vi "COD主界面（列队使用）.vi"() -> (8 "多列列表框":i32(listbox))   [LabVIEW 2016, in "斯坦道CODMn.lvlib"]
uses:
  <vilib>/Analysis/6fits.llb/Curve Fitting Criteria.ctl
  <vilib>/Utility/miscctls.llb/LVPointTypeDef.ctl
  <vilib>/Utility/config.llb/Read Key (I32).vi
  <vilib>/Utility/config.llb/Read Key (Double).vi
  <vilib>/Utility/config.llb/Read Key (Boolean).vi
  <vilib>/Utility/config.llb/Write Key (I32).vi
  <vilib>/Utility/config.llb/Write Key (Double).vi
  <vilib>/Utility/config.llb/Write Key (Boolean).vi
  <vilib>/Waveform/WDTFileIO.llb/Read Waveform from File.vi
  <vilib>/ptbypt/NI_PtbyPt.lvlib
  <vilib>/Utility/config.llb/NI_LVConfig.lvlib
  <vilib>/Analysis/NI_AALPro.lvlib
panel:
  in  "加标回收量程：":enum32{"H", "L", "AUTO"}(ring)=enum."AUTO"
  in  "定时设置":cluster{"启动":bool, "控制命令":T1, "测量参数":T2}(xcontrol)
  out "氢氧化钠":dbl
  in  "序列号变更":bool
  out "模块版本号":string
  in  "更新程序":bool
  out "进样无液体告警":bool
  out "校准内容显示":string
  out "60分钟超时报警":bool
  in  "远程校准量程":enum16{"L", "H"}(ring)
  in  "远程自动校准浓度":dbl
  in  "仪器参数":bool
  out "CODMn序列号":string
  out "CODMn软件版本：":string
  in  "标样核查量程选择":enum32{"H", "L", "AUTO"}(ring)=enum."AUTO"
  in  "标样浓度":dbl
  in  "零点核查量程选择":enum32{"H", "L", "AUTO"}(ring)=enum."AUTO"
  in  "零点核查浓度":dbl
  out "序列号":string
  in  "采水泵排液时间/s:":i32
  in  "采水泵润洗时间/s:":i32
  in  "采水泵沉淀时间/s:":i32
  in  "采水泵进样时间/s:":i32
  in  "常规版/认证版":enum16{"常规版-酸性", "常规版-碱性", "认证版", "浮台版"}(ring)
  in  "释放串口":bool
  in  "打开串口":bool
  in  "保存参数":dbl[](array[numeric])
  out "报警数字":i16
  out "CODMn工作状态":T3(ring)
  out "ORP-K":string
  out "ORP-B":string
  out "ORP-A":string
  out "x = y?":bool
  out "稀释倍数解释":string
  in  "跨度量程选择":enum32{"H", "L", "AUTO"}(ring)=enum."AUTO"
  in  "跨度液浓度":dbl
  in  "水样：":dbl
  in  "蒸馏水：":dbl
  in  "标液：":dbl
  in  "零点核查样：":dbl
  in  "加标回收样：":dbl
  in  "草酸钠":dbl
  in  "高锰酸钾":dbl
  in  "硫酸":dbl
  out "量程解释说明":string
  in  "高切低阈值:":dbl
  in  "低切高阈值:":dbl
  in  "水样量程选择:":enum16{"L", "H", "自动切换测一次", "自动切换测两次"}(ring)
  in  "氢氧化钠：":dbl
  in  "标准液浓度":dbl
  in  "温度":dbl
  in  "恒温时间":dbl
  in  "当前量程：":enum16{"L", "H"}(ring)
  in  "CODMn零点核查选择":enum16{"零点核查走纯水管", "零点核查走零漂管"}(ring)
  in  "锁定按钮":bool
  in  "低量程稀释倍数:":i8=1
  in  "高量程稀释倍数:":i8=2
  in  "一键写入":bool
  in  "测量模式(公式)":u16(ring)=1 items=["水样测试"=1, "标样核查"=2, "零点核查"=3, "跨度核查"=4, "空白测试"=5, "平行样"=6, "加标回收"=7]
  out "基本量程(显示)":string
  out "测量模式(显示)":string
  out "数据时间":string
  out "断电排液标记":bool
  out "COM":string
  in  "启用5":bool
  in  "校准5":bool
  in  "泵滴定数5":dbl
  in  "浓度5":dbl
  in  "启用4":bool
  in  "校准4":bool
  in  "泵滴定数4":dbl
  in  "浓度4":dbl
  out "波形时间":timestamp
  in  "历史波形":bool
  out "滴定数-ORP值":u16[](array[numeric]) caption="数组"
  in  "关闭 3":bool
  in  "滴定曲线":bool
  out "ORP滴定曲线":u16[](graph)
  out "空白测试标记":bool
  out "跨度核查标记":bool
  in  "量程选择":enum16{"低量程", "高量程", "0-2量程"}(ring)
  in  "手动控制":bool
  in  "选用水样":enum16{"葡萄糖", "草酸钠"}(ring)
  in  "方程系数":cluster{"K":dbl, "b":dbl, "X^2":dbl} {"X^2" format="%#.6g"; "b" format="%#.6g"; "K" format="%#.6g"}
  out "多项式系数":dbl[](array[numeric])
  out "XY图":cluster{"X Values":dbl[], "Y Values":dbl[]}[](graph)
  in  "模型":enum32{"线性", "多项式"}(ring)
  out "启动时间":timestamp format="%<%Y/%m/%d %H:%M:%S>T"
  in  "关闭 2":bool
  out "r^2":dbl format="%.8g"
  out "拟合公式":string
  out "b":dbl format="%#.4g"
  out "K":dbl format="%#.4f"
  in  "启用3":bool
  in  "启用2":bool
  in  "启用1":bool
  in  "校准3":bool
  in  "校准2":bool
  in  "校准1":bool
  in  "泵滴定数3":dbl
  in  "泵滴定数2":dbl
  in  "泵滴定数1":dbl
  in  "浓度3":dbl
  in  "浓度2":dbl
  in  "浓度1":dbl
  in  "写入":bool
  out "零点核查标记":bool
  out "排液故障":bool
  out "进水样超量程":bool
  out "标样核查标记":bool
  out "平行样测量":bool
  out "加标回收测量":bool
  out "质控样测量":bool
  out "待机":bool
  out "校标错误":bool
  out "校零错误":bool
  out "测量错误":bool
  out "草酸钠报警":bool
  out "高锰酸钾报警":bool
  out "加热故障":bool
  out "温控器故障":bool
  out "ORP故障":bool
  out "排液标记":bool
  out "故障标记":bool
  out "校标标记":bool
  out "校零标记":bool
  out "通讯状态":bool
  out "水样测量":bool
  in  "读取":bool
  in  "返回":bool
  in  "校准配置":bool
  in  "零点泵计量数 2":dbl
  in  "标度泵计量数 2":dbl
  out "标度滴定值":dbl
  out "零点滴定值":dbl
  in  "保存":bool
  in  "关闭":bool
  out "仪器时间":timestamp format="%<%Y/%m/%d %H:%M:%S>T"
  out "秒":u16
  out "分":u16
  out "COD浓度（mg/L)":dbl format="%.2g"
  out "进样管":dbl
  out "高锰酸钾":dbl
  out "草酸钠":dbl
  out "硫酸":dbl
  out "实时ORP":dbl
  out "温度℃":dbl
  out "加热":bool
  out "搅拌":bool
  out "进硫酸":bool
  out "进加标回收样":bool
  out "进零点核查样":bool
  out "进标液":bool
  out "进蒸馏水":bool
  out "进水样":bool
  out "进草酸钠":bool
  out "进高锰酸钾":bool
  in  "启动":bool
  in  "故障清除":bool
  in  "参数配置":bool
  in  "停止":bool
  in  "单步启动":bool
  out "系统时间":timestamp
  in  "时间校准":bool
  out "模式（受控）":u16
  # "测试时长："
  # "注：遇到加热故障和排液故障时仪器不能正常启动，\n必须排查故障并点击报警清除按钮方可运行。"
  # "mg/L"
  # "基本参数设置"
  # "校零校标结果"
  # "泵计量参数设置"
  # "校零结果："
  # "校零滴定值："
  # "高锰酸钾："
  # "加热恒温温度(℃):"
  # "草酸钠："
  # "校标结果："
  # "标度滴定值："
  # "恒温时间(分钟):"
  # "零点泵计量值："
  # "硫酸："
  # "标准液浓度(mg/L):"
  # "标度泵计量值："
  # "跨度核查浓度："
  # "跨度核查量程："
  # "零点核查浓度："
  # "标样浓度："
  # "零点核查量程："
  # "标样核查量程："
  # "远程校准配置区"
  # "公式读取写入区"
  # "mg/L"
  # "是否启用"
  # "泵滴定数"
  # "浓度"
  # "辅\n助\n计\n算\n区"
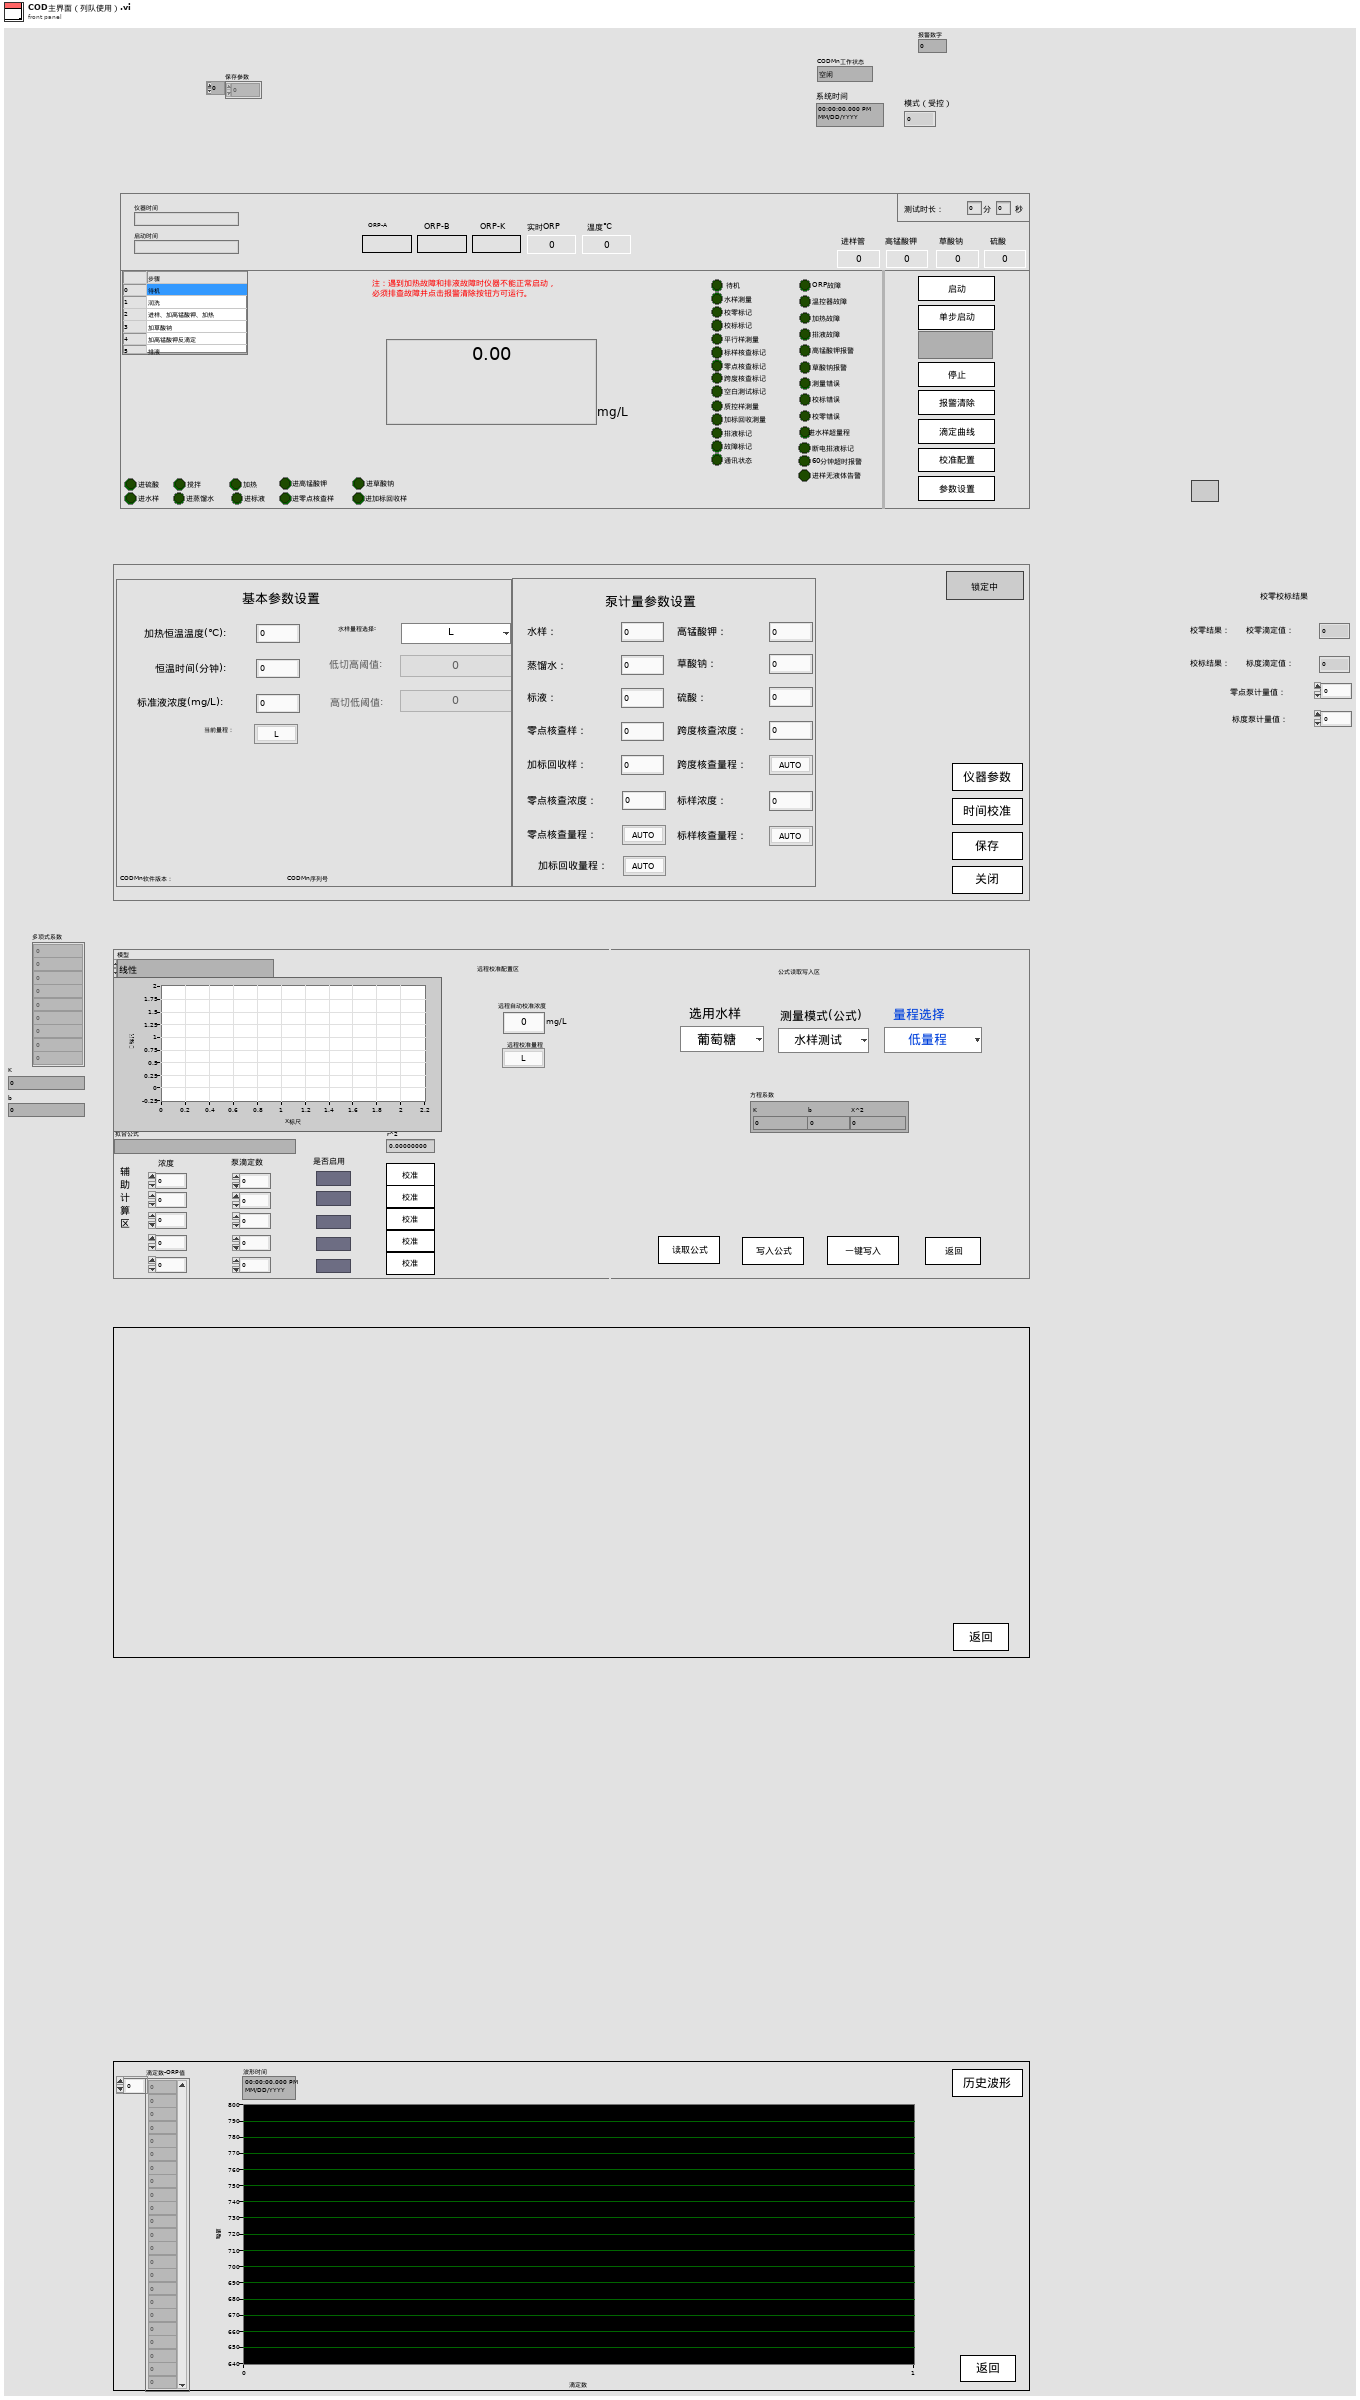
[diagram p1: front panel]
types:
  T1 = typedef "定时设置.xctl/国标控制命令.ctl" = enum16{"启动测量", "标样核查", "零点核查", "跨度核查", "空白测试", "平行样测试", "加标回收", "空白校准", "标样校准", "初始化（清洗）", "停止测试", "仪器重启", "校时", "模式设置", "测量间隔设置"}
  T2 = typedef "定时设置.xctl/测量参数.ctl" = u16
  T3 = enum16{"空闲", "水样测试", "标样核查", "零点核查", "跨度核查", "空白测试", "平行样测试", "质控样", "空白校准", "标样校准", "加标回收"}
  T4 = typedef "LVPointTypeDef.ctl" = cluster{"Horizontal":i16, "Vertical":i16}
  T5 = cluster{"Major":u16, "Minor":u16, "Fix":u16, "Build":u16}
  T6 = typedef "NI_LVConfig.lvlib/Config Data RefNum.ctl" = refnum<k1>
  T7 = cluster{"时间源选择":enum16{"系统时间源", "仪器时间源"}, "外部时间源":timestamp}
  T8 = enum32{"Bad", "Idle", "Run top level", "Running"}
  T9 = enum8{"Enabled", "Disabled", "Disabled and Grayed Out"}
  T10 = cluster{"时间":timestamp, "测量模式":string, "数据类型":string, "检测值":sgl, "单位":string, "数据标识":string, "因子编码":string, "标样参考值":sgl, "ORP-A":sgl, "ORP-B":sgl, "ORP-K":sgl, "COD滴定值":sgl, "高锰酸钾滴定数":sgl, "温度":sgl, "量程":sgl, "LastTime":timestamp, "序列号:":string}
  T11 = cluster{"因子编码":u32, "单位":u16, "标样参考值":sgl, "水样数据时间":timestamp, "水样实测值":sgl, "水样数据标识":string, "标样数据时间":timestamp, "标样实测值":sgl, "标样数据标识":string, "空白数据时间":timestamp, "空白实测值":sgl, "空白数据标识":string, "零点核查数据时间":timestamp, "零点核查实测值":sgl, "零点核查数据标识":string, "跨度核查数据时间":timestamp, "跨度核查实测值":sgl, "跨度核查数据标识":string, "加标回收数据时间":timestamp, "加标回收实测值":sgl, "加标回收数据标识":string, "平行样数据时间":timestamp, "平行样实测值":sgl, "平行样数据标识":string}
  T12 = cluster{"数组 2[0]":sgl, "数组 2[1]":sgl, "数组 2[2]":sgl, "数组 2[3]":sgl, "数组 2[4]":sgl, "数组 2[5]":sgl, "数组 2[6]":sgl, "数组 2[7]":sgl, "数组 2[8]":sgl, "数组 2[9]":sgl, "数组 2[10]":sgl, "数组 2[11]":sgl, "数组 2[12]":sgl, "数组 2[13]":sgl, "数组 2[14]":sgl, "数组 2[15]":sgl, "数组 2[16]":sgl, "数组 2[17]":sgl, "数组 2[18]":sgl, "数组 2[19]":sgl, "数组 2[20]":sgl, "数组 2[21]":sgl, "数组 2[22]":sgl, "数组 2[23]":sgl, "数组 2[24]":sgl, "数组 2[25]":sgl, "数组 2[26]":sgl, "数组 2[27]":sgl, "数组 2[28]":sgl, "数组 2[29]":sgl, "数组 2[30]":sgl, "数组 2[31]":sgl, "数组 2[32]":sgl, "数组 2[33]":sgl, "数组 2[34]":sgl, "数组 2[35]":sgl, "数组 2[36]":sgl, "数组 2[37]":sgl, "数组 2[38]":sgl, "数组 2[39]":sgl, "数组 2[40]":sgl, "数组 2[41]":sgl}
  T13 = cluster{"ORP故障":bool, "温控器故障":bool, "加热故障":bool, "高锰酸钾报警":bool, "草酸钠报警":bool, "测量错误":bool, "校零错误":bool, "校标错误":bool, " 进水样超量程":bool, "排液阀故障":bool, "60分钟超时报警":bool, "进样无液体报警":bool}
  T14 = cluster{"时间标识":timestamp, "参数":string, "日志信息":string, "流程参数":string}
  T15 = cluster{"测量量程":dbl, "测量精度":dbl, "测量间隔":dbl, "消解温度":dbl, "消解时长":dbl, "空白校准时间":timestamp, "曲线截距":dbl, "曲线斜率":dbl, "测量检出限":dbl, "测量信号值":dbl, "线性相关系数":dbl, "二次多项式系数":dbl, "标样校准时间":timestamp, "稀释倍数":dbl, "三项式系数":dbl, "空白标定系数":dbl, "量程系数":dbl, "F0/ORPA":dbl, "F1/ORPB":dbl, "F2/ORPK":dbl, "F3":dbl, "F4":dbl, "F5":dbl, "F6":dbl, "F7":dbl, "X0/滴定数":dbl, "量程":dbl}
  T16 = cluster{"确定":bool, "测量量程":dbl, "测量精度":dbl, "测量间隔":dbl, "消解温度":dbl, "消解时长":dbl, "空白校准时间":timestamp, "曲线截距":dbl, "曲线斜率":dbl, "测量检出限":dbl, "测量信号值":dbl, "线性相关系数":dbl, "二次多项式系数":dbl, "标样校准时间":timestamp, "稀释倍数":dbl, "三项式系数":dbl, "空白标定系数":dbl, "量程系数":dbl, "F0/ORPA":dbl, "F1/ORPB":dbl, "F2/ORPK":dbl, "F3":dbl, "F4":dbl, "F5":dbl, "F6":dbl, "F7":dbl, "X0/滴定数":dbl, "量程":dbl}
  T17 = cluster{"时间标识":timestamp, "设备":string, "日志信息":string, "流程参数":string}
  T18 = typedef "NI_AALPro.lvlib/Curve Fitting Criteria.ctl" = u16
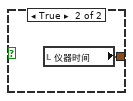
[diagram p2: hidden frame]
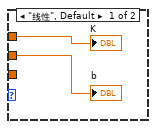
[diagram p8: hidden frame]
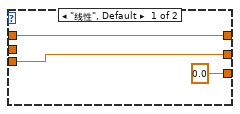
[diagram p10: hidden frame]
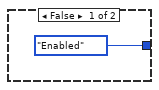
[diagram p11: hidden frame]
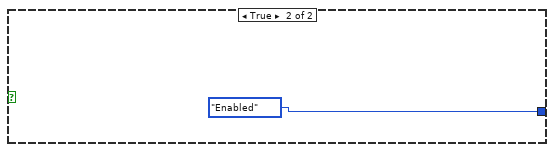
[diagram p12: hidden frame]
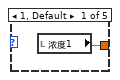
[diagram p17: hidden frame]
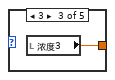
[diagram p18: hidden frame]
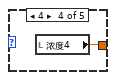
[diagram p19: hidden frame]
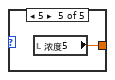
[diagram p20: hidden frame]
diagram:
  n1 = flat-sequence {
    tunnel: w3 -> [_]
    frame #0 {
      w20 = u16 1 items=["水样测试"=1, "标样核查"=2, "零点核查"=3, "跨度核查"=4, "空白测试"=5, "平行样"=6, "加标回收"=7] ("测量模式(公式)")
      n2 = vi-ref "斯坦道CODMn.lvlib:待机状态数据存储写入和切换量程(子VI).vi"() -> (w56:refnum<vi>)
      n3 = vi-ref "斯坦道CODMn.lvlib:日志报警状态存储 (子VI).vi"() -> (w49:refnum<vi>)
      n4 = vi-ref "斯坦道CODMn.lvlib:高锰酸钾-ORP滴定曲线(子VI).vi"() -> (w36:refnum<vi>)
      n5 = property class="VI"(reference=w49, error in=errorcluster {"status"=FALSE, "code"=0, "source"=""} ("错误输出")) -> ("Name"=w48:string)  [unwired: 2 out]
      n6 = property class="VI"(reference=w36, error in=errorcluster {"status"=FALSE, "code"=0, "source"=""} ("错误输出")) -> ("Name"=w37:string)  [unwired: 2 out]
      n7 = property class="VI"(reference=w56, error in=errorcluster {"status"=FALSE, "code"=0, "source"=""} ("错误输出")) -> ("Name"=w55:string)  [unwired: 2 out]
      n8 = Open VI Reference(type specifier VI Refnum (for type only)=refnum<vi> refnum, vi path=w48, options=128 ("选项")) -> (vi reference=w32:refnum<vi>, error out=w46:errorcluster)  [unwired: 3 in]
      n9 = Open VI Reference(type specifier VI Refnum (for type only)=refnum<vi> refnum, vi path=w37, options=128 ("选项")) -> (vi reference=w35:refnum<vi>, error out=w39:errorcluster)  [unwired: 3 in]
      n10 = call-by-ref "?"(reference=w32, error in=w46) -> (reference out=w44:refnum<vi>, error out=w45:errorcluster)  [unwired: 12 in]
      n11 = call-by-ref "?"(reference=w35, error in=w39) -> (reference out=w41:refnum<vi>, error out=w40:errorcluster)  [unwired: 12 in]
      n12 = Open VI Reference(type specifier VI Refnum (for type only)=refnum<vi> refnum, vi path=w55, options=128 ("选项")) -> (vi reference=w30:refnum<vi>, error out=w53:errorcluster)  [unwired: 3 in]
      n13 = Close Reference(reference=w44, error in (no error)=w45) -> ()  [unwired: 1 out]
      n14 = call-by-ref "?"(reference=w30, error in=w53) -> (reference out=w51:refnum<vi>, error out=w52:errorcluster)  [unwired: 12 in]
      n15 = Close Reference(reference=w41, error in (no error)=w40) -> ()  [unwired: 1 out]
      n16 = Close Reference(reference=w51, error in (no error)=w52) -> ()  [unwired: 1 out]
      n17 = vi-ref "关键参数交互.vi"() -> (w27:refnum<vi>)
      n18 = property class="VI"(reference=w27, error in=errorcluster {"status"=FALSE, "code"=0, "source"=""} ("错误输出")) -> ("Name"=w26:string)  [unwired: 2 out]
      n19 = Open VI Reference(type specifier VI Refnum (for type only)=refnum<vi> refnum, vi path=w26, options=128 ("选项")) -> (vi reference=w28:refnum<vi>, error out=w24:errorcluster)  [unwired: 3 in]
      n20 = call-by-ref "?"(reference=w28, error in=w24, "量程选择"=enum16{"低量程", "高量程", "0-2量程"}."低量程", "测量模式(公式)"=w20, "模型"=enum32{"线性", "多项式"}."线性") -> (reference out=w22:refnum<vi>, error out=w23:errorcluster)  [unwired: 9 in]
      n21 = Close Reference(reference=w22, error in (no error)=w23) -> ()  [unwired: 1 out]
    }
  }
  n22 = property on="定时设置" class="定时设置 (严格)"("引用参数"="CODMn") -> (error out=w1:errorcluster)  [unwired: 2 in, 1 out]
  n23 = flat-sequence {
    tunnel: [w59] -> w5
    tunnel: [errorcluster {"status"=FALSE, "code"=0, "source"=""} ("错误输出")] -> w3
    tunnel: [w61] -> w4
    frame #0 {
      w83 = "192.168.1.100" ("名称")
      n24 = global write "COD内部交互全局.vi" "量程切换次数"(u8 0 ("量程切换次数")) -> ()
      n25 = global write "COD内部交互全局.vi" "切换量程连续测两次"(FALSE ("切换量程连续测两次")) -> ()
      n26 = global read "COD内部交互全局.vi" "序列号:"() -> (w90:string)
      n27 = property on="窗格" class="Pane"("Origin"=T4 {"Horizontal"=0, "Vertical"=0} ("原点")) -> ()  [unwired: 2 in, 2 out]
      n28 = Empty String/Path?(string/path=w90) -> (empty?=w58:bool)
      n29 = case shown="真" w58 {
        tunnel: w90 -> [w105 _]
        tunnel: [w104 "data\\CODMnSet.ini" ("名称或相对路径")] -> w71
        frame False {
          # "与生产用上位机交互"
          n30 = Concatenate Strings("data\\" ("字符串"), "序列号" ("字符串"), w105, "Set.ini" ("名称或相对路径")) -> (w104:string)
        }
        frame True {
        }
      }
      n31 = String To IP(1:w83) -> (0:w76:u32)
      n32 = IP To String(2:w76) -> (0:w79:string)  [unwired: 1 in]
      n33 = Not Equal?(x=w83, y=w79) -> (x != y?=w84:bool)
      n34 = Concatenate Strings("\\\\" ("字符串"), w79) -> (w78:string)
      n35 = global write "CODMN外部API.vi" "ping"(w84) -> ()
      n36 = String To Path(string=w78) -> (path=w85:path)
      n37 = Build Path(base path=w85, name or relative path=w71) -> (appended path=w80:path)
      n38 = local write "量程选择"(enum16{"低量程", "高量程", "0-2量程"}."低量程" ("量程选择")) -> ()
      n39 = local write "选用水样"(enum16{"葡萄糖", "草酸钠"}."葡萄糖" ("选用水样")) -> ()
      n40 = global write "COD内部交互全局.vi" "配置文件ini"(w71) -> ()
      n41 = case shown="真" w84 {
        tunnel: w80 -> [w95 w99]
        tunnel: [w95 w98] -> w81
        tunnel: [FALSE w97] -> w82
        frame False {
        }
        frame True {
          n42 = call <vilib>:"Check if File or Folder Exists.vi"("path"=w99) -> ("file or folder exists?"=w97:bool, "dup path"=w98:path)  [unwired: 8 in, 1 out]
        }
      }
      n43 = control-ref of="本VI"() -> (w70:refnum<vi>)
      n44 = case shown="假" w82 {
        tunnel: w81 -> [_ w103]
        tunnel: [w101 w103] -> w62
        tunnel: w71 -> [w100 _]
        frame False {
          # "本地文件地址"
          n45 = call <vilib>:"Application Directory.vi"() -> ("Application Directory"=w102:path)
          n46 = Build Path(base path=w102, name or relative path=w100) -> (appended path=w101:path)
        }
        frame True {
          # "网络共享地址"
        }
      }
      n47 = property class="VI"(reference=w70) -> ("Library.Version"=w69:T5)  [unwired: 1 in, 2 out]
      n48 = Unbundle By Name(w69) -> ("Major"=w67:u16, "Minor"=w66:u16, "Fix"=w65:u16, "Build"=w64:u16)
      n49 = Format Into String(format string="模块版本号：%d.%d.%d.%d" ("格式字符串"), w67, w66, w65, w64) -> (resulting string=→"模块版本号":string)  [unwired: 2 in, 1 out]
      n50 = global write "CODMN外部API.vi" "配置文件 path"(w62) -> ()
      n51 = call <vilib>:"Open Config Data.vi"("configuration file path"=w62) -> ("error out"=w72:errorcluster, "refnum"=w73:T6)  [unwired: 8 in, 1 out]
      n52 = vi-ref "斯坦道CODMn.lvlib:CODMn断电保存全局变量.vi"() -> (w86:refnum<vi>)
      n53 = call <userlib>:"Read Panel from INI__ogtk.vi"("error in (no error)"=w72, "VI ref"=w86, "refnum"=w73) -> ("error out"=w74:errorcluster, "refnum out"=w75:T6)  [unwired: 7 in]
      n54 = call <vilib>:"Close Config Data.vi"("error in (no error)"=w74, "refnum"=w75) -> ("error out"=w60:errorcluster)  [unwired: 8 in, 1 out]
      n55 = call <vilib>:"Clear Errors.vi"("error in (no error)"=w60) -> ("error out"=w57:errorcluster)  [unwired: 5 in, 1 out]
      n56 = Read from Text File(file (use dialog)=w62, error in=w57) -> (text=w61:string, error out=w59:errorcluster)  [unwired: 2 in, 2 out]
      "稀释倍数解释" <- "稀释倍数解释：\n稀释倍数选择1，表示不稀释\n默认低量程系数倍数1，高量程系数倍数2\n则低量程为0~8，高量程为0~16" ("稀释倍数解释")
    }
  }
  n57 = while {
    tunnel: w1 -> [_]
    stop <- FALSE stop-if-true
    n58 = Wait (ms)(milliseconds to wait=u32 500 ("等待时间（毫秒）")) -> ()  [unwired: 1 out]
    n59 = global read "COD测量模式全局.vi" "CODMn工作状态"() -> (w116:T3)
    n60 = local read "通讯状态"() -> (w110:bool)
    n61 = case shown="假" w110 {
      tunnel: [w126 w127] -> w114
      frame False {
        n62 = Get Date/Time In Seconds() -> (seconds since 1Jan1904=w126:timestamp)
      }
      frame True {
        n63 = local read "仪器时间"() -> (w127:timestamp)
      }
    }
    n64 = vi-ref "CODMn测量流程.vi"() -> (w123:refnum<vi>)
    n65 = Bundle By Name(cluster=T7 {"时间源选择"=enum."系统时间源", "外部时间源"=timestamp(0 s since 1904-01-01)} ("时间源"), "时间源选择"=enum16{"系统时间源", "仪器时间源"}."仪器时间源", "外部时间源"=w114) -> (w112:T7)
    n66 = property class="VI"(reference=w123) -> ("Exec.State"=w121:T8, "Name"=w122:string)  [unwired: 1 in, 2 out]
    n67 = Not Equal?(x=w116, y=T3."空闲") -> (x != y?=w111:bool)
    n68 = property on="定时设置" class="定时设置 (严格)"("仪器状态"=w111, "时间源"=w112) -> ()  [unwired: 2 in, 2 out]
    n69 = Unbundle By Name("定时设置") -> ("启动"=w119:bool, "控制命令"=w120:T1)
    n70 = case shown="真" w119 {
      tunnel: w122 -> [_ w130]
      tunnel: w120 -> [_ w129]
      tunnel: w121 -> [_ w128]
      frame False {
      }
      frame True {
        n71 = case shown="\"Idle\"" w128 {
          tunnel: w130 -> [_ w134]
          tunnel: w129 -> [_ w131]
          frame "Bad", Default {
          }
          frame "Idle" {
            n72 = Open VI Reference(type specifier VI Refnum (for type only)=refnum<vi> refnum, vi path=w134, options=128 ("选项")) -> (vi reference=w135:refnum<vi>, error out=w136:errorcluster)  [unwired: 3 in]
            n73 = call-by-ref "开始异步调用"(reference=w135, error in=w136, "控制命令"=w131) -> (reference out=w137:refnum<vi>, error out=w138:errorcluster)  [unwired: 11 in]
            n74 = Close Reference(reference=w137, error in (no error)=w138) -> ()  [unwired: 1 out]
          }
        }
      }
    }
  }
  n75 = Obtain Queue(name (unnamed)="CODMn" ("名称（未命名）"), element data type=cluster{"命令":string} {"命令"="启用模块"} ("元素")) -> (queue out=w15:refnum<queue>, error out=w14:errorcluster)  [unwired: 3 in, 1 out]
  n76 = while {
    tunnel: [w145] -> _
    shift-right: [w143] -> _
    shift-left: w4 -> [w142]
    tunnel: w5 -> [_]
    stop <- FALSE stop-if-true
    n77 = global read "CODMN外部API.vi" "配置文件 path"() -> (w139:path)
    n78 = Wait (ms)(milliseconds to wait=u32 1000 ("等待时间（毫秒）")) -> ()  [unwired: 1 out]
    n79 = Read from Text File(file (use dialog)=w139) -> (text=w143:string, error out=w140:errorcluster)  [unwired: 3 in, 2 out]
    n80 = Not Equal?(x=w143, y=w142) -> (x != y?=w141:bool)
    n81 = case shown="真" w141 {
      tunnel: [w147 w154] -> w145
      tunnel: w139 -> [_ w148]
      tunnel: w140 -> [w147 _]
      frame False {
      }
      frame True {
        # "文件发生改变进行更新，远端和本地都更新"
        n82 = vi-ref "斯坦道CODMn.lvlib:CODMn断电保存全局变量.vi"() -> (w149:refnum<vi>)
        n83 = call <vilib>:"Open Config Data.vi"("configuration file path"=w148) -> ("error out"=w153:errorcluster, "refnum"=w152:T6)  [unwired: 8 in, 1 out]
        n84 = call <userlib>:"Read Panel from INI__ogtk.vi"("error in (no error)"=w153, "VI ref"=w149, "refnum"=w152) -> ("error out"=w151:errorcluster, "refnum out"=w150:T6)  [unwired: 7 in]
        n85 = call <vilib>:"Close Config Data.vi"("error in (no error)"=w151, "refnum"=w150) -> ("error out"=w154:errorcluster)  [unwired: 8 in, 1 out]
      }
    }
  }
  n86 = vi-ref "CODMn通讯.vi"() -> (w6:refnum<vi>)
  n87 = while {
    tunnel: w5 -> [_]
    stop <- FALSE stop-if-true
    # "赋值循环"
    n88 = flat-sequence {
      frame #0 {
        # "测量数据区"
        n89 = global read "COD内部交互全局.vi" "data"() -> (w399:T10)
        n90 = global read "COD测量模式全局.vi" "测量模式文字实时"() -> (w385:string)
        "测量模式(显示)" <- w385
        n91 = global read "CODMn断电保存全局变量.vi" "测量数据区"() -> (w394:T11)
        n92 = Unbundle By Name(w399) -> ("时间"=w398:timestamp, "检测值"=w397:sgl, "数据标识"=w396:string)
        n93 = case shown="\"水样测试\"" w385 {
          tunnel: w394 -> [w400 w405 w410 w415 w420 w425 w430 w435 w440 w445]
          tunnel: [w400 w404 w409 w411 w419 w424 w429 w434 w436 w444] -> w395
          tunnel: w398 -> [_ w403 w408 w414 w418 w423 w428 w433 w439 w443]
          tunnel: w397 -> [_ w402 w407 w413 w417 w422 w427 w432 w438 w442]
          tunnel: w396 -> [_ w401 w406 w412 w416 w421 w426 w431 w437 w441]
          frame "", Default {
          }
          frame "水样测试" {
            n94 = Bundle By Name(cluster=w405, "水样数据时间"=w403, "水样实测值"=w402, "水样数据标识"=w401) -> (w404:T11)
          }
          frame "标样核查" {
            n95 = Bundle By Name(cluster=w410, "标样数据时间"=w408, "标样实测值"=w407, "标样数据标识"=w406) -> (w409:T11)
          }
          frame "跨度核查" {
            n96 = Bundle By Name(cluster=w415, "跨度核查数据时间"=w414, "跨度核查实测值"=w413, "跨度核查数据标识"=w412) -> (w411:T11)
          }
          frame "零点核查" {
            n97 = Bundle By Name(cluster=w420, "零点核查数据时间"=w418, "零点核查实测值"=w417, "零点核查数据标识"=w416) -> (w419:T11)
          }
          frame "空白测试" {
            n98 = Bundle By Name(cluster=w425, "空白数据时间"=w423, "空白实测值"=w422, "空白数据标识"=w421) -> (w424:T11)
          }
          frame "加标回收" {
            n99 = Bundle By Name(cluster=w430, "加标回收数据时间"=w428, "加标回收实测值"=w427, "加标回收数据标识"=w426) -> (w429:T11)
          }
          frame "平行样" {
            n100 = Bundle By Name(cluster=w435, "平行样数据时间"=w433, "平行样实测值"=w432, "平行样数据标识"=w431) -> (w434:T11)
          }
          frame "校零" {
            n101 = Bundle By Name(cluster=w440, "空白数据时间"=w439, "空白实测值"=w438, "空白数据标识"=w437) -> (w436:T11)
          }
          frame "校标" {
            n102 = Bundle By Name(cluster=w445, "标样数据时间"=w443, "标样实测值"=w442, "标样数据标识"=w441) -> (w444:T11)
          }
        }
        n103 = Unbundle By Name(w394) -> ("水样实测值"=w391:sgl)
        n104 = feedback-in #1(w394) -> ()
        n105 = feedback #1(w394) -> (w393:T11)
        n106 = global read "CODMn断电保存全局变量.vi" "水样测试量程"() -> (w387:enum16{"L", "H"})
        n107 = Unbundle By Name(w393) -> ("水样实测值"=w392:sgl)
        n108 = feedback #2(w387) -> (w388:enum16{"L", "H"})
        n109 = feedback-in #2(w387) -> ()
        n110 = Not Equal?(x=w388, y=w387) -> (x != y?=w386:bool)
        n111 = Not Equal?(x=w391, y=w392) -> (x != y?=w390:bool)
        n112 = global write "CODMn断电保存全局变量.vi" "测量数据区"(w395) -> ()
        n113 = Or(x=w390, y=w386) -> (x .or. y?=w389:bool)
        n114 = case shown="真" w389 {
          frame False {
          }
          frame True {
            # "水样值发送改变存储本地"
            n115 = call "配置文件保存.vi"() -> ()  [unwired: 12 in]
          }
        }
      }
    }
    n116 = flat-sequence {
      frame #0 {
        # "局部变量给内部交互用全局变量"
        n117 = local read "COD浓度（mg/L)"() -> (w187:dbl)
        n118 = local read "CODMn工作状态"() -> (w190:T3)
        n119 = local read "多列列表框"() -> (w188:i32)
        n120 = local read "标准液浓度"() -> (w186:dbl)
        n121 = local read "温度℃"() -> (w181:dbl)
        n122 = local read "高锰酸钾报警"() -> (w184:bool)
        n123 = local read "断电排液标记"() -> (w183:bool)
        n124 = local read "实时ORP"() -> (w180:dbl)
        n125 = local read "故障标记"() -> (w189:bool)
        n126 = local read "高锰酸钾"() -> (w182:dbl)
        n127 = local read "待机"() -> (w185:bool)
        n128 = global write "COD内部交互全局.vi" "实时温度"(w181) -> ()
        n129 = global write "运行时序全局变量.vi" "多列列表框"(w188) -> ()
        n130 = global write "COD内部交互全局.vi" "故障标记"(w189) -> ()
        n131 = global write "COD内部交互全局.vi" "ORP显示"(w180) -> ()
        n132 = global write "COD浓度全局变量.vi" "标准液浓度"(w186) -> ()
        n133 = global write "COD内部交互全局.vi" "高锰酸钾"(w182) -> ()
        n134 = global write "COD内部交互全局.vi" "待机"(w185) -> ()
        n135 = global write "COD测量模式全局.vi" "CODMn工作状态"(w190) -> ()
        n136 = global write "COD内部交互全局.vi" "高锰酸钾报警"(w184) -> ()
        n137 = global write "COD内部交互全局.vi" "断电排液标记"(w183) -> ()
        n138 = global write "COD浓度全局变量.vi" "COD浓度（mg/L)"(w187) -> ()
      }
    }
    n139 = flat-sequence {
      frame #0 {
        # "断电保存全局给局部变量"
        n140 = global read "CODMn断电保存全局变量.vi" "高切低阈值:"() -> (w459:dbl)
        n141 = global read "CODMn断电保存全局变量.vi" "低切高阈值:"() -> (w458:dbl)
        n142 = global read "CODMn断电保存全局变量.vi" "跨度液浓度"() -> (w456:dbl)
        n143 = global read "COD内部交互全局.vi" "波形时间"() -> (→"波形时间":timestamp)
        n144 = global read "CODMn断电保存全局变量.vi" "启动时间"() -> (→"启动时间":timestamp)
        n145 = global read "CODMn断电保存全局变量.vi" "标样浓度"() -> (w454:dbl)
        n146 = global read "CODMn断电保存全局变量.vi" "CODMn跨度量程选择"() -> (w460:enum32{"H", "L", "AUTO"})
        n147 = global read "CODMn断电保存全局变量.vi" "标样核查量程选择"() -> (w451:enum32{"H", "L", "AUTO"})
        n148 = global read "CODMn断电保存全局变量.vi" "零点核查量程选择"() -> (w453:enum32{"H", "L", "AUTO"})
        n149 = global read "CODMn断电保存全局变量.vi" "加标回收量程选择"() -> (w446:enum32{"H", "L", "AUTO"})
        n150 = global read "COD内部交互全局.vi" "滴定数-ORP值"() -> (→"滴定数-ORP值":u16[])
        n151 = global read "CODMn断电保存全局变量.vi" "常规版/认证版"() -> (w455:enum16{"常规版-酸性", "常规版-碱性", "认证版", "浮台版"})
        n152 = global read "CODMn断电保存全局变量.vi" "自动切换量程:"() -> (w457:enum16{"L", "H", "自动切换测一次", "自动切换测两次"})
        n153 = global read "CODMn断电保存全局变量.vi" "零点核查浓度"() -> (w452:dbl)
        n154 = global read "CODMn断电保存全局变量.vi" "测量模式(公式)"() -> (w461:u16)
        n155 = global read "COD内部交互全局.vi" "ORP滴定曲线"() -> (→"ORP滴定曲线":u16[])
        n156 = local write "高切低阈值:"(w459) -> ()
        n157 = local write "跨度液浓度"(w456) -> ()
        n158 = local write "低切高阈值:"(w458) -> ()
        n159 = local write "标样浓度"(w454) -> ()
        n160 = local write "标样核查量程选择"(w451) -> ()
        n161 = local write "水样量程选择:"(w457) -> ()
        n162 = local write "常规版/认证版"(w455) -> ()
        n163 = local write "零点核查浓度"(w452) -> ()
        n164 = local write "零点核查量程选择"(w453) -> ()
        n165 = local write "加标回收量程："(w446) -> ()
        n166 = local write "测量模式(公式)"(w461) -> ()
        n167 = local write "跨度量程选择"(w460) -> ()
      }
    }
    n168 = flat-sequence {
      frame #0 {
        # "保存参数赋值"
        n169 = Multiply(x="温度", y=10.0) -> (x*y=w165:dbl)
        n170 = Multiply(x="标准液浓度", y=100.0) -> (x*y=w162:dbl)
        n171 = Build Array(w165, "恒温时间", w162, "氢氧化钠：", "当前量程：", "水样：", "蒸馏水：", "标液：", "零点核查样：", "加标回收样：", "高锰酸钾", "草酸钠", "硫酸", "零点泵计量数 2", "标度泵计量数 2", "高量程稀释倍数:", "低量程稀释倍数:", "CODMn零点核查选择") -> (w159:dbl[])
        n172 = local write "保存参数"(w159) -> ()
      }
    }
    n173 = flat-sequence {
      frame #0 {
        # "显示量程说明"
        n174 = global read "COD内部交互全局.vi" "通讯状态"() -> (→"通讯状态":bool)
        n175 = global read "CODMn断电保存全局变量.vi" "MB通信方式选择"() -> (w462:enum16{"串口", "TCP"})
        n176 = local read "低量程稀释倍数:"() -> (w476:i8)
        n177 = local read "高量程稀释倍数:"() -> (w466:i8)
        n178 = case shown="\"TCP\"" w462 {
          tunnel: [w479 w480] -> w467
          frame "串口", Default {
            n179 = global read "CODMn断电保存全局变量.vi" "VISA resource name"() -> (w479:refnum<visa-resource-name>)
          }
          frame "TCP" {
            n180 = global read "CODMn断电保存全局变量.vi" "IP"() -> (w480:string)
          }
        }
        "COM" <- w467
        n181 = Multiply(x=w476, y=i8 8) -> (x*y=w468:i8)
        n182 = Multiply(x=w466, y=i8 8) -> (x*y=w464:i8)
        n183 = Number To Decimal String(number=w468) -> (decimal integer string=w473:string)  [unwired: 1 in]
        n184 = Number To Decimal String(number=w464) -> (decimal integer string=w471:string)  [unwired: 1 in]
        n185 = Concatenate Strings("L低量程范围:0~" ("量程解释说明"), w473, "(mg/L)\n\nH高量程范围:" ("量程解释说明"), "0" ("字符串"), "~" ("量程解释说明"), w471, "(mg/L)" ("量程解释说明")) -> (→"量程解释说明":string)
      }
    }
    n186 = flat-sequence {
      frame #0 {
        # "参数赋值（只在读取参数时候改变一次）"
        n187 = global read "COD内部交互全局.vi" "读取浮台参数显示"() -> (w192:bool)
        n188 = global read "COD内部交互全局.vi" "读取浮台参数"() -> (w191:u16[])
        n189 = global read "COD内部交互全局.vi" "读取参数显示"() -> (w193:bool)
        n190 = global read "COD内部交互全局.vi" "读取参数"() -> (w194:u16[])
        n191 = case shown="真" w192 {
          tunnel: w191 -> [_ w200]
          frame False {
          }
          frame True {
            n192 = Index Array(array=w200) -> (element #1=w199:u16, element #2=w198:u16, element #3=w197:u16, element #4=w196:u16)  [unwired: 4 in]
            n193 = global write "COD内部交互全局.vi" "读取浮台参数显示"(FALSE ("读取参数显示")) -> ()
            n194 = local write "采水泵进样时间/s:"(w199) -> ()
            n195 = local write "采水泵润洗时间/s:"(w198) -> ()
            n196 = local write "采水泵沉淀时间/s:"(w197) -> ()
            n197 = local write "采水泵排液时间/s:"(w196) -> ()
          }
        }
        n198 = case shown="真" w193 {
          tunnel: w194 -> [_ w218]
          frame False {
          }
          frame True {
            n199 = Index Array(array=w218) -> (element #1=w227:u16, element #2=w239:u16, element #3=w223:u16, element #4=w201:u16, element #5=w226:u16, element #6=w225:u16, element #7=w238:u16, element #8=w237:u16, element #9=w236:u16, element #10=w235:u16, element #11=w234:u16, element #12=w233:u16, element #13=w232:u16, element #14=w231:u16, element #15=w230:u16, element #16=w221:u16, element #17=w220:u16, element #18=w219:u16, element #19=w216:u16, element #20=w215:u16, element #21=w214:u16, element #22=w213:u16, element #23=w212:u16, element #27=w208:u16, element #28=w207:u16, element #29=w206:u16, element #30=w205:u16, element #31=w204:u16)  [unwired: 31 in, 3 out]
            n200 = global write "COD内部交互全局.vi" "读取参数显示"(FALSE ("读取参数显示")) -> ()
            n201 = local write "水样："(w225) -> ()
            n202 = local write "标液："(w237) -> ()
            n203 = local write "硫酸"(w232) -> ()
            n204 = local write "零点核查样："(w236) -> ()
            n205 = local write "加标回收样："(w235) -> ()
            n206 = local write "当前量程："(w226) -> ()
            n207 = local write "蒸馏水："(w238) -> ()
            n208 = local write "恒温时间"(w239) -> ()
            n209 = local write "高锰酸钾"(w234) -> ()
            n210 = local write "草酸钠"(w233) -> ()
            n211 = local write "零点泵计量数 2"(w231) -> ()
            n212 = local write "标度泵计量数 2"(w230) -> ()
            n213 = local write "高量程稀释倍数:"(w221) -> ()
            n214 = local write "低量程稀释倍数:"(w220) -> ()
            n215 = local write "CODMn零点核查选择"(w219) -> ()
            n216 = Build Array(w216, w215, w214, w213, w212) -> (w211:u16[])
            n217 = Build Array(w208, w207, w206, w205, w204) -> (w203:u16[])
            n218 = Divide(x=w227, y=u16 10) -> (x/y=w228:dbl)
            n219 = Divide(x=w223, y=u16 100) -> (x/y=w222:dbl)
            n220 = local write "氢氧化钠："(w201) -> ()
            n221 = local write "温度"(w228) -> ()
            n222 = local write "标准液浓度"(w222) -> ()
            n223 = call "HexToString.vi"("数组"=w203) -> ("字符串"=w202:string)  [unwired: 10 in]
            "CODMn序列号" <- w202
            "序列号" <- w202
            n224 = call "FATEK_HexToString.vi"("数组"=w211) -> ("STRING"=w210:string[])  [unwired: 10 in]
            n225 = Index Array(array=w210) -> (element=→"CODMn软件版本：":string)  [unwired: 1 in]
            n226 = global write "COD内部交互全局.vi" "序列号:"(w202) -> ()
          }
        }
      }
    }
    n227 = flat-sequence {
      frame #0 {
        # "权限隐藏和显示功能"
        n228 = local read "x = y?"() -> (w482:bool)
        n229 = property on="更新程序" class="Bool (严格)"("Visible"=w482) -> ()  [unwired: 2 in, 2 out]
        n230 = property on="释放串口" class="Bool"("Visible"=w482) -> ()  [unwired: 2 in, 2 out]
        n231 = property on="打开串口" class="Bool"("Visible"=w482) -> ()  [unwired: 2 in, 2 out]
        n232 = property on="序列号变更" class="Bool"("Visible"=w482) -> ()  [unwired: 2 in, 2 out]
        n233 = property on="常规版/认证版" class="Enum (严格)"("Visible"=w482) -> ()  [unwired: 2 in, 2 out]
        n234 = property on="CODMn零点核查选择" class="Enum (严格)"("Visible"=w482) -> ()  [unwired: 2 in, 2 out]
        n235 = property on="低量程稀释倍数:" class="DigNum (严格)"("Visible"=w482) -> ()  [unwired: 2 in, 2 out]
        n236 = property on="稀释倍数解释" class="Str"("Visible"=w482) -> ()  [unwired: 2 in, 2 out]
        n237 = property on="高量程稀释倍数:" class="DigNum (严格)"("Visible"=w482) -> ()  [unwired: 2 in, 2 out]
        n238 = local read "常规版/认证版"() -> (w497:enum16{"常规版-酸性", "常规版-碱性", "认证版", "浮台版"})
        n239 = case shown="\"浮台版\"" w497 {
          tunnel: [T9."Enabled" ("禁用") T9."Enabled" ("禁用") T9."Disabled and Grayed Out" ("禁用") T9."Enabled" ("禁用")] -> w496
          tunnel: [i32[] [2] ("禁用项[]") i32[] [2] ("禁用项[]") i32[] [] ("禁用项[]") i32[] [2] ("禁用项[]")] -> w495
          tunnel: [w506 w511 T9."Disabled and Grayed Out" ("禁用") w522] -> w494
          tunnel: [w505 FALSE FALSE TRUE] -> w493
          tunnel: [w506 w511 T9."Disabled and Grayed Out" ("禁用") w522] -> w483
          tunnel: [w505 TRUE FALSE FALSE] -> w481
          frame "常规版-酸性", Default {
            w505 = FALSE
            w506 = T9."Enabled" ("禁用")
          }
          frame "常规版-碱性" {
            w511 = T9."Enabled" ("禁用")
          }
          frame "认证版" {
            w517 = u16 1 items=["水样测试"=1, "标样核查"=2, "零点核查"=3, "跨度核查"=4, "空白测试"=5, "平行样"=6, "加标回收"=7] ("测量模式(公式)")
            n240 = global write "CODMn断电保存全局变量.vi" "测量模式(公式)"(w517) -> ()
          }
          frame "浮台版" {
            w522 = T9."Enabled" ("禁用")
          }
        }
        n241 = control-ref of="水样："() -> (w492:refnum<vi>)
        n242 = control-ref of="蒸馏水："() -> (w491:refnum<vi>)
        n243 = control-ref of="标液："() -> (w490:refnum<vi>)
        n244 = control-ref of="零点核查样："() -> (w489:refnum<vi>)
        n245 = control-ref of="加标回收样："() -> (w488:refnum<vi>)
        n246 = local read "水样量程选择:"() -> (w499:enum16{"L", "H", "自动切换测一次", "自动切换测两次"})
        n247 = control-ref of="量程解释说明"() -> (w486:refnum<vi>)
        n248 = control-ref of="氢氧化钠："() -> (w487:refnum<vi>)
        n249 = Not Equal To 0?(x=w499) -> (x != 0?=w498:bool)
        n250 = control-ref of="进样管"() -> (w484:refnum<vi>)
        n251 = Build Array(w492, w491, w490, w489, w488, w486, w487, w484) -> (w485:refnum<vi>[])
        n252 = Select(t=T9."Enabled" ("禁用"), s=w498, f=T9."Disabled and Grayed Out" ("禁用")) -> (s? t:f=w500:T9)
        n253 = for {
          tunnel: w485 -> [w504] mode=indexing
          tunnel: w483 -> [w503]
          n254 = property class="Ctl"(reference=w504, "DisabledEnum"=w503) -> ()  [unwired: 1 in, 2 out]
        }
        n255 = property on="低切高阈值:" class="DigNum (严格)"("DisabledEnum"=w500) -> ()  [unwired: 2 in, 2 out]
        n256 = property on="高切低阈值:" class="DigNum (严格)"("DisabledEnum"=w500) -> ()  [unwired: 2 in, 2 out]
        n257 = property on="采水泵润洗时间/s:" class="DigNum (严格)"("Visible"=w493) -> ()  [unwired: 2 in, 2 out]
        n258 = property on="采水泵沉淀时间/s:" class="DigNum (严格)"("Visible"=w493) -> ()  [unwired: 2 in, 2 out]
        n259 = property on="采水泵排液时间/s:" class="DigNum (严格)"("Visible"=w493) -> ()  [unwired: 2 in, 2 out]
        n260 = property on="采水泵进样时间/s:" class="DigNum (严格)"("Visible"=w493) -> ()  [unwired: 2 in, 2 out]
        n261 = property on="一键写入" class="Bool (严格)"("DisabledEnum"=w494) -> ()  [unwired: 2 in, 2 out]
        n262 = property on="量程选择" class="Enum (严格)"("Disabled Items []"=w495) -> ()  [unwired: 2 in, 2 out]
        n263 = property on="测量模式(公式)" class="Ring (严格)"("DisabledEnum"=w496) -> ()  [unwired: 2 in, 2 out]
        n264 = property on="氢氧化钠：" class="DigNum (严格)"("Visible"=w481) -> ()  [unwired: 2 in, 2 out]
        n265 = property on="氢氧化钠" class="DigNum (严格)"("Visible"=w481) -> ()  [unwired: 2 in, 2 out]
      }
    }
    n266 = flat-sequence {
      frame #0 {
        # "公式读取显示（只在读取公式的时候改变一次）"
        n267 = global read "COD内部交互全局.vi" "读取公式显示"() -> (w240:bool)
        n268 = case shown="真" w240 {
          frame False {
          }
          frame True {
            n269 = global write "COD内部交互全局.vi" "读取公式显示"(FALSE ("读取参数显示")) -> ()
            n270 = global read "COD内部交互全局.vi" "读取公式"() -> (w250:u16[])
            n271 = Array Subset(array=w250, index=10 ("索引"), length=84 ("长度")) -> (w245:u16[])
            n272 = One Button Dialog(message="公式读取成功！" ("消息")) -> ()  [unwired: 1 in, 1 out]
            n273 = local read "测量模式(公式)"() -> (w248:u16)
            n274 = call "浮点CDAB转换COD.vi"("数组"=w245) -> ("数组 2"=w246:sgl[])  [unwired: 10 in]
            n275 = Array To Cluster(array=w246) -> (cluster=w249:T12)
            n276 = case shown="6" w248 {
              tunnel: [cluster{"X":dbl, "b":dbl, "X^2":dbl} {"X"=999.0, "b"=999.0, "X^2"=999.0} ("方程系数") w253 w272 w291 w310 w329 w348 w367] -> w247
              tunnel: w249 -> [_ w252 w271 w290 w309 w328 w347 w366]
              frame 0, Default {
              }
              frame 1 {
                n277 = local read "量程选择"() -> (w255:enum16{"低量程", "高量程", "0-2量程"})
                n278 = case shown="\"低量程\", 默认" w255 {
                  tunnel: w252 -> [w262 w266 w270]
                  tunnel: [w261 w265 w269] -> w258
                  tunnel: [w260 w264 w268] -> w257
                  tunnel: [w259 w263 w267] -> w256
                  frame "低量程", Default {
                    n279 = Unbundle By Name(w262) -> ("数组 2[0]"=w261:sgl, "数组 2[1]"=w260:sgl, "数组 2[2]"=w259:sgl)
                  }
                  frame "高量程" {
                    n280 = Unbundle By Name(w266) -> ("数组 2[3]"=w265:sgl, "数组 2[4]"=w264:sgl, "数组 2[5]"=w263:sgl)
                  }
                  frame "0-2量程" {
                    n281 = Unbundle By Name(w270) -> ("数组 2[6]"=w269:sgl, "数组 2[7]"=w268:sgl, "数组 2[8]"=w267:sgl)
                  }
                }
                n282 = Bundle By Name(cluster=cluster{"X":dbl, "b":dbl, "X^2":dbl} {"X"=0.0, "b"=0.0, "X^2"=0.0} ("方程系数"), "X"=w258, "b"=w257, "X^2"=w256) -> (w253:cluster{"X":dbl, "b":dbl, "X^2":dbl})
              }
              frame 2 {
                n283 = local read "量程选择"() -> (w274:enum16{"低量程", "高量程", "0-2量程"})
                n284 = case shown="\"高量程\"" w274 {
                  tunnel: w271 -> [w281 w285 w289]
                  tunnel: [w280 w284 w288] -> w277
                  tunnel: [w279 w283 w287] -> w276
                  tunnel: [w278 w282 w286] -> w275
                  frame "低量程", Default {
                    n285 = Unbundle By Name(w281) -> ("数组 2[6]"=w280:sgl, "数组 2[7]"=w279:sgl, "数组 2[8]"=w278:sgl)
                  }
                  frame "高量程" {
                    n286 = Unbundle By Name(w285) -> ("数组 2[9]"=w284:sgl, "数组 2[10]"=w283:sgl, "数组 2[11]"=w282:sgl)
                  }
                  frame "0-2量程" {
                    n287 = Unbundle By Name(w289) -> ("数组 2[6]"=w288:sgl, "数组 2[7]"=w287:sgl, "数组 2[8]"=w286:sgl)
                  }
                }
                n288 = Bundle By Name(cluster=cluster{"X":dbl, "b":dbl, "X^2":dbl} {"X"=0.0, "b"=0.0, "X^2"=0.0} ("方程系数"), "X"=w277, "b"=w276, "X^2"=w275) -> (w272:cluster{"X":dbl, "b":dbl, "X^2":dbl})
              }
              frame 3 {
                n289 = local read "量程选择"() -> (w293:enum16{"低量程", "高量程", "0-2量程"})
                n290 = case shown="\"高量程\"" w293 {
                  tunnel: w290 -> [w300 w304 w308]
                  tunnel: [w299 w303 w307] -> w296
                  tunnel: [w298 w302 w306] -> w295
                  tunnel: [w297 w301 w305] -> w294
                  frame "低量程", Default {
                    n291 = Unbundle By Name(w300) -> ("数组 2[12]"=w299:sgl, "数组 2[13]"=w298:sgl, "数组 2[14]"=w297:sgl)
                  }
                  frame "高量程" {
                    n292 = Unbundle By Name(w304) -> ("数组 2[15]"=w303:sgl, "数组 2[16]"=w302:sgl, "数组 2[17]"=w301:sgl)
                  }
                  frame "0-2量程" {
                    n293 = Unbundle By Name(w308) -> ("数组 2[6]"=w307:sgl, "数组 2[7]"=w306:sgl, "数组 2[8]"=w305:sgl)
                  }
                }
                n294 = Bundle By Name(cluster=cluster{"X":dbl, "b":dbl, "X^2":dbl} {"X"=0.0, "b"=0.0, "X^2"=0.0} ("方程系数"), "X"=w296, "b"=w295, "X^2"=w294) -> (w291:cluster{"X":dbl, "b":dbl, "X^2":dbl})
              }
              frame 4 {
                n295 = local read "量程选择"() -> (w312:enum16{"低量程", "高量程", "0-2量程"})
                n296 = case shown="\"高量程\"" w312 {
                  tunnel: w309 -> [w319 w323 w327]
                  tunnel: [w318 w322 w326] -> w315
                  tunnel: [w317 w321 w325] -> w314
                  tunnel: [w316 w320 w324] -> w313
                  frame "低量程", Default {
                    n297 = Unbundle By Name(w319) -> ("数组 2[18]"=w318:sgl, "数组 2[19]"=w317:sgl, "数组 2[20]"=w316:sgl)
                  }
                  frame "高量程" {
                    n298 = Unbundle By Name(w323) -> ("数组 2[21]"=w322:sgl, "数组 2[22]"=w321:sgl, "数组 2[23]"=w320:sgl)
                  }
                  frame "0-2量程" {
                    n299 = Unbundle By Name(w327) -> ("数组 2[6]"=w326:sgl, "数组 2[7]"=w325:sgl, "数组 2[8]"=w324:sgl)
                  }
                }
                n300 = Bundle By Name(cluster=cluster{"X":dbl, "b":dbl, "X^2":dbl} {"X"=0.0, "b"=0.0, "X^2"=0.0} ("方程系数"), "X"=w315, "b"=w314, "X^2"=w313) -> (w310:cluster{"X":dbl, "b":dbl, "X^2":dbl})
              }
              frame 5 {
                n301 = local read "量程选择"() -> (w331:enum16{"低量程", "高量程", "0-2量程"})
                n302 = case shown="\"高量程\"" w331 {
                  tunnel: w328 -> [w338 w342 w346]
                  tunnel: [w337 w341 w345] -> w334
                  tunnel: [w336 w340 w344] -> w333
                  tunnel: [w335 w339 w343] -> w332
                  frame "低量程", Default {
                    n303 = Unbundle By Name(w338) -> ("数组 2[24]"=w337:sgl, "数组 2[25]"=w336:sgl, "数组 2[26]"=w335:sgl)
                  }
                  frame "高量程" {
                    n304 = Unbundle By Name(w342) -> ("数组 2[27]"=w341:sgl, "数组 2[28]"=w340:sgl, "数组 2[29]"=w339:sgl)
                  }
                  frame "0-2量程" {
                    n305 = Unbundle By Name(w346) -> ("数组 2[6]"=w345:sgl, "数组 2[7]"=w344:sgl, "数组 2[8]"=w343:sgl)
                  }
                }
                n306 = Bundle By Name(cluster=cluster{"X":dbl, "b":dbl, "X^2":dbl} {"X"=0.0, "b"=0.0, "X^2"=0.0} ("方程系数"), "X"=w334, "b"=w333, "X^2"=w332) -> (w329:cluster{"X":dbl, "b":dbl, "X^2":dbl})
              }
              frame 6 {
                n307 = local read "量程选择"() -> (w350:enum16{"低量程", "高量程", "0-2量程"})
                n308 = case shown="\"高量程\"" w350 {
                  tunnel: w347 -> [w357 w361 w365]
                  tunnel: [w356 w360 w364] -> w353
                  tunnel: [w355 w359 w363] -> w352
                  tunnel: [w354 w358 w362] -> w351
                  frame "低量程", Default {
                    n309 = Unbundle By Name(w357) -> ("数组 2[30]"=w356:sgl, "数组 2[31]"=w355:sgl, "数组 2[32]"=w354:sgl)
                  }
                  frame "高量程" {
                    n310 = Unbundle By Name(w361) -> ("数组 2[33]"=w360:sgl, "数组 2[34]"=w359:sgl, "数组 2[35]"=w358:sgl)
                  }
                  frame "0-2量程" {
                    n311 = Unbundle By Name(w365) -> ("数组 2[6]"=w364:sgl, "数组 2[7]"=w363:sgl, "数组 2[8]"=w362:sgl)
                  }
                }
                n312 = Bundle By Name(cluster=cluster{"X":dbl, "b":dbl, "X^2":dbl} {"X"=0.0, "b"=0.0, "X^2"=0.0} ("方程系数"), "X"=w353, "b"=w352, "X^2"=w351) -> (w348:cluster{"X":dbl, "b":dbl, "X^2":dbl})
              }
              frame 7 {
                n313 = local read "量程选择"() -> (w369:enum16{"低量程", "高量程", "0-2量程"})
                n314 = case shown="\"高量程\"" w369 {
                  tunnel: w366 -> [w376 w380 w384]
                  tunnel: [w375 w379 w383] -> w372
                  tunnel: [w374 w378 w382] -> w371
                  tunnel: [w373 w377 w381] -> w370
                  frame "低量程", Default {
                    n315 = Unbundle By Name(w376) -> ("数组 2[36]"=w375:sgl, "数组 2[37]"=w374:sgl, "数组 2[38]"=w373:sgl)
                  }
                  frame "高量程" {
                    n316 = Unbundle By Name(w380) -> ("数组 2[39]"=w379:sgl, "数组 2[40]"=w378:sgl, "数组 2[41]"=w377:sgl)
                  }
                  frame "0-2量程" {
                    n317 = Unbundle By Name(w384) -> ("数组 2[6]"=w383:sgl, "数组 2[7]"=w382:sgl, "数组 2[8]"=w381:sgl)
                  }
                }
                n318 = Bundle By Name(cluster=cluster{"X":dbl, "b":dbl, "X^2":dbl} {"X"=0.0, "b"=0.0, "X^2"=0.0} ("方程系数"), "X"=w372, "b"=w371, "X^2"=w370) -> (w367:cluster{"X":dbl, "b":dbl, "X^2":dbl})
              }
            }
            n319 = local write "方程系数"(w247) -> ()
          }
        }
      }
    }
    n320 = Wait (ms)(milliseconds to wait=u32 1000 ("等待时间（毫秒）")) -> ()  [unwired: 1 out]
  }
  n321 = while {
    tunnel: w15 -> [w535]
    tunnel: w14 -> [w534]
    tunnel: w5 -> [_]
    stop <- FALSE stop-if-true
    # "主循环界面显示"
    n322 = flat-sequence {
      frame #0 {
        # "A，B，K"
        # "CODMn读取状态"
        n323 = global read "COD内部交互全局.vi" "ORP、时间"() -> (w664:u16[])
        n324 = To Word Integer(number=w664) -> (16bit integer=w685:i16[])
        n325 = Split 1D Array(array=w685, index=3 ("索引")) -> (first subarray=w666:i16[], second subarray=w684:i16[])
        n326 = Index Array(array=w666) -> (element #1=w670:i16, element #2=w669:i16, element #3=w668:i16)  [unwired: 3 in]
        n327 = Index Array(array=w684) -> (element #1=w679:i16, element #2=w683:i16, element #3=w682:i16, element #4=w681:i16)  [unwired: 4 in]
        n328 = To Single Precision Float(number=w681) -> (single precision float=w672:sgl)
        n329 = Build Array(w670, w669, w668) -> (w667:i16[])
        n330 = To Single Precision Float(number=w679) -> (single precision float=w678:sgl)
        n331 = To Single Precision Float(number=w683) -> (single precision float=w677:sgl)
        n332 = To Single Precision Float(number=w682) -> (single precision float=w673:sgl)
        n333 = call "HexToDate.vi"("数组"=w667) -> ("DATE"=w671:timestamp[])  [unwired: 10 in]
        n334 = Number To Decimal String(number=w677) -> (decimal integer string=→"ORP-A":string)  [unwired: 1 in]
        n335 = Number To Decimal String(number=w673) -> (decimal integer string=→"ORP-B":string)  [unwired: 1 in]
        n336 = Number To Decimal String(number=w672) -> (decimal integer string=→"ORP-K":string)  [unwired: 1 in]
        n337 = Divide(x=w678, y=sgl 100.0) -> (x/y=→"COD浓度（mg/L)":sgl)
        n338 = Index Array(array=w671) -> (element=w665:timestamp)  [unwired: 1 in]
        n339 = Format Date/Time String(seconds (now)=w665) -> (date/time string=→"数据时间":string)  [unwired: 2 in]
      }
    }
    n340 = flat-sequence {
      frame #0 {
        # "测量状态显示"
        n341 = global read "COD内部交互全局.vi" "测量状态"() -> (w584:u16[])
        n342 = To Word Integer(number=w584) -> (16bit integer=w594:i16[])
        n343 = Index Array(array=w594, index #1=0 ("索引"), index #4=3 ("索引"), index #14=13 ("索引"), index #15=14 ("索引"), index #21=20 ("索引"), index #32=31 ("索引")) -> (element #1=w598:i16, element #2=w597:i16, element #3=w596:i16, element #4=w580:i16, element #5=→"模式（受控）":i16, element #6=→"进样管":i16, element #7=→"高锰酸钾":i16, element #8=→"草酸钠":i16, element #9=→"硫酸":i16, element #10=w593:i16, element #11=w613:i16, element #12=w589:i16, element #13=→"报警数字":i16, element #14=w619:i16, element #15=w604:i16, element #16=→"多列列表框":i16, element #20=→"氢氧化钠":i16, element #21=w577:i16, element #33=→"分":i16, element #34=→"秒":i16)  [unwired: 28 in, 14 out]
        "CODMn工作状态" <- w580
        n344 = global write "COD内部交互全局.vi" "基本量程实时读取"(w577) -> ()
        n345 = Build Array(w598, w597, w596) -> (w599:i16[])
        n346 = To Single Precision Float(number=w593) -> (single precision float=→"实时ORP":sgl)
        n347 = Number To Decimal String(number=w577) -> (decimal integer string=→"基本量程(显示)":string)  [unwired: 1 in]
        n348 = Equal?(x=w589, y=u16 1) -> (x = y?=→"排液标记":bool)
        n349 = Equal?(x=w589, y=u16 2) -> (x = y?=→"断电排液标记":bool)
        n350 = Divide(x=w613, y=u16 10) -> (x/y=→"温度℃":dbl)
        n351 = Divide(x=w619, y=u16 1000) -> (x/y=→"零点滴定值":dbl)
        n352 = Divide(x=w604, y=u16 1000) -> (x/y=→"标度滴定值":dbl)
        n353 = Equal?(x=w580, y=T3."水样测试" ("CODMn工作状态")) -> (x = y?=w578:bool)
        n354 = call "HexToDate.vi"("数组"=w599) -> ("DATE"=w595:timestamp[])  [unwired: 10 in]
        n355 = case shown="真" w578 {
          tunnel: w577 -> [_ w622]
          frame False {
          }
          frame True {
            n356 = global write "CODMn断电保存全局变量.vi" "水样测试量程"(w622) -> ()
          }
        }
        n357 = Index Array(array=w595) -> (element=→"仪器时间":timestamp)  [unwired: 1 in]
      }
    }
    n358 = flat-sequence {
      frame #0 {
        # "报警状态显示"
        n359 = global read "COD内部交互全局.vi" "报警点位"() -> (w637:bool[])
        n360 = Index Array(array=w637, index #1=0 ("索引")) -> (element #1=w634:bool, element #2=w633:bool, element #3=w632:bool, element #4=w631:bool, element #5=w630:bool, element #6=w629:bool, element #7=w628:bool, element #8=w627:bool, element #9=w626:bool, element #11=w625:bool, element #13=w624:bool, element #14=w623:bool)  [unwired: 13 in, 2 out]
        "ORP故障" <- w634
        "温控器故障" <- w633
        "加热故障" <- w626
        "高锰酸钾报警" <- w628
        "草酸钠报警" <- w627
        "测量错误" <- w632
        "校零错误" <- w631
        "校标错误" <- w630
        "进水样超量程" <- w629
        "排液故障" <- w625
        "60分钟超时报警" <- w624
        "进样无液体告警" <- w623
        n361 = Compound Arithmetic op=OR ("复合运算")(w634, w633, w626, w628, w627, w632, w630, w631, w629, w625, w624) -> (→"故障标记":bool)
        n362 = Bundle By Name(cluster=T13 {"ORP故障"=FALSE, "温控器故障"=FALSE, "加热故障"=FALSE, "高锰酸钾报警"=FALSE, "草酸钠报警"=FALSE, "测量错误"=FALSE, "校零错误"=FALSE, "校标错误"=FALSE, " 进水样超量程"=FALSE, "排液阀故障"=FALSE, "60分钟超时报警"=FALSE, "进样无液体报警"=FALSE} ("报警簇"), "ORP故障"=w634, "温控器故障"=w633, "加热故障"=w626, "高锰酸钾报警"=w628, "草酸钠报警"=w627, "测量错误"=w632, "校零错误"=w631, "校标错误"=w630, "进水样超量程"=w629, "排液阀故障"=w625, "60分钟超时报警"=w624, "进样无液体报警"=w623) -> (w635:T13)
        n363 = global write "COD内部交互全局.vi" "报警簇"(w635) -> ()
      }
    }
    n364 = flat-sequence {
      frame #0 {
        # "CODMn读取状态"
        n365 = global read "COD内部交互全局.vi" "温度"() -> (w661:bool[])
        n366 = global read "COD内部交互全局.vi" "M输出点"() -> (w660:bool[])
        n367 = Index Array(array=w661) -> (element=→"加热":bool)  [unwired: 1 in]
        n368 = Index Array(array=w660) -> (element #1=→"搅拌":bool, element #4=→"进水样":bool, element #5=→"进蒸馏水":bool, element #6=→"进标液":bool, element #7=→"进零点核查样":bool, element #8=→"进加标回收样":bool, element #9=→"进高锰酸钾":bool, element #10=→"进草酸钠":bool, element #11=→"进硫酸":bool)  [unwired: 11 in, 2 out]
      }
    }
    n369 = flat-sequence {
      frame #0 {
        # "工作状态显示"
        n370 = local read "CODMn工作状态"() -> (w545:T3)
        n371 = case shown="\"标样校准\"" w545 {
          tunnel: [_ u16 0 ("y") u16 1 ("y") u16 2 ("y") u16 3 ("y") u16 4 ("y") u16 6 ("y") _ u16 7 ("y") u16 8 ("y") u16 5 ("y")] -> w544
          frame "空闲", Default {
          }
          frame "水样测试" {
          }
          frame "标样核查" {
          }
          frame "零点核查" {
          }
          frame "跨度核查" {
          }
          frame "空白测试" {
          }
          frame "平行样测试" {
          }
          frame "质控样" {
          }
          frame "空白校准" {
          }
          frame "标样校准" {
          }
          frame "加标回收" {
          }
        }
        n372 = Equal?(x=w545, y=u16 8) -> (x = y?=→"校零标记":bool)
        n373 = Equal?(x=w545, y=u16 4) -> (x = y?=→"跨度核查标记":bool)
        n374 = Equal?(x=w545, y=u16 0) -> (x = y?=→"待机":bool)
        n375 = Equal?(x=w545, y=u16 3) -> (x = y?=→"零点核查标记":bool)
        n376 = Equal?(x=w545, y=u16 7) -> (x = y?=→"质控样测量":bool)
        n377 = Equal?(x=w545, y=u16 1) -> (x = y?=→"水样测量":bool)
        n378 = Equal?(x=w545, y=u16 2) -> (x = y?=→"标样核查标记":bool)
        n379 = Equal?(x=w545, y=u16 6) -> (x = y?=→"平行样测量":bool)
        n380 = Equal?(x=w545, y=u16 9) -> (x = y?=→"校标标记":bool)
        n381 = Equal?(x=w545, y=u16 5) -> (x = y?=→"空白测试标记":bool)
        n382 = Equal?(x=w545, y=u16 10) -> (x = y?=→"加标回收测量":bool)
        n383 = global write "COD内部交互全局.vi" "测量模式数字"(w544) -> ()
      }
    }
    n384 = Get Date/Time In Seconds() -> (seconds since 1Jan1904=→"系统时间":timestamp)
    n385 = First Call?() -> (First Call?: T/F=w533:bool)
    n386 = Wait (ms)(milliseconds to wait=u32 1000 ("等待时间（毫秒）")) -> ()  [unwired: 1 out]
    n387 = case shown="真" w533 {
      tunnel: w535 -> [w641 w646]
      tunnel: w534 -> [w640 w645]
      tunnel: [w641 w644] -> w531
      tunnel: [w640 w643] -> w530
      frame False {
      }
      frame True {
        n388 = Bundle By Name(cluster=cluster{"命令":string} {"命令"=""} ("元素"), "命令"="CODMn读取参数" ("名称（未命名）")) -> (w649:cluster{"命令":string})
        n389 = Enqueue Element(queue=w646, element=w649, timeout in ms (-1)=1000 ("超时毫秒(-1)"), error in (no error)=w645) -> (queue out=w644:refnum<queue>, error out=w643:errorcluster)  [unwired: 1 out]
      }
    }
    n390 = Get Queue Status(queue=w531, error in (no error)=w530) -> (queue out=w527:refnum<queue>, error out=w526:errorcluster, # elements in queue=w529:i32)  [unwired: 1 in, 5 out]
    n391 = Equal To 0?(x=w529) -> (x = 0?=w528:bool)
    n392 = case shown="真" w528 {
      tunnel: w527 -> [_ w539]
      tunnel: w526 -> [_ w538]
      frame False {
      }
      frame True {
        n393 = Bundle By Name(cluster=cluster{"命令":string} {"命令"=""} ("元素"), "命令"="CODMn读取" ("名称（未命名）")) -> (w541:cluster{"命令":string})
        n394 = Enqueue Element(queue=w539, element=w541, timeout in ms (-1)=1000 ("超时毫秒(-1)"), error in (no error)=w538) -> ()  [unwired: 3 out]
      }
    }
  }
  n395 = while {
    stop <- FALSE stop-if-true
    # "数字键盘输入"
    n396 = event shown="[23] \"泵滴定数1\": 鼠标按下" {
      selector: _ -> [_ _ _ _ _ _ _ _ _ _ _ _ _ _ _ _ _ _ _ _ _ _ _ _ _ _ _ _ _ _]
      dyn-events: _ -> [_ _ _ _ _ _ _ _ _ _ _ _ _ _ _ _ _ _ _ _ _ _ _ _ _ _ _ _ _ _]
      timeout: _ -> [_ _ _ _ _ _ _ _ _ _ _ _ _ _ _ _ _ _ _ _ _ _ _ _ _ _ _ _ _ _]
      event Timeout {
        n397 = event-data() -> ()  [unwired: 1 in, 3 out]
      }
      event "温度": Mouse Down {
        n398 = event-data() -> ()  [unwired: 1 in, 8 out]
        n399 = local read "温度"() -> (w689:dbl)
        n400 = call "数字键盘.vi"("OldNumber"=w689) -> ("NewNumber"=w688:sgl)
        n401 = local write "温度"(w688) -> ()
      }
      event "恒温时间": Mouse Down {
        n402 = event-data() -> ()  [unwired: 1 in, 8 out]
        n403 = local read "恒温时间"() -> (w690:dbl)
        n404 = call "数字键盘.vi"("OldNumber"=w690) -> ("NewNumber"=w691:sgl)
        n405 = local write "恒温时间"(w691) -> ()
      }
      event "标准液浓度": Mouse Down {
        n406 = event-data() -> ()  [unwired: 1 in, 8 out]
        n407 = local read "标准液浓度"() -> (w693:dbl)
        n408 = call "数字键盘.vi"("OldNumber"=w693) -> ("NewNumber"=w692:sgl)
        n409 = local write "标准液浓度"(w692) -> ()
      }
      event "氢氧化钠：": Mouse Down {
        n410 = event-data() -> ()  [unwired: 1 in, 8 out]
        n411 = local read "氢氧化钠："() -> (w694:dbl)
        n412 = call "数字键盘.vi"("OldNumber"=w694) -> ("NewNumber"=w695:sgl)
        n413 = local write "氢氧化钠："(w695) -> ()
      }
      event "水样：": Mouse Down {
        n414 = event-data() -> ()  [unwired: 1 in, 8 out]
        n415 = local read "水样："() -> (w696:dbl)
        n416 = call "数字键盘.vi"("OldNumber"=w696) -> ("NewNumber"=w697:sgl)
        n417 = local write "水样："(w697) -> ()
      }
      event "蒸馏水：": Mouse Down {
        n418 = event-data() -> ()  [unwired: 1 in, 8 out]
        n419 = local read "蒸馏水："() -> (w698:dbl)
        n420 = call "数字键盘.vi"("OldNumber"=w698) -> ("NewNumber"=w699:sgl)
        n421 = local write "蒸馏水："(w699) -> ()
      }
      event "标液：": Mouse Down {
        n422 = event-data() -> ()  [unwired: 1 in, 8 out]
        n423 = local read "标液："() -> (w700:dbl)
        n424 = call "数字键盘.vi"("OldNumber"=w700) -> ("NewNumber"=w701:sgl)
        n425 = local write "标液："(w701) -> ()
      }
      event "零点核查样：": Mouse Down {
        n426 = event-data() -> ()  [unwired: 1 in, 8 out]
        n427 = local read "零点核查样："() -> (w702:dbl)
        n428 = call "数字键盘.vi"("OldNumber"=w702) -> ("NewNumber"=w703:sgl)
        n429 = local write "零点核查样："(w703) -> ()
      }
      event "加标回收样：": Mouse Down {
        n430 = event-data() -> ()  [unwired: 1 in, 8 out]
        n431 = local read "加标回收样："() -> (w704:dbl)
        n432 = call "数字键盘.vi"("OldNumber"=w704) -> ("NewNumber"=w705:sgl)
        n433 = local write "加标回收样："(w705) -> ()
      }
      event "草酸钠": Mouse Down {
        n434 = event-data() -> ()  [unwired: 1 in, 8 out]
        n435 = local read "草酸钠"() -> (w706:dbl)
        n436 = call "数字键盘.vi"("OldNumber"=w706) -> ("NewNumber"=w707:sgl)
        n437 = local write "草酸钠"(w707) -> ()
      }
      event "高锰酸钾": Mouse Down {
        n438 = event-data() -> ()  [unwired: 1 in, 8 out]
        n439 = local read "高锰酸钾"() -> (w708:dbl)
        n440 = call "数字键盘.vi"("OldNumber"=w708) -> ("NewNumber"=w709:sgl)
        n441 = local write "高锰酸钾"(w709) -> ()
      }
      event "硫酸": Mouse Down {
        n442 = event-data() -> ()  [unwired: 1 in, 8 out]
        n443 = local read "硫酸"() -> (w710:dbl)
        n444 = call "数字键盘.vi"("OldNumber"=w710) -> ("NewNumber"=w711:sgl)
        n445 = local write "硫酸"(w711) -> ()
      }
      event "零点泵计量数 2": Mouse Down {
        n446 = event-data() -> ()  [unwired: 1 in, 8 out]
        n447 = local read "零点泵计量数 2"() -> (w712:dbl)
        n448 = call "数字键盘.vi"("OldNumber"=w712) -> ("NewNumber"=w713:sgl)
        n449 = local write "零点泵计量数 2"(w713) -> ()
      }
      event "标度泵计量数 2": Mouse Down {
        n450 = event-data() -> ()  [unwired: 1 in, 8 out]
        n451 = local read "标度泵计量数 2"() -> (w714:dbl)
        n452 = call "数字键盘.vi"("OldNumber"=w714) -> ("NewNumber"=w715:sgl)
        n453 = local write "标度泵计量数 2"(w715) -> ()
      }
      event "高量程稀释倍数:": Mouse Down {
        n454 = event-data() -> ()  [unwired: 1 in, 8 out]
        n455 = local read "高量程稀释倍数:"() -> (w717:i8)
        n456 = call "数字键盘.vi"("OldNumber"=w717) -> ("NewNumber"=w716:sgl)
        n457 = local write "高量程稀释倍数:"(w716) -> ()
      }
      event "低量程稀释倍数:": Mouse Down {
        n458 = event-data() -> ()  [unwired: 1 in, 8 out]
        n459 = local read "低量程稀释倍数:"() -> (w719:i8)
        n460 = call "数字键盘.vi"("OldNumber"=w719) -> ("NewNumber"=w718:sgl)
        n461 = local write "低量程稀释倍数:"(w718) -> ()
      }
      event "浓度1": Mouse Down {
        n462 = event-data() -> ()  [unwired: 1 in, 8 out]
        n463 = local read "浓度1"() -> (w721:dbl)
        n464 = call "数字键盘.vi"("OldNumber"=w721) -> ("NewNumber"=w720:sgl)
        n465 = property on="浓度1" class="DigNum (严格)"("Val(Sgnl)"=w720) -> ()  [unwired: 2 in, 2 out]
      }
      event "浓度2": Mouse Down {
        n466 = event-data() -> ()  [unwired: 1 in, 8 out]
        n467 = local read "浓度2"() -> (w723:dbl)
        n468 = call "数字键盘.vi"("OldNumber"=w723) -> ("NewNumber"=w722:sgl)
        n469 = property on="浓度2" class="DigNum (严格)"("Val(Sgnl)"=w722) -> ()  [unwired: 2 in, 2 out]
      }
      event "浓度3": Mouse Down {
        n470 = event-data() -> ()  [unwired: 1 in, 8 out]
        n471 = local read "浓度3"() -> (w725:dbl)
        n472 = call "数字键盘.vi"("OldNumber"=w725) -> ("NewNumber"=w724:sgl)
        n473 = property on="浓度3" class="DigNum (严格)"("Val(Sgnl)"=w724) -> ()  [unwired: 2 in, 2 out]
      }
      event "浓度4": Mouse Down {
        n474 = event-data() -> ()  [unwired: 1 in, 8 out]
        n475 = local read "浓度4"() -> (w727:dbl)
        n476 = call "数字键盘.vi"("OldNumber"=w727) -> ("NewNumber"=w726:sgl)
        n477 = property on="浓度4" class="DigNum (严格)"("Val(Sgnl)"=w726) -> ()  [unwired: 2 in, 2 out]
      }
      event "浓度5": Mouse Down {
        n478 = event-data() -> ()  [unwired: 1 in, 8 out]
        n479 = local read "浓度5"() -> (w729:dbl)
        n480 = call "数字键盘.vi"("OldNumber"=w729) -> ("NewNumber"=w728:sgl)
        n481 = property on="浓度5" class="DigNum (严格)"("Val(Sgnl)"=w728) -> ()  [unwired: 2 in, 2 out]
      }
      event "跨度液浓度", "零点核查浓度", "标样浓度": Mouse Down {
        n482 = event-data() -> ("CtlRef"=w733:refnum<vi>)  [unwired: 1 in, 7 out]
        n483 = property class="DigNum (严格)"(reference=w733) -> (reference out=w730:refnum<vi>, "Value"=w732:dbl)  [unwired: 1 in, 1 out]
        n484 = call "数字键盘.vi"("OldNumber"=w732) -> ("NewNumber"=w731:sgl)
        n485 = property class="DigNum (严格)"(reference=w730, "Val(Sgnl)"=w731) -> ()  [unwired: 1 in, 2 out]
      }
      event "泵滴定数1": Mouse Down {
        n486 = event-data() -> ()  [unwired: 1 in, 8 out]
        n487 = local read "泵滴定数1"() -> (w735:dbl)
        n488 = call "数字键盘.vi"("OldNumber"=w735) -> ("NewNumber"=w734:sgl)
        n489 = property on="泵滴定数1" class="DigNum (严格)"("Val(Sgnl)"=w734) -> ()  [unwired: 2 in, 2 out]
      }
      event "泵滴定数2": Mouse Down {
        n490 = event-data() -> ()  [unwired: 1 in, 8 out]
        n491 = local read "泵滴定数2"() -> (w737:dbl)
        n492 = call "数字键盘.vi"("OldNumber"=w737) -> ("NewNumber"=w736:sgl)
        n493 = property on="泵滴定数2" class="DigNum (严格)"("Val(Sgnl)"=w736) -> ()  [unwired: 2 in, 2 out]
      }
      event "泵滴定数3": Mouse Down {
        n494 = event-data() -> ()  [unwired: 1 in, 8 out]
        n495 = local read "泵滴定数3"() -> (w739:dbl)
        n496 = call "数字键盘.vi"("OldNumber"=w739) -> ("NewNumber"=w738:sgl)
        n497 = property on="泵滴定数3" class="DigNum (严格)"("Val(Sgnl)"=w738) -> ()  [unwired: 2 in, 2 out]
      }
      event "泵滴定数4": Mouse Down {
        n498 = event-data() -> ()  [unwired: 1 in, 8 out]
        n499 = local read "泵滴定数4"() -> (w741:dbl)
        n500 = call "数字键盘.vi"("OldNumber"=w741) -> ("NewNumber"=w740:sgl)
        n501 = property on="泵滴定数4" class="DigNum (严格)"("Val(Sgnl)"=w740) -> ()  [unwired: 2 in, 2 out]
      }
      event "泵滴定数5": Mouse Down {
        n502 = event-data() -> ()  [unwired: 1 in, 8 out]
        n503 = local read "泵滴定数5"() -> (w743:dbl)
        n504 = call "数字键盘.vi"("OldNumber"=w743) -> ("NewNumber"=w742:sgl)
        n505 = property on="泵滴定数5" class="DigNum (严格)"("Val(Sgnl)"=w742) -> ()  [unwired: 2 in, 2 out]
      }
      event "低切高阈值:", "高切低阈值:": Mouse Down {
        n506 = event-data() -> ("CtlRef"=w747:refnum<vi>)  [unwired: 1 in, 7 out]
        n507 = property class="DigNum (严格)"(reference=w747) -> (reference out=w746:refnum<vi>, "Value"=w745:dbl)  [unwired: 1 in, 1 out]
        n508 = call "数字键盘.vi"("OldNumber"=w745) -> ("NewNumber"=w744:sgl)
        n509 = property class="DigNum (严格)"(reference=w746, "Val(Sgnl)"=w744) -> ()  [unwired: 1 in, 2 out]
      }
      event "远程自动校准浓度": Mouse Down {
        n510 = event-data() -> ("CtlRef"=w748:refnum<vi>)  [unwired: 1 in, 7 out]
        n511 = One Button Dialog(message="请输入其中一个在拟合公式中的非零浓度，用于远程校标！" ("消息")) -> (true=w750:bool)  [unwired: 1 in]
        n512 = case shown="真" w750 {
          tunnel: w748 -> [_ w757]
          frame False {
          }
          frame True {
            n513 = property class="DigNum (严格)"(reference=w757) -> (reference out=w752:refnum<vi>, "Value"=w758:dbl)  [unwired: 1 in, 1 out]
            n514 = global read "COD内部交互全局.vi" "启用的浓度数组"() -> (w754:dbl[])
            n515 = call "数字键盘.vi"("OldNumber"=w758) -> ("NewNumber"=w751:sgl)
            n516 = Search 1D Array(1D array=w754, element=w751) -> (index of element=w755:i32)  [unwired: 1 in]
            n517 = Equal?(x=w755, y=-1) -> (x = y?=w753:bool)
            n518 = case shown="真" w753 {
              tunnel: w752 -> [w760 _]
              tunnel: w751 -> [w759 _]
              frame False {
                n519 = property class="DigNum (严格)"(reference=w760, "Val(Sgnl)"=w759) -> ()  [unwired: 1 in, 2 out]
              }
              frame True {
                n520 = One Button Dialog(message="该浓度不属于校准浓度范围，请重新输入！" ("消息")) -> ()  [unwired: 1 in, 1 out]
              }
            }
          }
        }
      }
    }
  }
  n521 = while {
    tunnel: w15 -> [w763]
    tunnel: w14 -> [w762]
    stop <- FALSE stop-if-true
    # "主线事件"
    n522 = event shown="[1] \"启动\": 鼠标按下" {
      selector: _ -> [_ _ _ _ _ _ _ _ _ _ _ _ _ _ _ _ _ _ _ _ _ _ _ _ _ _ _ _ _ _ _ _ _ _]
      dyn-events: _ -> [_ _ _ _ _ _ _ _ _ _ _ _ _ _ _ _ _ _ _ _ _ _ _ _ _ _ _ _ _ _ _ _ _ _]
      timeout: _ -> [_ _ _ _ _ _ _ _ _ _ _ _ _ _ _ _ _ _ _ _ _ _ _ _ _ _ _ _ _ _ _ _ _ _]
      tunnel: w763 -> [_ _ _ _ _ w854 _ _ _ _ _ _ _ _ _ _ _ _ _ _ w1293 _ _ _ w1505 _ _ _ _ w1795 w1802 w1824 w1867 _]
      tunnel: w762 -> [_ _ _ _ _ w853 _ _ _ _ _ _ _ _ _ _ _ _ _ _ w1290 _ _ _ w1504 _ _ _ _ w1794 w1801 w1823 w1866 _]
      event "单步启动": Value Change {
        n523 = event-data() -> ()  [unwired: 1 in, 6 out]
        n524 = call "CODMn手动控制框.vi"() -> ()  [unwired: 12 in]
      }
      event "启动": Mouse Down {
        n525 = event-data() -> ()  [unwired: 1 in, 8 out]
        n526 = global read "COD内部交互全局.vi" "基本量程实时读取"() -> (w767:enum16{"L", "H", "AUTO"})
        n527 = call "启动测量模式选择对话框.vi"("量程选择"=w767) -> ("标样浓度输出"=w765:dbl, "量程选择输出"=w766:enum16{"L", "H", "AUTO"}, "启动选择输出"=w771:u16)  [unwired: 8 in]
        n528 = Not Equal?(x=w771, y=u16 8) -> (x != y?=w768:bool)
        n529 = Not Equal?(x=w771, y=u16 7) -> (x != y?=w769:bool)
        n530 = And(x=w769, y=w768) -> (x .and. y?=w773:bool)
        n531 = case shown="真" w773 {
          tunnel: w771 -> [_ w788]
          tunnel: w766 -> [_ w779]
          tunnel: w765 -> [_ w778]
          frame False {
            n532 = One Button Dialog(message="请到校准配置里面进行校准操作！" ("消息")) -> ()  [unwired: 1 in, 1 out]
          }
          frame True {
            n533 = Not Equal?(x=w788, y=u16 9) -> (x != y?=w783:bool)
            n534 = case shown="\"H\"" w779 {
              tunnel: [w789 w793 errorcluster {"status"=FALSE, "code"=0, "source"=""} ("error out")] -> w777
              frame "L", Default {
                n535 = call "CODMnMB_api.vi"("STEP"=enum16{"open", "read", "write", "close"}."write", "values"=u16[] [0], "starting address"=u16 4276) -> ("error out"=w789:errorcluster)  [unwired: 6 in, 2 out]
              }
              frame "H" {
                n536 = call "CODMnMB_api.vi"("STEP"=enum16{"open", "read", "write", "close"}."write", "values"=u16[] [1], "starting address"=u16 4276) -> ("error out"=w793:errorcluster)  [unwired: 6 in, 2 out]
              }
              frame "AUTO" {
              }
            }
            n537 = global write "CODMN外部API.vi" "手动启动CODMn"(w783) -> ()
            n538 = call "单步测试一键复位.vi"("Error in"=w777) -> ("error out"=w776:errorcluster)  [unwired: 10 in]
            n539 = call <vilib>:"Clear Errors.vi"("error in (no error)"=w776) -> ("error out"=w775:errorcluster)  [unwired: 5 in, 1 out]
            n540 = case shown="0" w788 {
              tunnel: [u16 4608 ("address") u16 4608 ("address") u16 4608 ("address") u16 4608 ("address") u16 4608 ("address") u16 4608 ("address") u16 4608 ("address") u16 4608 ("address") u16 4608 ("address") u16 4608 ("address")] -> w781
              tunnel: [u16 1 ("address") u16 2 ("address") u16 3 ("address") u16 4 ("address") u16 5 ("address") u16 7 ("address") u16 6 ("address") u16 8 ("address") u16 9 ("address") u16 0 ("address")] -> w785
              tunnel: w778 -> [_ w801 _ _ _ _ _ _ _ _]
              frame 0 {
              }
              frame 1 {
                n541 = property on="标样浓度" class="DigNum (严格)"("Val(Sgnl)"=w801) -> ()  [unwired: 2 in, 2 out]
              }
              frame 2 {
              }
              frame 3 {
              }
              frame 4 {
              }
              frame 5 {
              }
              frame 6 {
              }
              frame 7 {
              }
              frame 8 {
              }
              frame 9, Default {
              }
            }
            n542 = Insert Into Array(array=u16[] [] ("values"), index=0 ("索引"), new element=w785) -> (w780:u16[])
            n543 = call "CODMnMB_api.vi"("STEP"=enum16{"open", "read", "write", "close"}."write", "Error in"=w775, "values"=w780, "starting address"=w781) -> ()  [unwired: 5 in, 3 out]
          }
        }
      }
      event "停止": Value Change {
        n544 = event-data() -> ()  [unwired: 1 in, 6 out]
        n545 = Two Button Dialog(message="确认是否停止？" ("消息"), 1:"否" ("F按钮名称（“取消”）"), 2:"是" ("T按钮名称（“确定”）")) -> (T button?=w821:bool)
        n546 = case shown="真" w821 {
          frame False {
          }
          frame True {
            n547 = Obtain Notifier(name (unnamed)="CODMn" ("名称（未命名）"), notification data type=FALSE) -> (notifier out=w827:refnum<notifier>, error out=w825:errorcluster)  [unwired: 2 in, 1 out]
            n548 = Send Notification(notification=TRUE ("通知"), notifier=w827, error in (no error)=w825) -> (notifier out=w824:refnum<notifier>, error out=w823:errorcluster)
            n549 = Release Notifier(notifier=w824, error in (no error)=w823) -> ()  [unwired: 1 in, 3 out]
            n550 = call "CODMnMB_api.vi"("STEP"=enum16{"open", "read", "write", "close"}."write", "values"=u16[] [11], "starting address"=u16 4608) -> ()  [unwired: 6 in, 3 out]
          }
        }
      }
      event "手动控制": Value Change {
        n551 = event-data() -> ()  [unwired: 1 in, 6 out]
        n552 = call "数字密码键盘.vi"() -> ("NewNumber"=w833:sgl)  [unwired: 1 in]
        n553 = Equal?(x=w833, y=8.0) -> (x = y?=w834:bool)
        n554 = case shown="假" w834 {
          frame False {
            n555 = call "窗口弹出对话框(子VI).vi"("消息"="密码错误") -> ()  [unwired: 10 in, 1 out]
          }
          frame True {
          }
        }
      }
      event "锁定按钮": Mouse Down {
        n556 = event-data() -> ("CtlRef"=w839:refnum<vi>)  [unwired: 1 in, 7 out]
        n557 = property class="Bool (严格)"(reference=w839) -> ("Value"=w838:bool)  [unwired: 1 in, 2 out]
        n558 = case shown="真" w838 {
          selector: w838 -> [w840 _]
          tunnel: [w840 w844] -> w837
          frame False {
          }
          frame True {
            n559 = call "数字密码键盘.vi"() -> ("NewNumber"=w841:sgl)  [unwired: 1 in]
            n560 = Equal?(x=w841, y=23506.0) -> (x = y?=w845:bool)
            n561 = Equal?(x=w841, y=8.0) -> (x = y?=w842:bool)
            n562 = Or(x=w845, y=w842) -> (x .or. y?=w844:bool)
            n563 = case shown="假" w844 {
              selector: w844 -> [w848 _]
              frame False {
                n564 = local write "锁定按钮"(w848) -> ()
                n565 = One Button Dialog(message="密码错误!" ("消息")) -> ()  [unwired: 1 in, 1 out]
              }
              frame True {
                n566 = One Button Dialog(message="解锁成功!" ("消息")) -> ()  [unwired: 1 in, 1 out]
              }
            }
          }
        }
        "x = y?" <- w837
      }
      event "参数配置": Value Change {
        (unwired) u16 20 ("number of holding registers")
        (unwired) u16 4272 ("starting address")
        n567 = event-data() -> ()  [unwired: 1 in, 6 out]
        n568 = global read "CODMN外部API.vi" "ping"() -> (w852:bool)
        n569 = property on="窗格" class="Pane"("Origin"=T4 {"Horizontal"=0, "Vertical"=650} ("原点")) -> ()  [unwired: 2 in, 2 out]
        n570 = case shown="假" w852 {
          tunnel: [w864 w867] -> w851
          frame False {
            n571 = global read "COD内部交互全局.vi" "配置文件ini"() -> (w866:string)
            n572 = call <vilib>:"Application Directory.vi"() -> ("Application Directory"=w865:path)
            n573 = Build Path(base path=w865, name or relative path=w866) -> (appended path=w864:path)
          }
          frame True {
            n574 = global read "CODMN外部API.vi" "配置文件 path"() -> (w867:path)
          }
        }
        n575 = Bundle By Name(cluster=cluster{"命令":string} {"命令"=""} ("元素"), "命令"="CODMn读取参数" ("名称（未命名）")) -> (w855:cluster{"命令":string})
        n576 = call <vilib>:"Open Config Data.vi"("configuration file path"=w851) -> ("error out"=w861:errorcluster, "refnum"=w858:T6)  [unwired: 8 in, 1 out]
        n577 = Enqueue Element(queue=w854, element=w855, error in (no error)=w853) -> ()  [unwired: 1 in, 3 out]
        n578 = vi-ref "斯坦道CODMn.lvlib:CODMn断电保存全局变量.vi"() -> (w859:refnum<vi>)
        n579 = call <userlib>:"Read Panel from INI__ogtk.vi"("error in (no error)"=w861, "VI ref"=w859, "refnum"=w858) -> ("error out"=w862:errorcluster, "refnum out"=w860:T6)  [unwired: 7 in]
        n580 = call <vilib>:"Close Config Data.vi"("error in (no error)"=w862, "refnum"=w860) -> ("error out"=w850:errorcluster)  [unwired: 8 in, 1 out]
        n581 = call <vilib>:"Clear Errors.vi"("error in (no error)"=w850) -> ()  [unwired: 5 in, 2 out]
      }
      event "保存": Mouse Down {
        n582 = event-data() -> ()  [unwired: 1 in, 8 out]
        n583 = local read "通讯状态"() -> (w868:bool)
        n584 = Two Button Dialog(message="确定保存参数，保存参数将会替换原有参数！" ("消息")) -> (T button?=w870:bool)  [unwired: 2 in]
        n585 = case shown="真" w870 {
          tunnel: w868 -> [_ w871]
          frame False {
          }
          frame True {
            n586 = case shown="真" w871 {
              frame False {
                n587 = One Button Dialog(message="保存失败，当前无通讯！" ("消息")) -> ()  [unwired: 1 in, 1 out]
              }
              frame True {
                n588 = One Button Dialog(message="参数保存成功！" ("消息")) -> ()  [unwired: 1 in, 1 out]
                n589 = Build Array("采水泵进样时间/s:", "采水泵润洗时间/s:", "采水泵沉淀时间/s:", "采水泵排液时间/s:") -> (w874:i32[])
                n590 = call "CODMnMB_api.vi"("STEP"=enum16{"open", "read", "write", "close"}."write", "values"="保存参数", "starting address"=u16 4272) -> ("error out"=w880:errorcluster)  [unwired: 6 in, 2 out]
                n591 = call "CODMnMB_api.vi"("STEP"=enum16{"open", "read", "write", "close"}."write", "Error in"=w880, "values"=w874, "starting address"=u16 5596) -> ()  [unwired: 5 in, 3 out]
              }
            }
          }
        }
      }
      event "常规版/认证版": Value Change {
        n592 = event-data() -> ()  [unwired: 1 in, 6 out]
        n593 = flat-sequence {
          frame #0 {
            n594 = global write "CODMn断电保存全局变量.vi" "常规版/认证版"("常规版/认证版") -> ()
          }
          frame #1 {
            n595 = call "配置文件保存.vi"() -> ()  [unwired: 12 in]
          }
        }
      }
      event "校准配置": Value Change {
        w895 = "量程选择" ("section")
        n596 = event-data() -> ()  [unwired: 1 in, 6 out]
        n597 = global read "CODMN外部API.vi" "ping"() -> (w899:bool)
        n598 = property on="窗格" class="Pane"("Origin"=T4 {"Horizontal"=0, "Vertical"=1300} ("原点")) -> ()  [unwired: 2 in, 2 out]
        n599 = case shown="假" w899 {
          tunnel: [w977 w980] -> w898
          frame False {
            n600 = global read "COD内部交互全局.vi" "配置文件ini"() -> (w979:string)
            n601 = call <vilib>:"Application Directory.vi"() -> ("Application Directory"=w978:path)
            n602 = Build Path(base path=w978, name or relative path=w979) -> (appended path=w977:path)
          }
          frame True {
            n603 = global read "CODMN外部API.vi" "配置文件 path"() -> (w980:path)
          }
        }
        n604 = call <vilib>:"Open Config Data.vi"("configuration file path"=w898) -> ("error out"=w916:errorcluster, "refnum"=w917:T6)  [unwired: 8 in, 1 out]
        n605 = call-poly <vilib>:"Read Key.vi"("section"="CODMn模型选择" ("key"), "error in (no error)"=w916, "key"="线性和多项式", "refnum"=w917) -> ("error out"=w913:errorcluster, "value"=w915:i32, "refnum out"=w914:T6)  [unwired: 4 in, 1 out]
        n606 = local write "模型"(w915) -> ()
        n607 = call-poly <vilib>:"Read Key.vi"("section"="标线选择", "error in (no error)"=w913, "key"="选用水样", "refnum"=w914) -> ("error out"=w896:errorcluster, "value"=w900:i32, "refnum out"=w897:T6)  [unwired: 4 in, 1 out]
        n608 = local write "选用水样"(w900) -> ()
        n609 = case shown="0, 默认" w900 {
          tunnel: ["葡萄糖标线" ("section") "草酸钠标线" ("section")] -> w922
          frame 0, Default {
          }
          frame 1 {
          }
        }
        n610 = call-poly <vilib>:"Read Key.vi"("section"=w895, "error in (no error)"=w896, "key"=w895, "refnum"=w897) -> ("error out"=w893:errorcluster, "value"=w892:i32, "refnum out"=w894:T6)  [unwired: 4 in, 1 out]
        n611 = local write "量程选择"(w892) -> ()
        n612 = case shown="2" w892 {
          tunnel: ["低量程" "高量程" "0-2量程"] -> w921
          frame 0, Default {
          }
          frame 1 {
          }
          frame 2 {
          }
        }
        n613 = Concatenate Strings(w922, w921) -> (w920:string)
        n614 = call-poly <vilib>:"Read Key.vi"("section"=w920, "error in (no error)"=w893, "key"="浓度1", "refnum"=w894) -> ("error out"=w947:errorcluster, "value"=w945:dbl, "refnum out"=w946:T6)  [unwired: 4 in, 1 out]
        n615 = local write "浓度1"(w945) -> ()
        n616 = call-poly <vilib>:"Read Key.vi"("section"=w920, "error in (no error)"=w947, "key"="浓度2", "refnum"=w946) -> ("error out"=w961:errorcluster, "value"=w948:dbl, "refnum out"=w960:T6)  [unwired: 4 in, 1 out]
        n617 = local write "浓度2"(w948) -> ()
        n618 = call-poly <vilib>:"Read Key.vi"("section"=w920, "error in (no error)"=w961, "key"="浓度3", "refnum"=w960) -> ("error out"=w962:errorcluster, "value"=w950:dbl, "refnum out"=w959:T6)  [unwired: 4 in, 1 out]
        n619 = local write "浓度3"(w950) -> ()
        n620 = call-poly <vilib>:"Read Key.vi"("section"=w920, "error in (no error)"=w962, "key"="泵滴定数1", "refnum"=w959) -> ("error out"=w963:errorcluster, "value"=w952:dbl, "refnum out"=w958:T6)  [unwired: 4 in, 1 out]
        n621 = local write "泵滴定数1"(w952) -> ()
        n622 = call-poly <vilib>:"Read Key.vi"("section"=w920, "error in (no error)"=w963, "key"="泵滴定数2", "refnum"=w958) -> ("error out"=w957:errorcluster, "value"=w955:dbl, "refnum out"=w964:T6)  [unwired: 4 in, 1 out]
        n623 = local write "泵滴定数2"(w955) -> ()
        n624 = call-poly <vilib>:"Read Key.vi"("section"=w920, "error in (no error)"=w957, "key"="泵滴定数3", "refnum"=w964) -> ("error out"=w969:errorcluster, "value"=w968:dbl, "refnum out"=w965:T6)  [unwired: 4 in, 1 out]
        n625 = local write "泵滴定数3"(w968) -> ()
        n626 = call-poly <vilib>:"Read Key.vi"("section"=w920, "error in (no error)"=w969, "key"="浓度4", "refnum"=w965) -> ("error out"=w970:errorcluster, "value"=w906:dbl, "refnum out"=w966:T6)  [unwired: 4 in, 1 out]
        n627 = local write "浓度4"(w906) -> ()
        n628 = call-poly <vilib>:"Read Key.vi"("section"=w920, "error in (no error)"=w970, "key"="浓度5", "refnum"=w966) -> ("error out"=w911:errorcluster, "value"=w905:dbl, "refnum out"=w912:T6)  [unwired: 4 in, 1 out]
        n629 = local write "浓度5"(w905) -> ()
        n630 = call-poly <vilib>:"Read Key.vi"("section"=w920, "error in (no error)"=w911, "key"="泵滴定数4", "refnum"=w912) -> ("error out"=w971:errorcluster, "value"=w904:dbl, "refnum out"=w967:T6)  [unwired: 4 in, 1 out]
        n631 = local write "泵滴定数4"(w904) -> ()
        n632 = call-poly <vilib>:"Read Key.vi"("section"=w920, "error in (no error)"=w971, "key"="泵滴定数5", "refnum"=w967) -> ("error out"=w909:errorcluster, "value"=w903:dbl, "refnum out"=w910:T6)  [unwired: 4 in, 1 out]
        n633 = local write "泵滴定数5"(w903) -> ()
        n634 = call-poly <vilib>:"Read Key.vi"("section"=w920, "error in (no error)"=w909, "key"="当前选用的校准", "refnum"=w910) -> ("error out"=w941:errorcluster, "refnum out"=w942:T6)  [unwired: 4 in, 2 out]
        n635 = call-poly <vilib>:"Read Key.vi"("section"=w920, "error in (no error)"=w941, "key"="启用1", "refnum"=w942) -> ("error out"=w938:errorcluster, "value"=w927:bool, "refnum out"=w939:T6)  [unwired: 4 in, 1 out]
        n636 = local write "启用1"(w927) -> ()
        n637 = call-poly <vilib>:"Read Key.vi"("section"=w920, "error in (no error)"=w938, "key"="启用2", "refnum"=w939) -> ("error out"=w936:errorcluster, "value"=w926:bool, "refnum out"=w937:T6)  [unwired: 4 in, 1 out]
        n638 = local write "启用2"(w926) -> ()
        n639 = call-poly <vilib>:"Read Key.vi"("section"=w920, "error in (no error)"=w936, "key"="启用3", "refnum"=w937) -> ("error out"=w934:errorcluster, "value"=w925:bool, "refnum out"=w935:T6)  [unwired: 4 in, 1 out]
        n640 = local write "启用3"(w925) -> ()
        n641 = call-poly <vilib>:"Read Key.vi"("section"=w920, "error in (no error)"=w934, "key"="启用4", "refnum"=w935) -> ("error out"=w932:errorcluster, "value"=w902:bool, "refnum out"=w933:T6)  [unwired: 4 in, 1 out]
        n642 = local write "启用4"(w902) -> ()
        n643 = call-poly <vilib>:"Read Key.vi"("section"=w920, "error in (no error)"=w932, "key"="启用5", "refnum"=w933) -> ("error out"=w907:errorcluster, "value"=w901:bool, "refnum out"=w908:T6)  [unwired: 4 in, 1 out]
        n644 = local write "启用5"(w901) -> ()
        n645 = call <vilib>:"Close Config Data.vi"("error in (no error)"=w907, "refnum"=w908) -> ("error out"=w886:errorcluster, "file path"=w887:path)  [unwired: 8 in]
        n646 = Open/Create/Replace File(file path (use dialog)=w887, error in=w886) -> (refnum out=w889:refnum<file>, error out=w888:errorcluster)  [unwired: 4 in, 1 out]
        n647 = Flush File(refnum=w889, error in=w888) -> (refnum out=w890:refnum<file>, error out=w891:errorcluster)
        n648 = Close File(refnum=w890, error in=w891) -> ()  [unwired: 2 out]
      }
      event "选用水样": Value Change {
        (unwired) "浓度6" ("key")
        n649 = event-data() -> ()  [unwired: 1 in, 6 out]
        n650 = local read "量程选择"() -> (w1014:enum16{"低量程", "高量程", "0-2量程"})
        n651 = property on="窗格" class="Pane"("Origin"=T4 {"Horizontal"=0, "Vertical"=1300} ("原点")) -> ()  [unwired: 2 in, 2 out]
        n652 = case shown="\"葡萄糖\", 默认" "选用水样" {
          tunnel: ["葡萄糖标线" ("section") "草酸钠标线" ("section")] -> w1016
          frame "葡萄糖", Default {
          }
          frame "草酸钠" {
          }
        }
        n653 = global read "CODMN外部API.vi" "ping"() -> (w1000:bool)
        n654 = case shown="\"0-2量程\"" w1014 {
          tunnel: ["低量程" "高量程" "0-2量程"] -> w1015
          frame "低量程", Default {
          }
          frame "高量程" {
          }
          frame "0-2量程" {
          }
        }
        n655 = case shown="假" w1000 {
          tunnel: [w1069 w1072] -> w999
          frame False {
            n656 = global read "COD内部交互全局.vi" "配置文件ini"() -> (w1071:string)
            n657 = call <vilib>:"Application Directory.vi"() -> ("Application Directory"=w1070:path)
            n658 = Build Path(base path=w1070, name or relative path=w1071) -> (appended path=w1069:path)
          }
          frame True {
            n659 = global read "CODMN外部API.vi" "配置文件 path"() -> (w1072:path)
          }
        }
        n660 = Concatenate Strings(w1016, w1015) -> (w1013:string)
        n661 = call <vilib>:"Open Config Data.vi"("configuration file path"=w999) -> ("error out"=w995:errorcluster, "refnum"=w996:T6)  [unwired: 8 in, 1 out]
        n662 = call-poly <vilib>:"Write Key.vi"("section"="标线选择", "error in (no error)"=w995, "value"="选用水样", "key"="选用水样", "refnum"=w996) -> ("error out"=w992:errorcluster, "refnum out"=w993:T6)  [unwired: 4 in, 1 out]
        n663 = call-poly <vilib>:"Read Key.vi"("section"=w1013, "error in (no error)"=w992, "key"="浓度1", "refnum"=w993) -> ("error out"=w1039:errorcluster, "value"=w1037:dbl, "refnum out"=w1038:T6)  [unwired: 4 in, 1 out]
        n664 = local write "浓度1"(w1037) -> ()
        n665 = call-poly <vilib>:"Read Key.vi"("section"=w1013, "error in (no error)"=w1039, "key"="浓度2", "refnum"=w1038) -> ("error out"=w1053:errorcluster, "value"=w1040:dbl, "refnum out"=w1052:T6)  [unwired: 4 in, 1 out]
        n666 = local write "浓度2"(w1040) -> ()
        n667 = call-poly <vilib>:"Read Key.vi"("section"=w1013, "error in (no error)"=w1053, "key"="浓度3", "refnum"=w1052) -> ("error out"=w1054:errorcluster, "value"=w1042:dbl, "refnum out"=w1051:T6)  [unwired: 4 in, 1 out]
        n668 = local write "浓度3"(w1042) -> ()
        n669 = call-poly <vilib>:"Read Key.vi"("section"=w1013, "error in (no error)"=w1054, "key"="泵滴定数1", "refnum"=w1051) -> ("error out"=w1055:errorcluster, "value"=w1044:dbl, "refnum out"=w1050:T6)  [unwired: 4 in, 1 out]
        n670 = local write "泵滴定数1"(w1044) -> ()
        n671 = call-poly <vilib>:"Read Key.vi"("section"=w1013, "error in (no error)"=w1055, "key"="泵滴定数2", "refnum"=w1050) -> ("error out"=w1049:errorcluster, "value"=w1047:dbl, "refnum out"=w1056:T6)  [unwired: 4 in, 1 out]
        n672 = local write "泵滴定数2"(w1047) -> ()
        n673 = call-poly <vilib>:"Read Key.vi"("section"=w1013, "error in (no error)"=w1049, "key"="泵滴定数3", "refnum"=w1056) -> ("error out"=w1061:errorcluster, "value"=w1060:dbl, "refnum out"=w1057:T6)  [unwired: 4 in, 1 out]
        n674 = local write "泵滴定数3"(w1060) -> ()
        n675 = call-poly <vilib>:"Read Key.vi"("section"=w1013, "error in (no error)"=w1061, "key"="浓度4", "refnum"=w1057) -> ("error out"=w1062:errorcluster, "value"=w1008:dbl, "refnum out"=w1058:T6)  [unwired: 4 in, 1 out]
        n676 = local write "浓度4"(w1008) -> ()
        n677 = call-poly <vilib>:"Read Key.vi"("section"=w1013, "error in (no error)"=w1062, "key"="浓度5", "refnum"=w1058) -> ("error out"=w1011:errorcluster, "value"=w1007:dbl, "refnum out"=w1012:T6)  [unwired: 4 in, 1 out]
        n678 = local write "浓度5"(w1007) -> ()
        n679 = call-poly <vilib>:"Read Key.vi"("section"=w1013, "error in (no error)"=w1011, "key"="泵滴定数4", "refnum"=w1012) -> ("error out"=w1063:errorcluster, "value"=w1006:dbl, "refnum out"=w1059:T6)  [unwired: 4 in, 1 out]
        n680 = local write "泵滴定数4"(w1006) -> ()
        n681 = call-poly <vilib>:"Read Key.vi"("section"=w1013, "error in (no error)"=w1063, "key"="泵滴定数5", "refnum"=w1059) -> ("error out"=w1009:errorcluster, "value"=w1005:dbl, "refnum out"=w1010:T6)  [unwired: 4 in, 1 out]
        n682 = local write "泵滴定数5"(w1005) -> ()
        n683 = call-poly <vilib>:"Read Key.vi"("section"=w1013, "error in (no error)"=w1009, "key"="当前选用的校准", "refnum"=w1010) -> ("error out"=w1033:errorcluster, "refnum out"=w1034:T6)  [unwired: 4 in, 2 out]
        n684 = call-poly <vilib>:"Read Key.vi"("section"=w1013, "error in (no error)"=w1033, "key"="启用1", "refnum"=w1034) -> ("error out"=w1030:errorcluster, "value"=w1019:bool, "refnum out"=w1031:T6)  [unwired: 4 in, 1 out]
        n685 = local write "启用1"(w1019) -> ()
        n686 = call-poly <vilib>:"Read Key.vi"("section"=w1013, "error in (no error)"=w1030, "key"="启用2", "refnum"=w1031) -> ("error out"=w1028:errorcluster, "value"=w1018:bool, "refnum out"=w1029:T6)  [unwired: 4 in, 1 out]
        n687 = local write "启用2"(w1018) -> ()
        n688 = call-poly <vilib>:"Read Key.vi"("section"=w1013, "error in (no error)"=w1028, "key"="启用3", "refnum"=w1029) -> ("error out"=w1026:errorcluster, "value"=w1017:bool, "refnum out"=w1027:T6)  [unwired: 4 in, 1 out]
        n689 = local write "启用3"(w1017) -> ()
        n690 = call-poly <vilib>:"Read Key.vi"("section"=w1013, "error in (no error)"=w1026, "key"="启用4", "refnum"=w1027) -> ("error out"=w1024:errorcluster, "value"=w1002:bool, "refnum out"=w1025:T6)  [unwired: 4 in, 1 out]
        n691 = local write "启用4"(w1002) -> ()
        n692 = call-poly <vilib>:"Read Key.vi"("section"=w1013, "error in (no error)"=w1024, "key"="启用5", "refnum"=w1025) -> ("error out"=w1003:errorcluster, "value"=w1001:bool, "refnum out"=w1004:T6)  [unwired: 4 in, 1 out]
        n693 = local write "启用5"(w1001) -> ()
        n694 = call <vilib>:"Close Config Data.vi"("error in (no error)"=w1003, "refnum"=w1004) -> ("error out"=w986:errorcluster, "file path"=w987:path)  [unwired: 8 in]
        n695 = Open/Create/Replace File(file path (use dialog)=w987, error in=w986) -> (refnum out=w989:refnum<file>, error out=w988:errorcluster)  [unwired: 4 in, 1 out]
        n696 = Flush File(refnum=w989, error in=w988) -> (refnum out=w990:refnum<file>, error out=w991:errorcluster)
        n697 = Close File(refnum=w990, error in=w991) -> ()  [unwired: 2 out]
      }
      event "量程选择": Value Change {
        w1089 = "量程选择" ("section")
        n698 = event-data() -> ()  [unwired: 1 in, 6 out]
        n699 = local read "选用水样"() -> (w1107:enum16{"葡萄糖", "草酸钠"})
        n700 = property on="窗格" class="Pane"("Origin"=T4 {"Horizontal"=0, "Vertical"=1300} ("原点")) -> ()  [unwired: 2 in, 2 out]
        n701 = case shown="\"葡萄糖\", 默认" w1107 {
          tunnel: ["葡萄糖标线" ("section") "草酸钠标线" ("section")] -> w1106
          frame "葡萄糖", Default {
          }
          frame "草酸钠" {
          }
        }
        n702 = case shown="\"0-2量程\"" "量程选择" {
          tunnel: ["低量程" "高量程" "0-2量程"] -> w1104
          frame "低量程", Default {
          }
          frame "高量程" {
          }
          frame "0-2量程" {
          }
        }
        n703 = global read "CODMN外部API.vi" "ping"() -> (w1091:bool)
        n704 = case shown="假" w1091 {
          tunnel: [w1160 w1163] -> w1090
          frame False {
            n705 = global read "COD内部交互全局.vi" "配置文件ini"() -> (w1162:string)
            n706 = call <vilib>:"Application Directory.vi"() -> ("Application Directory"=w1161:path)
            n707 = Build Path(base path=w1161, name or relative path=w1162) -> (appended path=w1160:path)
          }
          frame True {
            n708 = global read "CODMN外部API.vi" "配置文件 path"() -> (w1163:path)
          }
        }
        n709 = Concatenate Strings(w1106, w1104) -> (w1105:string)
        n710 = call <vilib>:"Open Config Data.vi"("configuration file path"=w1090) -> ("error out"=w1088:errorcluster, "refnum"=w1087:T6)  [unwired: 8 in, 1 out]
        n711 = call-poly <vilib>:"Write Key.vi"("section"=w1089, "error in (no error)"=w1088, "value"="量程选择", "key"=w1089, "refnum"=w1087) -> ("error out"=w1084:errorcluster, "refnum out"=w1086:T6)  [unwired: 4 in, 1 out]
        n712 = call-poly <vilib>:"Read Key.vi"("section"=w1105, "error in (no error)"=w1084, "key"="浓度1", "refnum"=w1086) -> ("error out"=w1130:errorcluster, "value"=w1128:dbl, "refnum out"=w1129:T6)  [unwired: 4 in, 1 out]
        n713 = local write "浓度1"(w1128) -> ()
        n714 = call-poly <vilib>:"Read Key.vi"("section"=w1105, "error in (no error)"=w1130, "key"="浓度2", "refnum"=w1129) -> ("error out"=w1144:errorcluster, "value"=w1131:dbl, "refnum out"=w1143:T6)  [unwired: 4 in, 1 out]
        n715 = local write "浓度2"(w1131) -> ()
        n716 = call-poly <vilib>:"Read Key.vi"("section"=w1105, "error in (no error)"=w1144, "key"="浓度3", "refnum"=w1143) -> ("error out"=w1145:errorcluster, "value"=w1133:dbl, "refnum out"=w1142:T6)  [unwired: 4 in, 1 out]
        n717 = local write "浓度3"(w1133) -> ()
        n718 = call-poly <vilib>:"Read Key.vi"("section"=w1105, "error in (no error)"=w1145, "key"="泵滴定数1", "refnum"=w1142) -> ("error out"=w1146:errorcluster, "value"=w1135:dbl, "refnum out"=w1141:T6)  [unwired: 4 in, 1 out]
        n719 = local write "泵滴定数1"(w1135) -> ()
        n720 = call-poly <vilib>:"Read Key.vi"("section"=w1105, "error in (no error)"=w1146, "key"="泵滴定数2", "refnum"=w1141) -> ("error out"=w1140:errorcluster, "value"=w1138:dbl, "refnum out"=w1147:T6)  [unwired: 4 in, 1 out]
        n721 = local write "泵滴定数2"(w1138) -> ()
        n722 = call-poly <vilib>:"Read Key.vi"("section"=w1105, "error in (no error)"=w1140, "key"="泵滴定数3", "refnum"=w1147) -> ("error out"=w1152:errorcluster, "value"=w1151:dbl, "refnum out"=w1148:T6)  [unwired: 4 in, 1 out]
        n723 = local write "泵滴定数3"(w1151) -> ()
        n724 = call-poly <vilib>:"Read Key.vi"("section"=w1105, "error in (no error)"=w1152, "key"="浓度4", "refnum"=w1148) -> ("error out"=w1153:errorcluster, "value"=w1095:dbl, "refnum out"=w1149:T6)  [unwired: 4 in, 1 out]
        n725 = local write "浓度4"(w1095) -> ()
        n726 = call-poly <vilib>:"Read Key.vi"("section"=w1105, "error in (no error)"=w1153, "key"="浓度5", "refnum"=w1149) -> ("error out"=w1102:errorcluster, "value"=w1094:dbl, "refnum out"=w1103:T6)  [unwired: 4 in, 1 out]
        n727 = local write "浓度5"(w1094) -> ()
        n728 = call-poly <vilib>:"Read Key.vi"("section"=w1105, "error in (no error)"=w1102, "key"="泵滴定数4", "refnum"=w1103) -> ("error out"=w1154:errorcluster, "value"=w1093:dbl, "refnum out"=w1150:T6)  [unwired: 4 in, 1 out]
        n729 = local write "泵滴定数4"(w1093) -> ()
        n730 = call-poly <vilib>:"Read Key.vi"("section"=w1105, "error in (no error)"=w1154, "key"="泵滴定数5", "refnum"=w1150) -> ("error out"=w1100:errorcluster, "value"=w1092:dbl, "refnum out"=w1101:T6)  [unwired: 4 in, 1 out]
        n731 = local write "泵滴定数5"(w1092) -> ()
        n732 = call-poly <vilib>:"Read Key.vi"("section"=w1105, "error in (no error)"=w1100, "key"="当前选用的校准", "refnum"=w1101) -> ("error out"=w1124:errorcluster, "refnum out"=w1125:T6)  [unwired: 4 in, 2 out]
        n733 = call-poly <vilib>:"Read Key.vi"("section"=w1105, "error in (no error)"=w1124, "key"="启用1", "refnum"=w1125) -> ("error out"=w1121:errorcluster, "value"=w1110:bool, "refnum out"=w1122:T6)  [unwired: 4 in, 1 out]
        n734 = local write "启用1"(w1110) -> ()
        n735 = call-poly <vilib>:"Read Key.vi"("section"=w1105, "error in (no error)"=w1121, "key"="启用2", "refnum"=w1122) -> ("error out"=w1119:errorcluster, "value"=w1109:bool, "refnum out"=w1120:T6)  [unwired: 4 in, 1 out]
        n736 = local write "启用2"(w1109) -> ()
        n737 = call-poly <vilib>:"Read Key.vi"("section"=w1105, "error in (no error)"=w1119, "key"="启用3", "refnum"=w1120) -> ("error out"=w1117:errorcluster, "value"=w1108:bool, "refnum out"=w1118:T6)  [unwired: 4 in, 1 out]
        n738 = local write "启用3"(w1108) -> ()
        n739 = call-poly <vilib>:"Read Key.vi"("section"=w1105, "error in (no error)"=w1117, "key"="启用4", "refnum"=w1118) -> ("error out"=w1115:errorcluster, "value"=w1097:bool, "refnum out"=w1116:T6)  [unwired: 4 in, 1 out]
        n740 = local write "启用4"(w1097) -> ()
        n741 = call-poly <vilib>:"Read Key.vi"("section"=w1105, "error in (no error)"=w1115, "key"="启用5", "refnum"=w1116) -> ("error out"=w1098:errorcluster, "value"=w1096:bool, "refnum out"=w1099:T6)  [unwired: 4 in, 1 out]
        n742 = local write "启用5"(w1096) -> ()
        n743 = call <vilib>:"Close Config Data.vi"("error in (no error)"=w1098, "refnum"=w1099) -> ("error out"=w1078:errorcluster, "file path"=w1079:path)  [unwired: 8 in]
        n744 = Open/Create/Replace File(file path (use dialog)=w1079, error in=w1078) -> (refnum out=w1081:refnum<file>, error out=w1080:errorcluster)  [unwired: 4 in, 1 out]
        n745 = Flush File(refnum=w1081, error in=w1080) -> (refnum out=w1082:refnum<file>, error out=w1083:errorcluster)
        n746 = Close File(refnum=w1082, error in=w1083) -> ()  [unwired: 2 out]
      }
      event "返回": Value Change {
        w1190 = "CODMn" ("section")
        n747 = event-data() -> ()  [unwired: 1 in, 6 out]
        n748 = property on="窗格" class="Pane"("Origin"=T4 {"Horizontal"=0, "Vertical"=0} ("原点")) -> ()  [unwired: 2 in, 2 out]
        n749 = global read "CODMN外部API.vi" "ping"() -> (w1176:bool)
        n750 = case shown="假" w1176 {
          tunnel: [w1241 w1244] -> w1175
          frame False {
            n751 = global read "COD内部交互全局.vi" "配置文件ini"() -> (w1243:string)
            n752 = call <vilib>:"Application Directory.vi"() -> ("Application Directory"=w1242:path)
            n753 = Build Path(base path=w1242, name or relative path=w1243) -> (appended path=w1241:path)
          }
          frame True {
            n754 = global read "CODMN外部API.vi" "配置文件 path"() -> (w1244:path)
          }
        }
        n755 = call <vilib>:"Open Config Data.vi"("configuration file path"=w1175) -> ("error out"=w1239:errorcluster, "refnum"=w1240:T6)  [unwired: 8 in, 1 out]
        n756 = local read "浓度1"() -> (w1237:dbl)
        n757 = call-poly <vilib>:"Write Key.vi"("section"=w1190, "error in (no error)"=w1239, "value"=w1237, "key"="浓度1", "refnum"=w1240) -> ("error out"=w1236:errorcluster, "refnum out"=w1235:T6)  [unwired: 4 in, 1 out]
        n758 = local read "浓度2"() -> (w1221:dbl)
        n759 = call-poly <vilib>:"Write Key.vi"("section"=w1190, "error in (no error)"=w1236, "value"=w1221, "key"="浓度2", "refnum"=w1235) -> ("error out"=w1234:errorcluster, "refnum out"=w1233:T6)  [unwired: 4 in, 1 out]
        n760 = local read "浓度3"() -> (w1217:dbl)
        n761 = local read "泵滴定数1"() -> (w1215:dbl)
        n762 = call-poly <vilib>:"Write Key.vi"("section"=w1190, "error in (no error)"=w1234, "value"=w1217, "key"="浓度3", "refnum"=w1233) -> ("error out"=w1232:errorcluster, "refnum out"=w1231:T6)  [unwired: 4 in, 1 out]
        n763 = local read "泵滴定数2"() -> (w1213:dbl)
        n764 = call-poly <vilib>:"Write Key.vi"("section"=w1190, "error in (no error)"=w1232, "value"=w1215, "key"="泵滴定数1", "refnum"=w1231) -> ("error out"=w1230:errorcluster, "refnum out"=w1229:T6)  [unwired: 4 in, 1 out]
        n765 = local read "泵滴定数3"() -> (w1211:dbl)
        n766 = call-poly <vilib>:"Write Key.vi"("section"=w1190, "error in (no error)"=w1230, "value"=w1213, "key"="泵滴定数2", "refnum"=w1229) -> ("error out"=w1228:errorcluster, "refnum out"=w1227:T6)  [unwired: 4 in, 1 out]
        n767 = call-poly <vilib>:"Write Key.vi"("section"=w1190, "error in (no error)"=w1228, "value"=w1211, "key"="泵滴定数3", "refnum"=w1227) -> ("error out"=w1226:errorcluster, "refnum out"=w1225:T6)  [unwired: 4 in, 1 out]
        n768 = local read "浓度4"() -> (w1178:dbl)
        n769 = call-poly <vilib>:"Write Key.vi"("section"=w1190, "error in (no error)"=w1226, "value"=w1178, "key"="浓度4", "refnum"=w1225) -> ("error out"=w1219:errorcluster, "refnum out"=w1220:T6)  [unwired: 4 in, 1 out]
        n770 = local read "浓度5"() -> (w1177:dbl)
        n771 = local read "泵滴定数4"() -> (w1179:dbl)
        n772 = call-poly <vilib>:"Write Key.vi"("section"=w1190, "error in (no error)"=w1219, "value"=w1177, "key"="浓度5", "refnum"=w1220) -> ("error out"=w1187:errorcluster, "refnum out"=w1188:T6)  [unwired: 4 in, 1 out]
        n773 = local read "泵滴定数5"() -> (w1180:dbl)
        n774 = call-poly <vilib>:"Write Key.vi"("section"=w1190, "error in (no error)"=w1187, "value"=w1179, "key"="泵滴定数4", "refnum"=w1188) -> ("error out"=w1224:errorcluster, "refnum out"=w1223:T6)  [unwired: 4 in, 1 out]
        n775 = call-poly <vilib>:"Write Key.vi"("section"=w1190, "error in (no error)"=w1224, "value"=w1180, "key"="泵滴定数5", "refnum"=w1223) -> ("error out"=w1185:errorcluster, "refnum out"=w1186:T6)  [unwired: 4 in, 1 out]
        n776 = local read "启用1"() -> (w1199:bool)
        n777 = call-poly <vilib>:"Write Key.vi"("section"=w1190, "error in (no error)"=w1185, "value"=w1199, "key"="启用1", "refnum"=w1186) -> ("error out"=w1195:errorcluster, "refnum out"=w1198:T6)  [unwired: 4 in, 1 out]
        n778 = local read "启用2"() -> (w1196:bool)
        n779 = call-poly <vilib>:"Write Key.vi"("section"=w1190, "error in (no error)"=w1195, "value"=w1196, "key"="启用2", "refnum"=w1198) -> ("error out"=w1206:errorcluster, "refnum out"=w1205:T6)  [unwired: 4 in, 1 out]
        n780 = local read "启用3"() -> (w1194:bool)
        n781 = call-poly <vilib>:"Write Key.vi"("section"=w1190, "error in (no error)"=w1206, "value"=w1194, "key"="启用3", "refnum"=w1205) -> ("error out"=w1204:errorcluster, "refnum out"=w1203:T6)  [unwired: 4 in, 1 out]
        n782 = local read "启用4"() -> (w1182:bool)
        n783 = call-poly <vilib>:"Write Key.vi"("section"=w1190, "error in (no error)"=w1204, "value"=w1182, "key"="启用4", "refnum"=w1203) -> ("error out"=w1202:errorcluster, "refnum out"=w1201:T6)  [unwired: 4 in, 1 out]
        n784 = local read "启用5"() -> (w1181:bool)
        n785 = call-poly <vilib>:"Write Key.vi"("section"=w1190, "error in (no error)"=w1202, "value"=w1181, "key"="启用5", "refnum"=w1201) -> ("error out"=w1183:errorcluster, "refnum out"=w1184:T6)  [unwired: 4 in, 1 out]
        n786 = call <vilib>:"Close Config Data.vi"("error in (no error)"=w1183, "refnum"=w1184) -> ("error out"=w1169:errorcluster, "file path"=w1170:path)  [unwired: 8 in]
        n787 = Open/Create/Replace File(file path (use dialog)=w1170, error in=w1169) -> (refnum out=w1172:refnum<file>, error out=w1171:errorcluster)  [unwired: 4 in, 1 out]
        n788 = Flush File(refnum=w1172, error in=w1171) -> (refnum out=w1173:refnum<file>, error out=w1174:errorcluster)
        n789 = Close File(refnum=w1173, error in=w1174) -> ()  [unwired: 2 out]
      }
      event "关闭", "关闭 2", "关闭 3": Value Change {
        n790 = event-data() -> ()  [unwired: 1 in, 6 out]
        n791 = property on="窗格" class="Pane"("Origin"=T4 {"Horizontal"=0, "Vertical"=0} ("原点")) -> ()  [unwired: 2 in, 2 out]
      }
      event Application Instance Close {
        n792 = event-data() -> ()  [unwired: 1 in, 4 out]
      }
      event "时间校准": Value Change {
        n793 = event-data() -> ()  [unwired: 1 in, 6 out]
        n794 = Get Date/Time In Seconds() -> (seconds since 1Jan1904=w1254:timestamp)
        n795 = Build Array(w1254) -> (w1253:timestamp[])
        n796 = call "DateToHex.vi"("DATE"=w1253) -> ("数组"=w1251:u16[])  [unwired: 10 in]
        n797 = Insert Into Array(array=u16[] [1] ("values"), index=1 ("索引"), new element=w1251) -> (w1247:u16[])
        n798 = call "CODMnMB_api.vi"("STEP"=enum16{"open", "read", "write", "close"}."write", "values"=w1247, "starting address"=u16 4612) -> ("error out"=w1246:errorcluster)  [unwired: 6 in, 2 out]
        n799 = call <vilib>:"Clear Errors.vi"("error in (no error)"=w1246) -> ()  [unwired: 5 in, 2 out]
      }
      event "故障清除": Value Change {
        n800 = event-data() -> ()  [unwired: 1 in, 6 out]
        n801 = call "CODMnMB_api.vi"("STEP"=enum16{"open", "read", "write", "close"}."write", "values"=u16[] [1], "starting address"=u16 4611) -> ()  [unwired: 6 in, 3 out]
      }
      event "仪器参数": Value Change {
        n802 = event-data() -> ()  [unwired: 1 in, 6 out]
        n803 = global read "CODMn断电保存全局变量.vi" "CODMn仪器参数"() -> (w1258:T15)
        n804 = call "仪器参数设置.vi"("氨氮仪器参数"=w1258) -> ("仪器参数设置输出"=w1259:T16)  [unwired: 10 in]
        n805 = Unbundle By Name(w1259) -> ("确定"=w1260:bool)
        n806 = case shown="真" w1260 {
          tunnel: w1259 -> [_ w1262]
          tunnel: w1258 -> [_ w1261]
          frame False {
          }
          frame True {
            n807 = flat-sequence {
              tunnel: w1262 -> [w1279]
              tunnel: w1261 -> [w1278]
              frame #0 {
                n808 = Unbundle By Name(w1279) -> ("测量量程"=w1277:dbl, "测量精度"=w1276:dbl, "测量间隔"=w1275:dbl, "消解温度"=w1274:dbl, "消解时长"=w1273:dbl, "空白校准时间"=w1272:timestamp, "曲线截距"=w1271:dbl, "曲线斜率"=w1270:dbl, "测量检出限"=w1269:dbl, "测量信号值"=w1268:dbl, "线性相关系数"=w1267:dbl, "二次多项式系数"=w1266:dbl, "标样校准时间"=w1265:timestamp, "稀释倍数"=w1264:dbl)
                n809 = Bundle By Name(cluster=w1278, "测量量程"=w1277, "测量精度"=w1276, "测量间隔"=w1275, "消解温度"=w1274, "消解时长"=w1273, "空白校准时间"=w1272, "曲线截距"=w1271, "曲线斜率"=w1270, "测量检出限"=w1269, "测量信号值"=w1268, "线性相关系数"=w1267, "二次多项式系数"=w1266, "标样校准时间"=w1265, "稀释倍数"=w1264) -> (w1263:T15)
                n810 = global write "CODMn断电保存全局变量.vi" "CODMn仪器参数"(w1263) -> ()
              }
              frame #1 {
                n811 = call "配置文件保存.vi"() -> ()  [unwired: 12 in]
              }
            }
          }
        }
      }
      event "远程自动校准浓度", "远程校准量程": Value Change {
        n812 = event-data() -> ()  [unwired: 1 in, 6 out]
        n813 = flat-sequence {
          frame #0 {
            n814 = global write "CODMn断电保存全局变量.vi" "远程校准量程"("远程校准量程") -> ()
            n815 = global write "CODMn断电保存全局变量.vi" "远程自动校准浓度"("远程自动校准浓度") -> ()
          }
          frame #1 {
            n816 = call "配置文件保存.vi"() -> ()  [unwired: 12 in]
          }
        }
      }
      event "测量模式(公式)": Value Change {
        n817 = event-data() -> ()  [unwired: 1 in, 6 out]
        n818 = flat-sequence {
          frame #0 {
            n819 = global write "CODMn断电保存全局变量.vi" "测量模式(公式)"("测量模式(公式)") -> ()
          }
          frame #1 {
            n820 = call "配置文件保存.vi"() -> ()  [unwired: 12 in]
          }
        }
      }
      event "跨度量程选择", "跨度液浓度", "零点核查量程选择", "零点核查浓度", "标样浓度", "标样核查量程选择", "加标回收量程：": Value Change {
        n821 = event-data() -> ()  [unwired: 1 in, 6 out]
        n822 = flat-sequence {
          frame #0 {
            n823 = global write "CODMn断电保存全局变量.vi" "标样浓度"("标样浓度") -> ()
            n824 = global write "CODMn断电保存全局变量.vi" "零点核查浓度"("零点核查浓度") -> ()
            n825 = global write "CODMn断电保存全局变量.vi" "跨度液浓度"("跨度液浓度") -> ()
            n826 = global write "CODMn断电保存全局变量.vi" "CODMn跨度量程选择"("跨度量程选择") -> ()
            n827 = global write "CODMn断电保存全局变量.vi" "加标回收量程选择"("加标回收量程：") -> ()
            n828 = global write "CODMn断电保存全局变量.vi" "标样核查量程选择"("标样核查量程选择") -> ()
            n829 = global write "CODMn断电保存全局变量.vi" "零点核查量程选择"("零点核查量程选择") -> ()
          }
          frame #1 {
            n830 = call "配置文件保存.vi"() -> ()  [unwired: 12 in]
          }
        }
      }
      event "校准1", "校准2", "校准3", "校准4", "校准5": Value Change {
        n831 = event-data() -> ()  [unwired: 1 in, 6 out]
        n832 = flat-sequence {
          tunnel: w1293 -> [w1302]
          tunnel: [w1302] -> w1295
          tunnel: w1290 -> [w1301]
          tunnel: [w1301] -> w1292
          tunnel: w1295 -> [w1338]
          tunnel: [w1338] -> w1294
          tunnel: w1292 -> [w1337]
          tunnel: [w1337] -> w1291
          tunnel: w1294 -> [w1365]
          tunnel: w1291 -> [w1364]
          frame #0 {
            n833 = Build Array("校准1", "校准2", "校准3", "校准4", "校准5") -> (w1305:bool[])
            n834 = for {
              tunnel: w1305 -> [w1320] mode=indexing
              tunnel: [w1312] -> w1296
              i -> [w1313]
              n835 = case shown="4" w1313 {
                tunnel: ["浓度1" "浓度2" "浓度3" "浓度4" "浓度5"] -> w1316
                frame 0, Default {
                }
                frame 1 {
                }
                frame 2 {
                }
                frame 3 {
                }
                frame 4 {
                }
              }
              n836 = Multiply(x=w1316, y=100.0) -> (x*y=w1314:dbl)
              n837 = Insert Into Array(array=u16[] [] ("values"), index=0 ("索引"), new element=w1314) -> (w1317:u16[])
              n838 = case shown="真" w1320 {
                tunnel: w1317 -> [_ w1329]
                tunnel: w1313 -> [_ w1331]
                tunnel: [_ w1326] -> w1312
                frame False {
                }
                frame True {
                  n839 = Increment(x=w1331) -> (x+1=w1327:i32)
                  n840 = global write "COD内部交互全局.vi" "当前校准"(w1327) -> ()
                  n841 = call "CODMnMB_api.vi"("STEP"=enum16{"open", "read", "write", "close"}."write", "values"=w1329, "starting address"=u16 4274) -> ("error out"=w1326:errorcluster)  [unwired: 6 in, 2 out]
                }
              }
            }
            n842 = local read "量程选择"() -> (w1298:enum16{"低量程", "高量程", "0-2量程"})
            n843 = case shown="\"高量程\"" w1298 {
              tunnel: [u16[] [0] ("values") u16[] [1] ("values") u16[] [0] ("values")] -> w1297
              frame "低量程", Default {
              }
              frame "高量程" {
              }
              frame "0-2量程" {
              }
            }
            n844 = call "CODMnMB_api.vi"("STEP"=enum16{"open", "read", "write", "close"}."write", "Error in"=w1296, "values"=w1297, "starting address"=u16 4276) -> ()  [unwired: 5 in, 3 out]
          }
          frame #1 {
            n845 = global read "COD内部交互全局.vi" "当前校准"() -> (w1339:i32)
            n846 = case shown="5" w1339 {
              tunnel: [w1347 w1348 w1349 w1350 w1351] -> w1335
              frame 1, Default {
                n847 = local read "浓度1"() -> (w1347:dbl)
              }
              frame 2 {
                n848 = local read "浓度2"() -> (w1348:dbl)
              }
              frame 3 {
                n849 = local read "浓度3"() -> (w1349:dbl)
              }
              frame 4 {
                n850 = local read "浓度4"() -> (w1350:dbl)
              }
              frame 5 {
                n851 = local read "浓度5"() -> (w1351:dbl)
              }
            }
            n852 = Number To Decimal String(number=w1335) -> (decimal integer string=w1334:string)  [unwired: 1 in]
            n853 = Concatenate Strings("仪器校准中!\n当前校准浓度为:", w1334, "mg/L" ("字符串")) -> (w1332:string)
            n854 = Not Equal To 0?(x=w1335) -> (x != 0?=w1343:bool)
            n855 = global write "COD内部交互全局.vi" "校准内容显示"(w1332) -> ()
            n856 = case shown="真" w1343 {
              tunnel: [u16 8 ("address") u16 9 ("address")] -> w1346
              tunnel: ["校零" ("测量模式") "校标" ("测量模式")] -> _
              frame False {
              }
              frame True {
              }
            }
            n857 = Insert Into Array(array=u16[] [] ("values"), index=0 ("索引"), new element=w1346) -> (w1340:u16[])
            n858 = call "CODMnMB_api.vi"("STEP"=enum16{"open", "read", "write", "close"}."write", "values"=w1340, "starting address"=u16 4608 ("address")) -> ()  [unwired: 6 in, 3 out]
          }
          frame #2 {
            n859 = local read "选用水样"() -> (w1373:enum16{"葡萄糖", "草酸钠"})
            n860 = global read "CODMN外部API.vi" "ping"() -> (w1363:bool)
            n861 = case shown="假" w1363 {
              tunnel: [w1381 w1384] -> w1362
              frame False {
                n862 = global read "COD内部交互全局.vi" "配置文件ini"() -> (w1383:string)
                n863 = call <vilib>:"Application Directory.vi"() -> ("Application Directory"=w1382:path)
                n864 = Build Path(base path=w1382, name or relative path=w1383) -> (appended path=w1381:path)
              }
              frame True {
                n865 = global read "CODMN外部API.vi" "配置文件 path"() -> (w1384:path)
              }
            }
            n866 = local read "量程选择"() -> (w1372:enum16{"低量程", "高量程", "0-2量程"})
            n867 = case shown="\"葡萄糖\", 默认" w1373 {
              tunnel: ["葡萄糖标线" ("section") "草酸钠标线" ("section")] -> w1374
              frame "葡萄糖", Default {
              }
              frame "草酸钠" {
              }
            }
            n868 = Bundle By Name(cluster=cluster{"命令":string} {"命令"=""} ("元素"), "命令"="CODMn读取参数" ("名称（未命名）")) -> (w1369:cluster{"命令":string})
            n869 = case shown="\"0-2量程\"" w1372 {
              tunnel: ["低量程" "高量程" "0-2量程"] -> w1375
              frame "低量程", Default {
              }
              frame "高量程" {
              }
              frame "0-2量程" {
              }
            }
            n870 = global read "COD内部交互全局.vi" "当前校准"() -> (w1370:i32)
            n871 = Enqueue Element(queue=w1365, element=w1369, timeout in ms (-1)=1000 ("超时毫秒(-1)"), error in (no error)=w1364) -> ()  [unwired: 3 out]
            n872 = Concatenate Strings(w1374, w1375) -> (w1371:string)
            n873 = call <vilib>:"Open Config Data.vi"("configuration file path"=w1362) -> ("error out"=w1379:errorcluster, "refnum"=w1380:T6)  [unwired: 8 in, 1 out]
            n874 = call-poly <vilib>:"Write Key.vi"("section"=w1371, "error in (no error)"=w1379, "value"=w1370, "key"="当前选用的校准" ("section"), "refnum"=w1380) -> ("error out"=w1376:errorcluster, "refnum out"=w1377:T6)  [unwired: 4 in, 1 out]
            n875 = call <vilib>:"Close Config Data.vi"("error in (no error)"=w1376, "refnum"=w1377) -> ("error out"=w1356:errorcluster, "file path"=w1357:path)  [unwired: 8 in]
            n876 = Open/Create/Replace File(file path (use dialog)=w1357, error in=w1356) -> (refnum out=w1359:refnum<file>, error out=w1358:errorcluster)  [unwired: 4 in, 1 out]
            n877 = Flush File(refnum=w1359, error in=w1358) -> (refnum out=w1360:refnum<file>, error out=w1361:errorcluster)
            n878 = Close File(refnum=w1360, error in=w1361) -> ()  [unwired: 2 out]
          }
        }
      }
      event "水样量程选择:", "低切高阈值:", "高切低阈值:": Value Change {
        n879 = event-data() -> ()  [unwired: 1 in, 6 out]
        n880 = flat-sequence {
          frame #0 {
            n881 = global write "CODMn断电保存全局变量.vi" "高切低阈值:"("高切低阈值:") -> ()
            n882 = global write "CODMn断电保存全局变量.vi" "自动切换量程:"("水样量程选择:") -> ()
            n883 = global write "CODMn断电保存全局变量.vi" "低切高阈值:"("低切高阈值:") -> ()
          }
          frame #1 {
            n884 = call "配置文件保存.vi"() -> ()  [unwired: 12 in]
          }
        }
      }
      event "模型": Value Change {
        n885 = event-data() -> ()  [unwired: 1 in, 6 out]
        n886 = global read "CODMN外部API.vi" "ping"() -> (w1400:bool)
        n887 = case shown="假" w1400 {
          tunnel: [w1408 w1411] -> w1399
          frame False {
            n888 = global read "COD内部交互全局.vi" "配置文件ini"() -> (w1410:string)
            n889 = call <vilib>:"Application Directory.vi"() -> ("Application Directory"=w1409:path)
            n890 = Build Path(base path=w1409, name or relative path=w1410) -> (appended path=w1408:path)
          }
          frame True {
            n891 = global read "CODMN外部API.vi" "配置文件 path"() -> (w1411:path)
          }
        }
        n892 = call <vilib>:"Open Config Data.vi"("configuration file path"=w1399) -> ("error out"=w1406:errorcluster, "refnum"=w1407:T6)  [unwired: 8 in, 1 out]
        n893 = local read "模型"() -> (w1401:enum32{"线性", "多项式"})
        n894 = call-poly <vilib>:"Write Key.vi"("section"="CODMn模型选择" ("key"), "error in (no error)"=w1406, "value"=w1401, "key"="线性和多项式", "refnum"=w1407) -> ("error out"=w1402:errorcluster, "refnum out"=w1403:T6)  [unwired: 4 in, 1 out]
        n895 = call <vilib>:"Close Config Data.vi"("error in (no error)"=w1402, "refnum"=w1403) -> ("error out"=w1393:errorcluster, "file path"=w1394:path)  [unwired: 8 in]
        n896 = Open/Create/Replace File(file path (use dialog)=w1394, error in=w1393) -> (refnum out=w1396:refnum<file>, error out=w1395:errorcluster)  [unwired: 4 in, 1 out]
        n897 = Flush File(refnum=w1396, error in=w1395) -> (refnum out=w1397:refnum<file>, error out=w1398:errorcluster)
        n898 = Close File(refnum=w1397, error in=w1398) -> ()  [unwired: 2 out]
      }
      event "浓度1", "浓度2", "浓度3", "泵滴定数1", "泵滴定数2", "泵滴定数3", "启用1", "启用2", "启用3", "浓度4", "浓度5", "泵滴定数4", "泵滴定数5", "启用4", "启用5": Value Change {
        n899 = event-data() -> ()  [unwired: 1 in, 6 out]
        n900 = local read "选用水样"() -> (w1435:enum16{"葡萄糖", "草酸钠"})
        n901 = local read "量程选择"() -> (w1434:enum16{"低量程", "高量程", "0-2量程"})
        n902 = case shown="\"葡萄糖\", 默认" w1435 {
          tunnel: ["葡萄糖标线" ("section") "草酸钠标线" ("section")] -> w1441
          frame "葡萄糖", Default {
          }
          frame "草酸钠" {
          }
        }
        n903 = case shown="\"0-2量程\"" w1434 {
          tunnel: ["低量程" "高量程" "0-2量程"] -> w1432
          frame "低量程", Default {
          }
          frame "高量程" {
          }
          frame "0-2量程" {
          }
        }
        n904 = global read "CODMN外部API.vi" "ping"() -> (w1419:bool)
        n905 = case shown="假" w1419 {
          tunnel: [w1492 w1495] -> w1418
          frame False {
            n906 = global read "COD内部交互全局.vi" "配置文件ini"() -> (w1494:string)
            n907 = call <vilib>:"Application Directory.vi"() -> ("Application Directory"=w1493:path)
            n908 = Build Path(base path=w1493, name or relative path=w1494) -> (appended path=w1492:path)
          }
          frame True {
            n909 = global read "CODMN外部API.vi" "配置文件 path"() -> (w1495:path)
          }
        }
        n910 = Concatenate Strings(w1441, w1432) -> (w1433:string)
        n911 = call <vilib>:"Open Config Data.vi"("configuration file path"=w1418) -> ("error out"=w1490:errorcluster, "refnum"=w1491:T6)  [unwired: 8 in, 1 out]
        n912 = local read "浓度1"() -> (w1488:dbl)
        n913 = call-poly <vilib>:"Write Key.vi"("section"=w1433, "error in (no error)"=w1490, "value"=w1488, "key"="浓度1", "refnum"=w1491) -> ("error out"=w1487:errorcluster, "refnum out"=w1486:T6)  [unwired: 4 in, 1 out]
        n914 = local read "浓度2"() -> (w1472:dbl)
        n915 = call-poly <vilib>:"Write Key.vi"("section"=w1433, "error in (no error)"=w1487, "value"=w1472, "key"="浓度2", "refnum"=w1486) -> ("error out"=w1485:errorcluster, "refnum out"=w1484:T6)  [unwired: 4 in, 1 out]
        n916 = local read "浓度3"() -> (w1468:dbl)
        n917 = local read "泵滴定数1"() -> (w1466:dbl)
        n918 = call-poly <vilib>:"Write Key.vi"("section"=w1433, "error in (no error)"=w1485, "value"=w1468, "key"="浓度3", "refnum"=w1484) -> ("error out"=w1483:errorcluster, "refnum out"=w1482:T6)  [unwired: 4 in, 1 out]
        n919 = local read "泵滴定数2"() -> (w1464:dbl)
        n920 = call-poly <vilib>:"Write Key.vi"("section"=w1433, "error in (no error)"=w1483, "value"=w1466, "key"="泵滴定数1", "refnum"=w1482) -> ("error out"=w1481:errorcluster, "refnum out"=w1480:T6)  [unwired: 4 in, 1 out]
        n921 = local read "泵滴定数3"() -> (w1462:dbl)
        n922 = call-poly <vilib>:"Write Key.vi"("section"=w1433, "error in (no error)"=w1481, "value"=w1464, "key"="泵滴定数2", "refnum"=w1480) -> ("error out"=w1479:errorcluster, "refnum out"=w1478:T6)  [unwired: 4 in, 1 out]
        n923 = call-poly <vilib>:"Write Key.vi"("section"=w1433, "error in (no error)"=w1479, "value"=w1462, "key"="泵滴定数3", "refnum"=w1478) -> ("error out"=w1477:errorcluster, "refnum out"=w1476:T6)  [unwired: 4 in, 1 out]
        n924 = local read "浓度4"() -> (w1431:dbl)
        n925 = call-poly <vilib>:"Write Key.vi"("section"=w1433, "error in (no error)"=w1477, "value"=w1431, "key"="浓度4", "refnum"=w1476) -> ("error out"=w1470:errorcluster, "refnum out"=w1471:T6)  [unwired: 4 in, 1 out]
        n926 = local read "浓度5"() -> (w1430:dbl)
        n927 = local read "泵滴定数4"() -> (w1427:dbl)
        n928 = call-poly <vilib>:"Write Key.vi"("section"=w1433, "error in (no error)"=w1470, "value"=w1430, "key"="浓度5", "refnum"=w1471) -> ("error out"=w1428:errorcluster, "refnum out"=w1429:T6)  [unwired: 4 in, 1 out]
        n929 = local read "泵滴定数5"() -> (w1426:dbl)
        n930 = call-poly <vilib>:"Write Key.vi"("section"=w1433, "error in (no error)"=w1428, "value"=w1427, "key"="泵滴定数4", "refnum"=w1429) -> ("error out"=w1475:errorcluster, "refnum out"=w1474:T6)  [unwired: 4 in, 1 out]
        n931 = call-poly <vilib>:"Write Key.vi"("section"=w1433, "error in (no error)"=w1475, "value"=w1426, "key"="泵滴定数5", "refnum"=w1474) -> ("error out"=w1424:errorcluster, "refnum out"=w1425:T6)  [unwired: 4 in, 1 out]
        n932 = local read "启用1"() -> (w1450:bool)
        n933 = call-poly <vilib>:"Write Key.vi"("section"=w1433, "error in (no error)"=w1424, "value"=w1450, "key"="启用1", "refnum"=w1425) -> ("error out"=w1446:errorcluster, "refnum out"=w1449:T6)  [unwired: 4 in, 1 out]
        n934 = local read "启用2"() -> (w1447:bool)
        n935 = call-poly <vilib>:"Write Key.vi"("section"=w1433, "error in (no error)"=w1446, "value"=w1447, "key"="启用2", "refnum"=w1449) -> ("error out"=w1457:errorcluster, "refnum out"=w1456:T6)  [unwired: 4 in, 1 out]
        n936 = local read "启用3"() -> (w1445:bool)
        n937 = call-poly <vilib>:"Write Key.vi"("section"=w1433, "error in (no error)"=w1457, "value"=w1445, "key"="启用3", "refnum"=w1456) -> ("error out"=w1455:errorcluster, "refnum out"=w1454:T6)  [unwired: 4 in, 1 out]
        n938 = local read "启用4"() -> (w1420:bool)
        n939 = call-poly <vilib>:"Write Key.vi"("section"=w1433, "error in (no error)"=w1455, "value"=w1420, "key"="启用4", "refnum"=w1454) -> ("error out"=w1453:errorcluster, "refnum out"=w1452:T6)  [unwired: 4 in, 1 out]
        n940 = local read "启用5"() -> (w1421:bool)
        n941 = local read "选用水样"() -> (w1440:enum16{"葡萄糖", "草酸钠"})
        n942 = call-poly <vilib>:"Write Key.vi"("section"=w1433, "error in (no error)"=w1453, "value"=w1421, "key"="启用5", "refnum"=w1452) -> ("error out"=w1422:errorcluster, "refnum out"=w1423:T6)  [unwired: 4 in, 1 out]
        n943 = call-poly <vilib>:"Write Key.vi"("section"="标线选择", "error in (no error)"=w1422, "value"=w1440, "key"="选用水样", "refnum"=w1423) -> ("error out"=w1437:errorcluster, "refnum out"=w1438:T6)  [unwired: 4 in, 1 out]
        n944 = call <vilib>:"Close Config Data.vi"("error in (no error)"=w1437, "refnum"=w1438) -> ("error out"=w1412:errorcluster, "file path"=w1413:path)  [unwired: 8 in]
        n945 = Open/Create/Replace File(file path (use dialog)=w1413, error in=w1412) -> (refnum out=w1415:refnum<file>, error out=w1414:errorcluster)  [unwired: 4 in, 1 out]
        n946 = Flush File(refnum=w1415, error in=w1414) -> (refnum out=w1416:refnum<file>, error out=w1417:errorcluster)
        n947 = Close File(refnum=w1416, error in=w1417) -> ()  [unwired: 2 out]
      }
      event "读取": Value Change {
        (unwired) u16 94 ("number of holding registers")
        (unwired) u16 4616 ("starting address")
        n948 = event-data() -> ()  [unwired: 1 in, 6 out]
        n949 = Bundle By Name(cluster=cluster{"命令":string} {"命令"=""} ("元素"), "命令"="CODMn读取公式" ("名称（未命名）")) -> (w1501:cluster{"命令":string})
        n950 = Enqueue Element(queue=w1505, element=w1501, error in (no error)=w1504) -> ()  [unwired: 1 in, 3 out]
      }
      event "写入": Mouse Down {
        n951 = event-data() -> ()  [unwired: 1 in, 8 out]
        n952 = Two Button Dialog(message="是否将上方方程系数K、B、X^2的值写入，写入会覆盖原有公式！" ("消息")) -> (T button?=w1506:bool)  [unwired: 2 in]
        n953 = case shown="真" w1506 {
          frame False {
          }
          frame True {
            n954 = local read "测量模式(公式)"() -> (w1509:u16)
            n955 = local read "量程选择"() -> (w1508:enum16{"低量程", "高量程", "0-2量程"})
            n956 = local read "模型"() -> (w1519:enum32{"线性", "多项式"})
            n957 = case shown="\"线性\", 默认" w1519 {
              tunnel: [w1562 w1605] -> w1517
              tunnel: [w1561 w1604] -> w1516
              tunnel: w1509 -> [w1560 _]
              tunnel: w1508 -> [w1559 _]
              frame "线性", Default {
                (unwired) "线性" ("table输入")
                n958 = case shown="1" w1560 {
                  tunnel: [u16 4626 ("starting address") w1569 w1574 w1579 w1584 w1589 w1594 w1599] -> w1562
                  tunnel: w1559 -> [_ w1568 _ _ _ _ _ _]
                  frame 0, Default {
                  }
                  frame 1 {
                    n959 = case shown="\"低量程\", 默认" w1568 {
                      tunnel: [u16 4626 ("starting address") u16 4632 ("starting address") u16 4638 ("starting address")] -> w1569
                      frame "低量程", Default {
                      }
                      frame "高量程" {
                      }
                      frame "0-2量程" {
                      }
                    }
                  }
                  frame 2 {
                    n960 = local read "量程选择"() -> (w1573:enum16{"低量程", "高量程", "0-2量程"})
                    n961 = case shown="\"低量程\", 默认" w1573 {
                      tunnel: [u16 4638 ("starting address") u16 4644 ("starting address") u16 4638 ("starting address")] -> w1574
                      frame "低量程", Default {
                      }
                      frame "高量程" {
                      }
                      frame "0-2量程" {
                      }
                    }
                  }
                  frame 3 {
                    n962 = local read "量程选择"() -> (w1578:enum16{"低量程", "高量程", "0-2量程"})
                    n963 = case shown="\"低量程\", 默认" w1578 {
                      tunnel: [u16 4650 ("starting address") u16 4656 ("starting address") u16 4638 ("starting address")] -> w1579
                      frame "低量程", Default {
                      }
                      frame "高量程" {
                      }
                      frame "0-2量程" {
                      }
                    }
                  }
                  frame 4 {
                    n964 = local read "量程选择"() -> (w1583:enum16{"低量程", "高量程", "0-2量程"})
                    n965 = case shown="\"低量程\", 默认" w1583 {
                      tunnel: [u16 4662 ("starting address") u16 4668 ("starting address") u16 4638 ("starting address")] -> w1584
                      frame "低量程", Default {
                      }
                      frame "高量程" {
                      }
                      frame "0-2量程" {
                      }
                    }
                  }
                  frame 5 {
                    n966 = local read "量程选择"() -> (w1588:enum16{"低量程", "高量程", "0-2量程"})
                    n967 = case shown="\"低量程\", 默认" w1588 {
                      tunnel: [u16 4674 ("starting address") u16 4680 ("starting address") u16 4638 ("starting address")] -> w1589
                      frame "低量程", Default {
                      }
                      frame "高量程" {
                      }
                      frame "0-2量程" {
                      }
                    }
                  }
                  frame 6 {
                    n968 = local read "量程选择"() -> (w1593:enum16{"低量程", "高量程", "0-2量程"})
                    n969 = case shown="\"低量程\", 默认" w1593 {
                      tunnel: [u16 4686 ("starting address") u16 4692 ("starting address") u16 4638 ("starting address")] -> w1594
                      frame "低量程", Default {
                      }
                      frame "高量程" {
                      }
                      frame "0-2量程" {
                      }
                    }
                  }
                  frame 7 {
                    n970 = local read "量程选择"() -> (w1598:enum16{"低量程", "高量程", "0-2量程"})
                    n971 = case shown="\"低量程\", 默认" w1598 {
                      tunnel: [u16 4698 ("starting address") u16 4704 ("starting address") u16 4638 ("starting address")] -> w1599
                      frame "低量程", Default {
                      }
                      frame "高量程" {
                      }
                      frame "0-2量程" {
                      }
                    }
                  }
                }
                n972 = local read "K"() -> (w1566:dbl)
                n973 = local read "b"() -> (w1565:dbl)
                n974 = Build Array(w1566, w1565, 0.0 ("元素")) -> (w1564:dbl[])
                n975 = call "浮点转CDAB整形cod.vi"("浮点数"=w1564) -> ("CDAB整形输出"=w1561:u16[])  [unwired: 10 in]
              }
              frame "多项式" {
                (unwired) "多项式" ("table输入")
                # "b,k,c"
                n976 = local read "多项式系数"() -> (w1610:dbl[])
                n977 = local read "测量模式(公式)"() -> (w1606:u16)
                n978 = Index Array(array=w1610) -> (element #1=w1608:dbl, element #2=w1603:dbl, element #3=w1607:dbl)  [unwired: 3 in]
                n979 = case shown="1" w1606 {
                  tunnel: [u16 4626 ("starting address") w1613 w1618 w1623 w1628 w1633 w1638 w1643] -> w1605
                  frame 0, Default {
                  }
                  frame 1 {
                    n980 = local read "量程选择"() -> (w1612:enum16{"低量程", "高量程", "0-2量程"})
                    n981 = case shown="\"低量程\", 默认" w1612 {
                      tunnel: [u16 4626 ("starting address") u16 4632 ("starting address") u16 4638 ("starting address")] -> w1613
                      frame "低量程", Default {
                      }
                      frame "高量程" {
                      }
                      frame "0-2量程" {
                      }
                    }
                  }
                  frame 2 {
                    n982 = local read "量程选择"() -> (w1617:enum16{"低量程", "高量程", "0-2量程"})
                    n983 = case shown="\"低量程\", 默认" w1617 {
                      tunnel: [u16 4638 ("starting address") u16 4644 ("starting address") u16 4638 ("starting address")] -> w1618
                      frame "低量程", Default {
                      }
                      frame "高量程" {
                      }
                      frame "0-2量程" {
                      }
                    }
                  }
                  frame 3 {
                    n984 = local read "量程选择"() -> (w1622:enum16{"低量程", "高量程", "0-2量程"})
                    n985 = case shown="\"低量程\", 默认" w1622 {
                      tunnel: [u16 4650 ("starting address") u16 4656 ("starting address") u16 4638 ("starting address")] -> w1623
                      frame "低量程", Default {
                      }
                      frame "高量程" {
                      }
                      frame "0-2量程" {
                      }
                    }
                  }
                  frame 4 {
                    n986 = local read "量程选择"() -> (w1627:enum16{"低量程", "高量程", "0-2量程"})
                    n987 = case shown="\"低量程\", 默认" w1627 {
                      tunnel: [u16 4662 ("starting address") u16 4668 ("starting address") u16 4638 ("starting address")] -> w1628
                      frame "低量程", Default {
                      }
                      frame "高量程" {
                      }
                      frame "0-2量程" {
                      }
                    }
                  }
                  frame 5 {
                    n988 = local read "量程选择"() -> (w1632:enum16{"低量程", "高量程", "0-2量程"})
                    n989 = case shown="\"低量程\", 默认" w1632 {
                      tunnel: [u16 4674 ("starting address") u16 4680 ("starting address") u16 4638 ("starting address")] -> w1633
                      frame "低量程", Default {
                      }
                      frame "高量程" {
                      }
                      frame "0-2量程" {
                      }
                    }
                  }
                  frame 6 {
                    n990 = local read "量程选择"() -> (w1637:enum16{"低量程", "高量程", "0-2量程"})
                    n991 = case shown="\"低量程\", 默认" w1637 {
                      tunnel: [u16 4686 ("starting address") u16 4692 ("starting address") u16 4638 ("starting address")] -> w1638
                      frame "低量程", Default {
                      }
                      frame "高量程" {
                      }
                      frame "0-2量程" {
                      }
                    }
                  }
                  frame 7 {
                    n992 = local read "量程选择"() -> (w1642:enum16{"低量程", "高量程", "0-2量程"})
                    n993 = case shown="\"低量程\", 默认" w1642 {
                      tunnel: [u16 4698 ("starting address") u16 4704 ("starting address") u16 4638 ("starting address")] -> w1643
                      frame "低量程", Default {
                      }
                      frame "高量程" {
                      }
                      frame "0-2量程" {
                      }
                    }
                  }
                }
                n994 = Build Array(w1603, w1608, w1607) -> (w1609:dbl[])
                n995 = call "浮点转CDAB整形cod.vi"("浮点数"=w1609) -> ("CDAB整形输出"=w1604:u16[])  [unwired: 10 in]
              }
            }
            n996 = local read "多项式系数"() -> (w1513:dbl[])
            n997 = call "CODMnMB_api.vi"("STEP"=enum16{"open", "read", "write", "close"}."write", "values"=w1516, "starting address"=w1517) -> ("error out"=w1515:errorcluster)  [unwired: 6 in, 2 out]
            n998 = Index Array(array=w1513) -> (element #1=w1512:dbl, element #2=w1511:dbl, element #3=w1510:dbl)  [unwired: 3 in]
            n999 = case shown="无错误" w1515 {
              tunnel: ["写入成功！" "写入失败！"] -> w1514
              tunnel: w1512 -> [w1520 _]
              tunnel: w1511 -> [w1521 _]
              tunnel: w1510 -> [w1522 _]
              tunnel: w1509 -> [w1527 _]
              tunnel: w1508 -> [w1526 _]
              frame No Error {
                w1529 = u16 1 items=["水样测试"=1, "标样核查"=2, "零点核查"=3, "跨度核查"=4, "空白测试"=5, "平行样"=6, "加标回收"=7] ("测量模式(公式)")
                n1000 = Number To Fractional String(number=w1520) -> (F-format string=w1531:string)  [unwired: 3 in]
                n1001 = Number To Fractional String(number=w1521) -> (F-format string=w1532:string)  [unwired: 3 in]
                n1002 = Number To Fractional String(number=w1522) -> (F-format string=w1530:string)  [unwired: 3 in]
                n1003 = property on="模型" class="Enum (严格)"() -> ("RingText.Text"=w1542:string)  [unwired: 2 in, 2 out]
                n1004 = property on="测量模式(公式)" class="Ring (严格)"() -> ("RingText.Text"=w1541:string)  [unwired: 2 in, 2 out]
                n1005 = property on="量程选择" class="Enum (严格)"() -> ("RingText.Text"=w1540:string)  [unwired: 2 in, 2 out]
                n1006 = Concatenate Strings("变更后:" ("table输入"), "K:" ("字符串"), w1532, "B:" ("字符串"), w1531, "X^2:" ("字符串"), w1530) -> (w1533:string)
                n1007 = Concatenate Strings(w1542, w1541, w1540, "公式改变" ("日志信息")) -> (w1534:string)
                n1008 = Equal?(x=w1527, y=w1529) -> (x = y?=w1525:bool)
                n1009 = Equal?(x=w1526, y=enum16{"低量程", "高量程", "0-2量程"}."低量程" ("量程选择")) -> (x = y?=w1524:bool)
                n1010 = Compound Arithmetic op=AND ("复合运算")(w1525, w1524) -> (w1523:bool)
                n1011 = case shown="真" w1523 {
                  tunnel: w1521 -> [_ w1555]
                  tunnel: w1520 -> [_ w1554]
                  tunnel: w1522 -> [_ w1553]
                  frame False {
                  }
                  frame True {
                    n1012 = global read "CODMn断电保存全局变量.vi" "CODMn仪器参数"() -> (w1556:T15)
                    n1013 = Bundle By Name(cluster=w1556, "曲线截距"=w1554, "曲线斜率"=w1555, "二次多项式系数"=w1553) -> (w1557:T15)
                    n1014 = global write "CODMn断电保存全局变量.vi" "CODMn仪器参数"(w1557) -> ()
                  }
                }
                n1015 = Get Date/Time In Seconds() -> (seconds since 1Jan1904=w1546:timestamp)
                n1016 = Bundle(cluster=T14 {"时间标识"=timestamp(0 s since 1904-01-01), "参数"="", "日志信息"="", "流程参数"=""} ("data in"), "时间标识"=w1546, "参数"="CODMn" ("table输入"), "日志信息"=w1534, "流程参数"=w1533) -> (w1544:T14)
                n1017 = call "流程日志字段定义.vi"("table输入"="操作日志", "data in"=w1544) -> ("table输出"=w1549:string, "columns"=w1550:string[], "data out"=w1551:T17)  [unwired: 7 in]
                n1018 = call "插入数据.vi"("data"=w1551, "columns"=w1550, "database"="database3.mdb", "table"=w1549) -> ()  [unwired: 7 in, 1 out]
              }
              frame Error {
              }
            }
            n1019 = One Button Dialog(message=w1514) -> ()  [unwired: 1 in, 1 out]
          }
        }
      }
      event "一键写入": Value Change {
        n1020 = event-data() -> ()  [unwired: 1 in, 6 out]
        n1021 = Two Button Dialog(message="确认是否写入公式，写入会覆盖原有公式！" ("消息")) -> (T button?=w1647:bool)  [unwired: 2 in]
        n1022 = case shown="真" w1647 {
          frame False {
          }
          frame True {
            n1023 = local read "模型"() -> (w1651:enum32{"线性", "多项式"})
            n1024 = case shown="\"线性\", 默认" w1651 {
              tunnel: [w1682 w1733] -> w1649
              frame "线性", Default {
                n1025 = property on="测量模式(公式)" class="Ring (严格)"() -> ("NumItems"=w1683:u32)  [unwired: 2 in, 2 out]
                n1026 = for {
                  N: w1683 -> [_]
                  tunnel: [w1684] -> w1682
                  i -> [w1689]
                  n1027 = Increment(x=w1689) -> (x+1=w1688:i32)
                  n1028 = local read "K"() -> (w1693:dbl)
                  n1029 = local read "b"() -> (w1694:dbl)
                  n1030 = case shown="1" w1688 {
                    tunnel: [u16 4626 ("starting address") w1699 w1704 w1709 w1714 w1719 w1724 w1729] -> w1686
                    frame 0, Default {
                    }
                    frame 1 {
                      n1031 = local read "量程选择"() -> (w1698:enum16{"低量程", "高量程", "0-2量程"})
                      n1032 = case shown="\"低量程\", 默认" w1698 {
                        tunnel: [u16 4626 ("starting address") u16 4632 ("starting address") u16 4638 ("starting address")] -> w1699
                        frame "低量程", Default {
                        }
                        frame "高量程" {
                        }
                        frame "0-2量程" {
                        }
                      }
                    }
                    frame 2 {
                      n1033 = local read "量程选择"() -> (w1703:enum16{"低量程", "高量程", "0-2量程"})
                      n1034 = case shown="\"低量程\", 默认" w1703 {
                        tunnel: [u16 4638 ("starting address") u16 4644 ("starting address") u16 4638 ("starting address")] -> w1704
                        frame "低量程", Default {
                        }
                        frame "高量程" {
                        }
                        frame "0-2量程" {
                        }
                      }
                    }
                    frame 3 {
                      n1035 = local read "量程选择"() -> (w1708:enum16{"低量程", "高量程", "0-2量程"})
                      n1036 = case shown="\"低量程\", 默认" w1708 {
                        tunnel: [u16 4650 ("starting address") u16 4656 ("starting address") u16 4638 ("starting address")] -> w1709
                        frame "低量程", Default {
                        }
                        frame "高量程" {
                        }
                        frame "0-2量程" {
                        }
                      }
                    }
                    frame 4 {
                      n1037 = local read "量程选择"() -> (w1713:enum16{"低量程", "高量程", "0-2量程"})
                      n1038 = case shown="\"高量程\"" w1713 {
                        tunnel: [u16 4662 ("starting address") u16 4668 ("starting address") u16 4638 ("starting address")] -> w1714
                        frame "低量程", Default {
                        }
                        frame "高量程" {
                        }
                        frame "0-2量程" {
                        }
                      }
                    }
                    frame 5 {
                      n1039 = local read "量程选择"() -> (w1718:enum16{"低量程", "高量程", "0-2量程"})
                      n1040 = case shown="\"低量程\", 默认" w1718 {
                        tunnel: [u16 4674 ("starting address") u16 4680 ("starting address") u16 4638 ("starting address")] -> w1719
                        frame "低量程", Default {
                        }
                        frame "高量程" {
                        }
                        frame "0-2量程" {
                        }
                      }
                    }
                    frame 6 {
                      n1041 = local read "量程选择"() -> (w1723:enum16{"低量程", "高量程", "0-2量程"})
                      n1042 = case shown="\"低量程\", 默认" w1723 {
                        tunnel: [u16 4686 ("starting address") u16 4692 ("starting address") u16 4638 ("starting address")] -> w1724
                        frame "低量程", Default {
                        }
                        frame "高量程" {
                        }
                        frame "0-2量程" {
                        }
                      }
                    }
                    frame 7 {
                      n1043 = local read "量程选择"() -> (w1728:enum16{"低量程", "高量程", "0-2量程"})
                      n1044 = case shown="\"低量程\", 默认" w1728 {
                        tunnel: [u16 4698 ("starting address") u16 4704 ("starting address") u16 4638 ("starting address")] -> w1729
                        frame "低量程", Default {
                        }
                        frame "高量程" {
                        }
                        frame "0-2量程" {
                        }
                      }
                    }
                  }
                  n1045 = Build Array(w1693, w1694, 0.0 ("元素")) -> (w1695:dbl[])
                  n1046 = call "浮点转CDAB整形cod.vi"("浮点数"=w1695) -> ("CDAB整形输出"=w1692:u16[])  [unwired: 10 in]
                  n1047 = Insert Into Array(array=u16[] [], index=0 ("索引"), new element=w1692) -> (w1685:u16[])
                  n1048 = call "CODMnMB_api.vi"("STEP"=enum16{"open", "read", "write", "close"}."write", "values"=w1685, "starting address"=w1686) -> ("error out"=w1684:errorcluster)  [unwired: 6 in, 2 out]
                }
              }
              frame "多项式" {
                # "b,k,c"
                n1049 = property on="测量模式(公式)" class="Ring (严格)"() -> ("NumItems"=w1734:u32)  [unwired: 2 in, 2 out]
                n1050 = for {
                  N: w1734 -> [_]
                  tunnel: [w1735] -> w1733
                  i -> [w1740]
                  n1051 = Increment(x=w1740) -> (x+1=w1739:i32)
                  n1052 = local read "多项式系数"() -> (w1744:dbl[])
                  n1053 = case shown="2" w1739 {
                    tunnel: [u16 4626 ("starting address") w1751 w1756 w1761 w1766 w1771 w1776 w1781] -> w1736
                    frame 0, Default {
                    }
                    frame 1 {
                      n1054 = local read "量程选择"() -> (w1750:enum16{"低量程", "高量程", "0-2量程"})
                      n1055 = case shown="\"低量程\", 默认" w1750 {
                        tunnel: [u16 4626 ("starting address") u16 4632 ("starting address") u16 4638 ("starting address")] -> w1751
                        frame "低量程", Default {
                        }
                        frame "高量程" {
                        }
                        frame "0-2量程" {
                        }
                      }
                    }
                    frame 2 {
                      n1056 = local read "量程选择"() -> (w1755:enum16{"低量程", "高量程", "0-2量程"})
                      n1057 = case shown="\"低量程\", 默认" w1755 {
                        tunnel: [u16 4638 ("starting address") u16 4644 ("starting address") u16 4638 ("starting address")] -> w1756
                        frame "低量程", Default {
                        }
                        frame "高量程" {
                        }
                        frame "0-2量程" {
                        }
                      }
                    }
                    frame 3 {
                      n1058 = local read "量程选择"() -> (w1760:enum16{"低量程", "高量程", "0-2量程"})
                      n1059 = case shown="\"低量程\", 默认" w1760 {
                        tunnel: [u16 4650 ("starting address") u16 4656 ("starting address") u16 4638 ("starting address")] -> w1761
                        frame "低量程", Default {
                        }
                        frame "高量程" {
                        }
                        frame "0-2量程" {
                        }
                      }
                    }
                    frame 4 {
                      n1060 = local read "量程选择"() -> (w1765:enum16{"低量程", "高量程", "0-2量程"})
                      n1061 = case shown="\"低量程\", 默认" w1765 {
                        tunnel: [u16 4662 ("starting address") u16 4668 ("starting address") u16 4638 ("starting address")] -> w1766
                        frame "低量程", Default {
                        }
                        frame "高量程" {
                        }
                        frame "0-2量程" {
                        }
                      }
                    }
                    frame 5 {
                      n1062 = local read "量程选择"() -> (w1770:enum16{"低量程", "高量程", "0-2量程"})
                      n1063 = case shown="\"低量程\", 默认" w1770 {
                        tunnel: [u16 4674 ("starting address") u16 4680 ("starting address") u16 4638 ("starting address")] -> w1771
                        frame "低量程", Default {
                        }
                        frame "高量程" {
                        }
                        frame "0-2量程" {
                        }
                      }
                    }
                    frame 6 {
                      n1064 = local read "量程选择"() -> (w1775:enum16{"低量程", "高量程", "0-2量程"})
                      n1065 = case shown="\"低量程\", 默认" w1775 {
                        tunnel: [u16 4686 ("starting address") u16 4692 ("starting address") u16 4638 ("starting address")] -> w1776
                        frame "低量程", Default {
                        }
                        frame "高量程" {
                        }
                        frame "0-2量程" {
                        }
                      }
                    }
                    frame 7 {
                      n1066 = local read "量程选择"() -> (w1780:enum16{"低量程", "高量程", "0-2量程"})
                      n1067 = case shown="\"低量程\", 默认" w1780 {
                        tunnel: [u16 4698 ("starting address") u16 4704 ("starting address") u16 4638 ("starting address")] -> w1781
                        frame "低量程", Default {
                        }
                        frame "高量程" {
                        }
                        frame "0-2量程" {
                        }
                      }
                    }
                  }
                  n1068 = Index Array(array=w1744) -> (element #1=w1747:dbl, element #2=w1746:dbl, element #3=w1748:dbl)  [unwired: 3 in]
                  n1069 = Build Array(w1746, w1747, w1748) -> (w1745:dbl[])
                  n1070 = call "浮点转CDAB整形cod.vi"("浮点数"=w1745) -> ("CDAB整形输出"=w1743:u16[])  [unwired: 10 in]
                  n1071 = Insert Into Array(array=u16[] [], index=0 ("索引"), new element=w1743) -> (w1737:u16[])
                  n1072 = call "CODMnMB_api.vi"("STEP"=enum16{"open", "read", "write", "close"}."write", "values"=w1737, "starting address"=w1736) -> ("error out"=w1735:errorcluster)  [unwired: 6 in, 2 out]
                }
              }
            }
            n1073 = case shown="无错误" w1649 {
              tunnel: ["写入成功！" "写入失败！"] -> w1650
              frame No Error {
                n1074 = local read "多项式系数"() -> (w1657:dbl[])
                n1075 = Index Array(array=w1657) -> (element #1=w1654:dbl, element #2=w1653:dbl, element #3=w1652:dbl)  [unwired: 3 in]
                n1076 = Number To Fractional String(number=w1654) -> (F-format string=w1660:string)  [unwired: 3 in]
                n1077 = Number To Fractional String(number=w1653) -> (F-format string=w1661:string)  [unwired: 3 in]
                n1078 = Number To Fractional String(number=w1652) -> (F-format string=w1659:string)  [unwired: 3 in]
                n1079 = property on="模型" class="Enum (严格)"() -> ("RingText.Text"=w1670:string)  [unwired: 2 in, 2 out]
                n1080 = property on="量程选择" class="Enum (严格)"() -> ("RingText.Text"=w1669:string)  [unwired: 2 in, 2 out]
                n1081 = Concatenate Strings("变更后:" ("table输入"), "K:" ("字符串"), w1661, "B:" ("字符串"), w1660, "X^2:" ("字符串"), w1659) -> (w1662:string)
                n1082 = global read "CODMn断电保存全局变量.vi" "CODMn仪器参数"() -> (w1655:T15)
                n1083 = Concatenate Strings(w1670, "【一键写入全部模式】" ("日志信息"), w1669, "公式改变" ("日志信息")) -> (w1663:string)
                n1084 = Get Date/Time In Seconds() -> (seconds since 1Jan1904=w1674:timestamp)
                n1085 = Bundle By Name(cluster=w1655, "曲线截距"=w1654, "曲线斜率"=w1653, "二次多项式系数"=w1652) -> (w1656:T15)
                n1086 = Bundle(cluster=T14 {"时间标识"=timestamp(0 s since 1904-01-01), "参数"="", "日志信息"="", "流程参数"=""} ("data in"), "时间标识"=w1674, "参数"="CODMn" ("table输入"), "日志信息"=w1663, "流程参数"=w1662) -> (w1672:T14)
                n1087 = global write "CODMn断电保存全局变量.vi" "CODMn仪器参数"(w1656) -> ()
                n1088 = call "流程日志字段定义.vi"("table输入"="操作日志", "data in"=w1672) -> ("table输出"=w1677:string, "columns"=w1678:string[], "data out"=w1679:T17)  [unwired: 7 in]
                n1089 = call "插入数据.vi"("data"=w1679, "columns"=w1678, "database"="database3.mdb", "table"=w1677) -> ()  [unwired: 7 in, 1 out]
              }
              frame Error {
              }
            }
            n1090 = One Button Dialog(message=w1650) -> ()  [unwired: 1 in, 1 out]
          }
        }
      }
      event "滴定曲线": Value Change {
        n1091 = event-data() -> ()  [unwired: 1 in, 6 out]
        n1092 = property on="窗格" class="Pane"("Origin"=T4 {"Horizontal"=0, "Vertical"=3200} ("原点")) -> ()  [unwired: 2 in, 2 out]
      }
      event "历史波形": Value Change {
        n1093 = event-data() -> ()  [unwired: 1 in, 6 out]
        n1094 = call-poly <vilib>:"Read Waveforms from File.vi"() -> ("error out"=w1786:errorcluster, "first waveform in record"=w1787:waveform(dbl))  [unwired: 6 in, 2 out]
        n1095 = case shown="无错误" w1786 {
          tunnel: w1787 -> [w1790 _]
          frame No Error {
            n1096 = Unbundle By Name(w1790) -> ("t0"=w1788:timestamp, "Y"=w1789:dbl[])  [unwired: 2 out]
            n1097 = global write "COD内部交互全局.vi" "波形时间"(w1788) -> ()
            n1098 = global write "COD内部交互全局.vi" "ORP滴定曲线"(w1789) -> ()
            n1099 = global write "COD内部交互全局.vi" "滴定数-ORP值"(w1789) -> ()
          }
          frame Error {
            n1100 = One Button Dialog(message="打开失败" ("消息")) -> ()  [unwired: 1 in, 1 out]
          }
        }
      }
      event "释放串口": Value Change {
        n1101 = event-data() -> ()  [unwired: 1 in, 6 out]
        n1102 = Two Button Dialog(message="确认是否释放串口，释放串口将导致通信失败！" ("消息")) -> (T button?=w1792:bool)  [unwired: 2 in]
        n1103 = case shown="真" w1792 {
          tunnel: w1795 -> [_ w1797]
          tunnel: w1794 -> [_ w1796]
          frame False {
          }
          frame True {
            n1104 = Bundle By Name(cluster=cluster{"命令":string} {"命令"=""} ("元素"), "命令"="停用模块" ("名称（未命名）")) -> (w1798:cluster{"命令":string})
            n1105 = Enqueue Element(queue=w1797, element=w1798, error in (no error)=w1796) -> ()  [unwired: 1 in, 3 out]
          }
        }
      }
      event "打开串口": Value Change {
        n1106 = event-data() -> ()  [unwired: 1 in, 6 out]
        n1107 = flat-sequence {
          tunnel: w1802 -> [w1810]
          tunnel: w1801 -> [w1809]
          frame #0 {
            n1108 = global read "CODMn断电保存全局变量.vi" "VISA resource name"() -> (w1813:refnum<visa-resource-name>)
            n1109 = global read "CODMn断电保存全局变量.vi" "MB通信方式选择"() -> (w1806:enum16{"串口", "TCP"})
            n1110 = global read "CODMn断电保存全局变量.vi" "PORT"() -> (w1804:string)
            n1111 = global read "CODMn断电保存全局变量.vi" "IP"() -> (w1805:string)
            n1112 = call "串口配置.vi"("PORT"=w1804, "IP"=w1805, "MB通信方式选择"=w1806, "请选择串口:"=w1813) -> ("PORT 2"=w1807:string, "IP 2"=w1808:string, "确认 2"=w1811:bool, "VISA资源名称 2"=w1812:refnum<visa-resource-name>, "MB通信方式选择 2"=w1803:enum16{"串口", "TCP"})  [unwired: 3 in]
            n1113 = case shown="真" w1811 {
              tunnel: w1812 -> [_ w1822]
              tunnel: w1810 -> [_ w1818]
              tunnel: w1809 -> [_ w1817]
              tunnel: w1808 -> [_ w1816]
              tunnel: w1807 -> [_ w1815]
              tunnel: w1803 -> [_ w1814]
              frame False {
              }
              frame True {
                n1114 = global write "CODMn断电保存全局变量.vi" "IP"(w1816) -> ()
                n1115 = global write "CODMn断电保存全局变量.vi" "PORT"(w1815) -> ()
                n1116 = global write "CODMn断电保存全局变量.vi" "VISA resource name"(w1822) -> ()
                n1117 = global write "CODMn断电保存全局变量.vi" "MB通信方式选择"(w1814) -> ()
                n1118 = Bundle By Name(cluster=cluster{"命令":string} {"命令"=""} ("元素"), "命令"="启用模块" ("名称（未命名）")) -> (w1819:cluster{"命令":string})
                n1119 = Enqueue Element(queue=w1818, element=w1819, error in (no error)=w1817) -> ()  [unwired: 1 in, 3 out]
              }
            }
          }
          frame #1 {
            n1120 = call "配置文件保存.vi"() -> ()  [unwired: 12 in]
          }
        }
      }
      event "更新程序": Value Change {
        n1121 = event-data() -> ("CtlRef"=w1825:refnum<vi>, "NewVal"=w1826:bool)  [unwired: 1 in, 4 out]
        n1122 = case shown="真" w1826 {
          tunnel: w1825 -> [_ w1835]
          tunnel: w1824 -> [w1828 w1834]
          tunnel: w1823 -> [w1827 w1833]
          frame False {
            n1123 = Bundle By Name(cluster=cluster{"命令":string} {"命令"=""} ("元素"), "命令"="启用模块" ("名称（未命名）")) -> (w1829:cluster{"命令":string})
            n1124 = Enqueue Element(queue=w1828, element=w1829, error in (no error)=w1827) -> ()  [unwired: 1 in, 3 out]
          }
          frame True {
            n1125 = Two Button Dialog(message="警告，非专业人士请勿进行此操作！！！\n请确认是否继续？" ("消息")) -> (T button?=w1837:bool)  [unwired: 2 in]
            n1126 = case shown="真" w1837 {
              tunnel: w1835 -> [w1853 _]
              tunnel: w1834 -> [_ w1861]
              tunnel: w1833 -> [_ w1860]
              tunnel: [errorcluster {"status"=TRUE, "code"=0, "source"=""} ("error out") w1854] -> w1832
              frame False {
                n1127 = property class="Bool (严格)"(reference=w1853, "Value"=FALSE ("释放串口")) -> ()  [unwired: 1 in, 2 out]
              }
              frame True {
                n1128 = Bundle By Name(cluster=cluster{"命令":string} {"命令"=""} ("元素"), "命令"="CODMn程序更新" ("名称（未命名）")) -> (w1864:cluster{"命令":string})
                n1129 = Enqueue Element(queue=w1861, element=w1864, error in (no error)=w1860) -> (queue out=w1859:refnum<queue>, error out=w1858:errorcluster)  [unwired: 1 in, 1 out]
                n1130 = Bundle By Name(cluster=cluster{"命令":string} {"命令"=""} ("元素"), "命令"="停用模块" ("名称（未命名）")) -> (w1855:cluster{"命令":string})
                n1131 = Enqueue Element(queue=w1859, element=w1855, error in (no error)=w1858) -> (error out=w1854:errorcluster)  [unwired: 1 in, 2 out]
              }
            }
            n1132 = case shown="无错误" w1832 {
              frame No Error {
                n1133 = call "文件对话框"("start path"=path "D:/SRC") -> ("selected path"=w1840:path, "cancelled"=w1838:bool)  [unwired: 11 in, 2 out]
                n1134 = case shown="假" w1838 {
                  tunnel: w1840 -> [w1845 _]
                  frame False {
                    n1135 = Path To String(path=w1845) -> (string=w1842:string)
                    n1136 = Format Into String(format string="  - \"%s\"" ("格式字符串"), initial string="\"C:\\Program Files\\Fatek\\WinProladder\\WProlad.exe\"" ("command line"), w1842) -> (resulting string=w1843:string)  [unwired: 1 in, 1 out]
                    n1137 = call <vilib>:"System Exec.vi"("command line"=w1843) -> ("error out"=w1846:errorcluster)  [unwired: 7 in, 3 out]
                    n1138 = case shown="错误" w1846 {
                      tunnel: w1842 -> [_ w1849]
                      frame No Error {
                      }
                      frame Error {
                        n1139 = Format Into String(format string="  - \"%s\"" ("格式字符串"), initial string="\"C:\\Program Files (x86)\\Fatek\\WinProladder\\WProlad.exe\"" ("command line"), w1849) -> (resulting string=w1847:string)  [unwired: 1 in, 1 out]
                        n1140 = call <vilib>:"System Exec.vi"("command line"=w1847) -> ()  [unwired: 7 in, 4 out]
                      }
                    }
                  }
                  frame True {
                  }
                }
              }
              frame Error {
              }
            }
          }
        }
      }
      event "序列号变更": Value Change {
        n1141 = event-data() -> ()  [unwired: 1 in, 6 out]
        n1142 = local read "CODMn序列号"() -> (w1868:string)
        n1143 = call "序列号写入.vi"("序列号:"=w1868) -> ("确认 2"=w1865:bool, "序列号输出"=w1869:string)  [unwired: 9 in]
        n1144 = case shown="真" w1865 {
          tunnel: w1869 -> [_ w1875]
          tunnel: w1867 -> [_ w1871]
          tunnel: w1866 -> [_ w1870]
          frame False {
          }
          frame True {
            n1145 = global write "COD内部交互全局.vi" "序列号:"(w1875) -> ()
            n1146 = Bundle By Name(cluster=cluster{"命令":string} {"命令"=""} ("元素"), "命令"="CODMn序列号写入" ("名称（未命名）")) -> (w1872:cluster{"命令":string})
            n1147 = Enqueue Element(queue=w1871, element=w1872, error in (no error)=w1870) -> ()  [unwired: 1 in, 3 out]
          }
        }
      }
      event Timeout {
        n1148 = event-data() -> ()  [unwired: 1 in, 3 out]
      }
    }
  }
  n1149 = while {
    stop <- FALSE stop-if-true
    # "相差60秒自动校时"
    n1150 = global read "运行时序全局变量.vi" "多列列表框"() -> (w1877:i32)
    n1151 = local read "仪器时间"() -> (w1884:timestamp)
    n1152 = local read "系统时间"() -> (w1885:timestamp)
    n1153 = Wait (ms)(milliseconds to wait=u32 1000 ("等待时间（毫秒）")) -> ()  [unwired: 1 out]
    n1154 = Build Array(w1884) -> (w1883:timestamp[])
    n1155 = Build Array(w1885) -> (w1902:timestamp[])
    n1156 = Equal?(x=w1877, y=u16 5) -> (x = y?=w1879:bool)
    n1157 = call <vilib>:"Boolean Crossing PtByPt.vi"("direction"=enum16{"either", "false-true", "true-false"}."false-true", "input"=w1879) -> ("crossing"=w1876:bool)  [unwired: 1 in]
    n1158 = call "DateToHex.vi"("DATE"=w1883) -> ("数组"=w1896:u16[])  [unwired: 10 in]
    n1159 = call "DateToHex.vi"("DATE"=w1902) -> ("数组"=w1901:u16[])  [unwired: 10 in]
    n1160 = case shown="真" w1876 {
      frame False {
      }
      frame True {
        # "校准结束后自动更新曲线泵滴定数"
        n1161 = global read "COD测量模式全局.vi" "测量模式文字实时"() -> (w1903:string)
        n1162 = global read "COD测量模式全局.vi" "测量模式文字实时"() -> (w1908:string)
        n1163 = global read "CODMN外部API.vi" "远程反控校准CODMn"() -> (w1907:bool)
        n1164 = global read "COD内部交互全局.vi" "高锰酸钾"() -> (w1911:dbl)
        n1165 = Equal?(x=w1903, y="校零") -> (x = y?=w1904:bool)
        n1166 = Equal?(x=w1908, y="校标") -> (x = y?=w1910:bool)
        n1167 = Or(x=w1904, y=w1910) -> (x .or. y?=w1906:bool)
        n1168 = case shown="真" w1906 {
          tunnel: w1911 -> [_ w1918]
          tunnel: w1903 -> [_ w1915]
          frame False {
          }
          frame True {
            w1942 = "量程选择" ("section")
            n1169 = global read "CODMN外部API.vi" "ping"() -> (w1953:bool)
            n1170 = case shown="\"校零\"" w1915 {
              tunnel: ["标样校准时间：" "空白校准时间："] -> w1921
              frame "校标", Default {
              }
              frame "校零" {
              }
            }
            n1171 = case shown="假" w1953 {
              tunnel: [w1962 w1965] -> w1954
              frame False {
                n1172 = global read "COD内部交互全局.vi" "配置文件ini"() -> (w1964:string)
                n1173 = call <vilib>:"Application Directory.vi"() -> ("Application Directory"=w1963:path)
                n1174 = Build Path(base path=w1963, name or relative path=w1964) -> (appended path=w1962:path)
              }
              frame True {
                n1175 = global read "CODMN外部API.vi" "配置文件 path"() -> (w1965:path)
              }
            }
            n1176 = Number To Fractional String(number=w1918) -> (F-format string=w1923:string)  [unwired: 3 in]
            n1177 = call <vilib>:"Open Config Data.vi"("configuration file path"=w1954) -> ("error out"=w1941:errorcluster, "refnum"=w1940:T6)  [unwired: 8 in, 1 out]
            n1178 = Get Date/Time In Seconds() -> (seconds since 1Jan1904=w1919:timestamp)
            n1179 = Format Date/Time String(time format string (%c)="%Y/%m/%d %H:%M:%S" ("时间格式字符串(%c)"), seconds (now)=w1919) -> (date/time string=w1920:string)  [unwired: 1 in]
            n1180 = call-poly <vilib>:"Read Key.vi"("section"="标线选择", "error in (no error)"=w1941, "key"="选用水样", "refnum"=w1940) -> ("error out"=w1943:errorcluster, "value"=w1936:i32, "refnum out"=w1944:T6)  [unwired: 4 in, 1 out]
            n1181 = local write "选用水样"(w1936) -> ()
            n1182 = call-poly <vilib>:"Read Key.vi"("section"=w1942, "error in (no error)"=w1943, "key"=w1942, "refnum"=w1944) -> ("error out"=w1937:errorcluster, "value"=w1939:i32, "refnum out"=w1938:T6)  [unwired: 4 in, 1 out]
            n1183 = case shown="1" w1936 {
              tunnel: ["葡萄糖标线" ("section") "草酸钠标线" ("section")] -> w1951
              frame 0, Default {
              }
              frame 1 {
              }
            }
            n1184 = local write "量程选择"(w1939) -> ()
            n1185 = case shown="2" w1939 {
              tunnel: ["低量程" "高量程" "0-2量程"] -> w1950
              frame 0, Default {
              }
              frame 1 {
              }
              frame 2 {
              }
            }
            n1186 = Concatenate Strings(w1951, w1950) -> (w1952:string)
            n1187 = call-poly <vilib>:"Read Key.vi"("section"=w1952, "error in (no error)"=w1937, "key"="当前选用的校准" ("section"), "refnum"=w1938) -> ("error out"=w1949:errorcluster, "value"=w1914:i32, "refnum out"=w1948:T6)  [unwired: 4 in, 1 out]
            n1188 = call <vilib>:"Close Config Data.vi"("error in (no error)"=w1949, "refnum"=w1948) -> ()  [unwired: 8 in, 2 out]
            n1189 = case shown="2" w1914 {
              tunnel: [w1955 w1956 w1957 w1958 w1959] -> w1913
              frame 1, Default {
                n1190 = local read "浓度1"() -> (w1955:dbl)
              }
              frame 2 {
                n1191 = local read "浓度2"() -> (w1956:dbl)
              }
              frame 3 {
                n1192 = local read "浓度3"() -> (w1957:dbl)
              }
              frame 4 {
                n1193 = local read "浓度4"() -> (w1958:dbl)
              }
              frame 5 {
                n1194 = local read "浓度5"() -> (w1959:dbl)
              }
            }
            n1195 = Number To Fractional String(number=w1913) -> (F-format string=w1925:string)  [unwired: 3 in]
            n1196 = Concatenate Strings("信息：校准结果：\n", "校准浓度：", w1925, "滴定数：", w1923, w1921, w1920) -> (w1917:string)
            n1197 = Bundle(cluster=T14 {"时间标识"=timestamp(0 s since 1904-01-01), "参数"="", "日志信息"="", "流程参数"=""} ("data in"), "时间标识"=w1919, "参数"="CODMn" ("table输入"), "日志信息"=w1917, "流程参数"="" ("table输入")) -> (w1929:T14)
            n1198 = call "流程日志字段定义.vi"("table输入"="校准记录", "data in"=w1929) -> ("table输出"=w1933:string, "columns"=w1934:string[], "data out"=w1935:T17)  [unwired: 7 in]
            n1199 = call "插入数据.vi"("data"=w1935, "columns"=w1934, "database"="database3.mdb", "table"=w1933) -> ()  [unwired: 7 in, 1 out]
            n1200 = global write "COD内部交互全局.vi" "当前校准"(w1914) -> ()
            n1201 = case shown="1, 默认" w1914 {
              tunnel: w1918 -> [w1971 w1972 w1973 w1974 w1975]
              frame 1, Default {
                n1202 = property on="泵滴定数1" class="DigNum (严格)"("Val(Sgnl)"=w1971) -> ()  [unwired: 2 in, 2 out]
              }
              frame 2 {
                n1203 = property on="泵滴定数2" class="DigNum (严格)"("Val(Sgnl)"=w1972) -> ()  [unwired: 2 in, 2 out]
              }
              frame 3 {
                n1204 = property on="泵滴定数3" class="DigNum (严格)"("Val(Sgnl)"=w1973) -> ()  [unwired: 2 in, 2 out]
              }
              frame 4 {
                n1205 = property on="泵滴定数4" class="DigNum (严格)"("Val(Sgnl)"=w1974) -> ()  [unwired: 2 in, 2 out]
              }
              frame 5 {
                n1206 = property on="泵滴定数5" class="DigNum (严格)"("Val(Sgnl)"=w1975) -> ()  [unwired: 2 in, 2 out]
              }
            }
          }
        }
        n1207 = case shown="真" w1907 {
          frame False {
          }
          frame True {
            # "校准完自动写入公式"
            n1208 = global write "CODMN外部API.vi" "远程反控校准CODMn"(FALSE ("远程反控校准CODMn")) -> ()
          }
        }
      }
    }
    n1209 = Index Array(array=w1896, index=2 ("索引")) -> (element=w1898:u16)
    n1210 = Index Array(array=w1901, index=2 ("索引")) -> (element=w1899:u16)
    n1211 = Split Number(x=w1898) -> (hi(x)=w1892:u8)  [unwired: 1 out]
    n1212 = Split Number(x=w1899) -> (hi(x)=w1895:u8)  [unwired: 1 out]
    n1213 = To Byte Integer(number=w1892) -> (8bit integer=w1891:i8)
    n1214 = To Byte Integer(number=w1895) -> (8bit integer=w1894:i8)
    n1215 = Subtract(x=w1891, y=w1894) -> (x-y=w1893:i8)
    n1216 = Absolute Value(x=w1893) -> (abs(x)=w1890:i8)
    n1217 = local read "通讯状态"() -> (w1887:bool)
    n1218 = Greater Or Equal?(x=w1890, y=i8 5) -> (x >= y?=w1888:bool)
    n1219 = And(x=w1888, y=w1887) -> (x .and. y?=w1886:bool)
    n1220 = case shown="真" w1886 {
      frame False {
      }
      frame True {
        # "相差60秒时间自动校准"
        n1221 = flat-sequence {
          frame #0 {
            n1222 = property on="时间校准" class="Bool (严格)"("Val(Sgnl)"=TRUE ("值(信号)")) -> ()  [unwired: 2 in, 2 out]
          }
          frame #1 {
            n1223 = Wait (ms)(milliseconds to wait=u32 500 ("等待时间（毫秒）")) -> ()  [unwired: 1 out]
          }
          frame #2 {
            n1224 = property on="时间校准" class="Bool (严格)"("Val(Sgnl)"=FALSE ("值(信号)")) -> ()  [unwired: 2 in, 2 out]
          }
        }
      }
    }
  }
  n1225 = while {
    stop <- FALSE stop-if-true
    n1226 = global read "COD内部交互全局.vi" "待机"() -> (w1980:bool)
    n1227 = Wait (ms)(milliseconds to wait=u32 1000 ("等待时间（毫秒）")) -> ()  [unwired: 1 out]
    n1228 = case shown="假" w1980 {
      tunnel: [w1997 T9."Enabled" ("禁用")] -> w1982
      tunnel: [w1996 _] -> w1981
      frame False {
        # "运行中"
        n1229 = local read "校标标记"() -> (w1995:bool)
        n1230 = local read "校零标记"() -> (w1994:bool)
        n1231 = Or(x=w1995, y=w1994) -> (x .or. y?=w1998:bool)
        n1232 = case shown="真" w1998 {
          tunnel: [T9."Enabled" ("禁用") T9."Disabled and Grayed Out" ("禁用")] -> w1997
          tunnel: [_ TRUE] -> w1996
          frame False {
          }
          frame True {
          }
        }
      }
      frame True {
      }
    }
    n1233 = control-ref of="量程选择"() -> (w1988:refnum<vi>)
    n1234 = property on="校准内容显示" class="Str"("Visible"=w1981) -> ()  [unwired: 2 in, 2 out]
    n1235 = control-ref of="选用水样"() -> (w1989:refnum<vi>)
    n1236 = control-ref of="校准5"() -> (w1983:refnum<vi>)
    n1237 = control-ref of="校准4"() -> (w1984:refnum<vi>)
    n1238 = control-ref of="校准3"() -> (w1985:refnum<vi>)
    n1239 = control-ref of="校准2"() -> (w1986:refnum<vi>)
    n1240 = control-ref of="校准1"() -> (w1987:refnum<vi>)
    n1241 = Build Array(w1983, w1984, w1985, w1986, w1987, w1989, w1988) -> (w1990:refnum<vi>[])
    n1242 = for {
      tunnel: w1990 -> [w1993] mode=indexing
      tunnel: w1982 -> [w1992]
      n1243 = property class="Ctl"(reference=w1993, "DisabledEnum"=w1992) -> ()  [unwired: 1 in, 2 out]
    }
  }
  n1244 = while {
    stop <- FALSE stop-if-true
    # "滚动显示"
    n1245 = global read "COD内部交互全局.vi" "待机"() -> (w2003:bool)
    n1246 = case shown="假" w2003 {
      frame False {
        # "运行中"
        n1247 = global read "COD内部交互全局.vi" "校准内容显示"() -> (w2006:string)
        n1248 = while {
          shift-right: [w2008] -> _
          shift-left: w2006 -> [w2013]
          stop <- w2007 stop-if-true
          (unwired) "仪器校准中!\n当前校准浓度为:3mg/L" ("校准内容显示")
          n1249 = Wait (ms)(milliseconds to wait=u32 500 ("等待时间（毫秒）")) -> ()  [unwired: 1 out]
          n1250 = Spreadsheet String To Array(delimiter (Tab)="\n" ("分隔符(Tab)"), format string="" ("格式字符串"), spreadsheet string=w2013, array type (2D Dbl)=string[] []) -> (array=w2016:string[])
          n1251 = for {
            tunnel: w2016 -> [w2024] mode=indexing
            tunnel: [w2022] -> _ mode=indexing
            shift-right: [w2020] -> w2011
            shift-left: "" ("格式字符串") -> [w2021]
            n1252 = call "字符串移位显示.vi"("字符框大小"=36, "字符串输入"=w2024) -> ("移位后字符串"=w2022:string)  [unwired: 8 in, 1 out]
            n1253 = Concatenate Strings(w2021, w2022, "\n" ("分隔符(Tab)")) -> (w2020:string)
          }
          n1254 = String Length(string=w2011) -> (length=w2010:i32)
          n1255 = Decrement(x=w2010) -> (x-1=w2009:i32)
          n1256 = String Subset(string=w2011, length (rest)=w2009) -> (substring=w2008:string)  [unwired: 1 in]
          "校准内容显示" <- w2008
          n1257 = global read "COD内部交互全局.vi" "待机"() -> (w2007:bool)
        }
      }
      frame True {
      }
    }
    n1258 = Wait (ms)(milliseconds to wait=u32 1000 ("等待时间（毫秒）")) -> ()  [unwired: 1 out]
  }
  n1259 = while {
    stop <- FALSE stop-if-true
    w2058 = T18 0 items=["最小二乘", "最小绝对残差", "Bisquare"] ("method")
    # "计算线性、多项式公式、远程校准"
    n1260 = local read "浓度1"() -> (w2031:dbl)
    n1261 = local read "浓度2"() -> (w2060:dbl)
    n1262 = local read "浓度3"() -> (w2061:dbl)
    n1263 = local read "浓度4"() -> (w2053:dbl)
    n1264 = local read "浓度5"() -> (w2052:dbl)
    n1265 = Build Array("泵滴定数1", "泵滴定数2", "泵滴定数3", "泵滴定数4", "泵滴定数5") -> (w2059:dbl[])
    n1266 = Build Array(w2031, w2060, w2061, w2053, w2052) -> (w2027:dbl[])
    n1267 = Build Array("启用1", "启用2", "启用3", "启用4", "启用5") -> (w2030:bool[])
    n1268 = global read "CODMN外部API.vi" "远程反控校准CODMn"() -> (w2028:bool)
    n1269 = call "将启用的浓度作为新的浓度数组.vi"("启用布尔数组"=w2030, "输入浓度数组"=w2027) -> ("启用的浓度数组"=w2029:dbl[])  [unwired: 13 in]
    n1270 = Unbundle By Name("方程系数") -> ("K"=w2039:dbl, "b"=w2038:dbl, "X^2"=w2037:dbl)
    n1271 = case shown="\"多项式\"" "模型" {
      tunnel: w2039 -> [w2070 w2073]
      tunnel: w2038 -> [w2069 w2074]
      tunnel: w2037 -> [_ w2072]
      frame "线性", Default {
        "K" <- w2070
        "b" <- w2069
      }
      frame "多项式" {
        n1272 = Build Array(w2074, w2073, w2072) -> (→"多项式系数":dbl[])
      }
    }
    n1273 = call "线性公式CODMn用.vi"("标液浓度"=w2027, "监测浓度"=w2059, "启用"=w2030, "method"=w2058, "模型"="模型", "精度"=6) -> ("拟合方程"=w2045:string, "r^2"=→"r^2":dbl, "slope"=w2043:dbl, "intercept"=w2044:dbl, "XY图"=→"XY图":cluster{"X Values":dbl[], "Y Values":dbl[]}[], "Polynomial Coefficients"=w2054:dbl[])  [unwired: 8 in]
    "拟合公式" <- w2045
    n1274 = call <vilib>:"Boolean Crossing PtByPt.vi"("direction"=enum16{"either", "false-true", "true-false"}."false-true", "input"=w2028) -> ("crossing"=w2026:bool)  [unwired: 1 in]
    n1275 = case shown="真" w2026 {
      tunnel: w2027 -> [_ w2064]
      frame False {
      }
      frame True {
        n1276 = global read "CODMn断电保存全局变量.vi" "远程自动校准浓度"() -> (w2065:dbl)
        n1277 = Search 1D Array(1D array=w2064, element=w2065) -> (index of element=w2066:i32)  [unwired: 1 in]
        n1278 = case shown="0, 默认" w2066 {
          selector: w2066 -> [_ w2068]
          frame -1 {
          }
          frame 0, Default {
            n1279 = Increment(x=w2068) -> (x+1=w2067:i32)
            n1280 = global write "COD内部交互全局.vi" "当前校准"(w2067) -> ()
          }
        }
      }
    }
    n1281 = feedback #3(w2045) -> (w2046:string)
    n1282 = feedback-in #3(w2045) -> ()
    n1283 = Not Equal?(x=w2045, y=w2046) -> (x != y?=w2042:bool)
    n1284 = global write "COD内部交互全局.vi" "启用的浓度数组"(w2029) -> ()
    n1285 = case shown="真" w2042 {
      tunnel: w2054 -> [_ w2078]
      tunnel: w2044 -> [_ w2079]
      tunnel: w2043 -> [_ w2080]
      frame False {
      }
      frame True {
        # "当公式发生改变时赋值到右侧公式"
        n1286 = local read "模型"() -> (w2081:enum32{"线性", "多项式"})
        n1287 = case shown="\"多项式\"" w2081 {
          tunnel: [w2086 w2088] -> w2076
          tunnel: w2080 -> [w2086 _]
          tunnel: w2079 -> [w2085 _]
          tunnel: [w2085 w2089] -> w2077
          tunnel: w2078 -> [_ w2090]
          tunnel: [0.0 ("数值") w2087] -> w2075
          frame "线性", Default {
          }
          frame "多项式" {
            # "B,K,X^2"
            n1288 = Index Array(array=w2090) -> (element #1=w2089:dbl, element #2=w2088:dbl, element #3=w2087:dbl)  [unwired: 3 in]
          }
        }
        n1289 = Bundle By Name(cluster=cluster{"K":dbl, "b":dbl, "X^2":dbl} {"K"=0.0, "b"=0.0, "X^2"=0.0} ("方程系数"), "K"=w2076, "b"=w2077, "X^2"=w2075) -> (w2082:cluster{"K":dbl, "b":dbl, "X^2":dbl})
        n1290 = local write "方程系数"(w2082) -> ()
      }
    }
    n1291 = Wait (ms)(milliseconds to wait=u32 1000 ("等待时间（毫秒）")) -> ()  [unwired: 1 out]
  }
  n1292 = property class="VI"(reference=w6, error in=w3) -> ("Name"=w7:string)  [unwired: 2 out]
  n1293 = Open VI Reference(type specifier VI Refnum (for type only)=refnum<vi> refnum, vi path=w7, options=128 ("选项")) -> (vi reference=w9:refnum<vi>, error out=w11:errorcluster)  [unwired: 3 in]
  n1294 = call-by-ref "?"(reference=w9, error in=w11) -> (reference out=w13:refnum<vi>, error out=w12:errorcluster)  [unwired: 12 in]
  n1295 = Close Reference(reference=w13, error in (no error)=w12) -> ()  [unwired: 1 out]
